vi "IonicsServiceTool.vi"() -> ()   [LabVIEW 2018]
uses:
  Type/_Source Type.ctl
  Type/_Syringe Pump Command.ctl
  Type/_Instrument Model.ctl
  Type/_RT Instrument State.ctl
  Type/_Run State.ctl
  Type/_Log Command.ctl
  Type/_RT Command.ctl
  Type/_RT Configuration 2.ctl
  Type/_PIC Channel.ctl
  Type/_RT Startup Options.ctl
  Type/_RT Instrument 2.ctl
  Type/_Data Operation.ctl
  Type/_Model Family.ctl
  Type/_SaveOption.ctl
  Type/_Board ID.ctl
  Type/_Run Module.ctl
  Type/_Voltage Type.ctl
  Print.ctl
  Type/_Pump Parameter.ctl
  Configuration/_Global Configuration.vi
  <vilib>/Utility/config.llb/Read Key (Path).vi
  <vilib>/Utility/config.llb/Write Key (Path).vi
  <vilib>/Utility/config.llb/Read Key (String).vi
  <vilib>/Utility/config.llb/Write Key (String).vi
  LCDriver/_Global LC Driver.vi
  <vilib>/Utility/config.llb/Read Key (I32).vi
  <vilib>/Utility/NIReport.llb/Append Image to Report (path wrap).vi
  <vilib>/Platform/browser.llb/Open URL in Default Browser (string).vi
  <vilib>/Utility/config.llb/Write Key (I32).vi
  <vilib>/Utility/NIReport.llb/NI_report.lvclass
  <vilib>/Utility/config.llb/NI_LVConfig.lvlib
panel:
  in  "Force Update Oscillators":bool
  out "Version":string
  out "Date/Time":string
  out "SN":string
  in  "Force Update Poles":bool
  out "MS State":T1
  in  "Print":bool
  in  "Options":bool
  in  "Unit":bool
  out "Firmware OK":bool
  out "Intlk/Per OK":bool
  out "Quad/Tune OK":bool=TRUE
  out "SVG OK":bool
  out "Voltage OK":bool
  out "Turbo OK":bool
  in  "Tab Control":T2(tab)
  out "*.ipf Path:":path=path "C:/GIT/EH-Simplicity/firmware-server/Sniffer.900/Ionica Server.ipf"
  in  "Header Info":bool
  out "IP Address":string="172.16.0.2"
  out "Corona":u16
  out "Source 2":u16
  out "Source 1":u16
  out "HSID":u16
  out "Model Name":T3=enum."Simulation (Single Source)"
  out "Serial Number":string="Ion Sniffer 03"
  in  "Refresh":bool
  out "Messages":string
  out "Description":string
  in  "Load Firmware":bool
  out "Current Information:":string[][](table)=[["FW Package Version", "0"], ["RT Firmware Version", "0"], ["FPGA Firmware Version", "0"], ["", ""], ["Instrument Serial #", "-1"], ["Instrument Model", "-1"]]
  out "Number of Power Failures:":u32
  out "Number of Pressure Overload Errors:":u32
  out "Total Number of Errors:":u32
  out "Errors:":string[][](table)=[["0", ""], ["", ""], ["", ""], ["", ""], ["", ""], ["", ""], ["", ""], ["", ""]]
  out "PumpStatus":u16(ring)
  out "Turning":bool
  out "Normal \nOperation":bool
  out "Accel":bool
  out "Decel":bool
  out "Frequency (Hz):":u16(slide) scale=0.0..1000.0
  out "Controller Temperature:":u16(slide) scale=0.0..90.0
  out "Moter Temperature:":u32(slide) scale=0.0..120.0
  out "Bearing Temperature:":u32(slide) scale=0.0..75.0
  out "Pressures:":string[][](table)=[["Foreline Pressure (torr)", "-0.11"], ["Analyzer Pressure (torr)", "1.00E+0"]]
  out "Run Time:":string[][](table)=[["Pump (hours)", ""], ["Days", ""], ["Number of Starts", ""], ["", ""], ["", ""], ["", ""], ["", ""], ["", ""]]
  out "Power:":string[][](table)=[["Voltage (V)", ""], ["Power (W)", ""], ["Current (A)", ""], ["Mean Current (A)", ""], ["Max Current (A)", ""], ["", ""], ["", ""], ["", ""]]
  out "Configuration:":string[][](table)=[["Pump Model", ""], ["Pump Serial Number", ""], ["Controller Model", ""], ["Controller Serial Number", ""], ["Electronics Model", ""], ["Electronic Serial Number", ""], ["Software Version", ""], ["Pump Parameter Set", ""]]
  in  "LBPower":bool
  in  "LBRunTime":bool
  in  "LBError":bool
  in  "LBConfiguration":bool
  in  "LBFreqTemp":bool
  in  "LBUpdateAll":bool
  in  "LBPump":bool
  in  "Update Power":bool
  in  "Update Temp":bool
  in  "Update Pumping":bool
  in  "Update Info":bool
  out "Error History":string[][](table)
  out "Temperatures:":string[][](table)=[["Electronic Drive Temperature", "Pass"], ["Pump Temperature", "Pass"], ["Power Stage Temperature (°C)", "0"], ["Electronics Temperature (°C)", "0"], ["Upper Pump Temperature (°C)", "0"], ["Bearing Temperature (°C)", "0"], ["Motor Temperature (°C)", "0"]]
  out "Power / Current:":string[][](table)=[["Drive Power (W)", "0"], ["Drive Current (A)", "0"]]
  out "Pumping:":string[][](table)=[["Rotational Frequency (Hz)", "0"], ["Rotational Speed (rpm)", "0"]]
  out "Pump Info:":string[][](table)=[["Hardware Version", "0"], ["Firmware Version", "0"], ["Operating Hours (Pump)", "0"], ["Operating Hours (Electronic Drive)", "0"]]
  in  "Turbo Update":bool
  out "Vacuum Readings by Region":string[][](table)=[["Foreline Pressure (torr)", "-0.11"], ["Analyzer Pressure (torr)", "1.00E+0"]]
  in  "Update Error":bool
  out "Main System Current (A)":dbl
  out "Lens Board 2 PS":i32(listbox)=-1
  in  "Set 0 Values":bool
  in  "Load Default Method":bool
  in  "Load Tune File":bool
  in  "Min Voltages":bool
  in  "Max Voltages":bool
  in  "Test Voltages":bool
  in  "Switch Polarity":bool
  out "Main System PS":i32(listbox)=-1
  out "Quad DC PS":i32(listbox)=-1
  out "Lens Board 1 PS":i32(listbox)=-1
  in  "Detector":string[][](table)=[["HED", "", "0.0", "3.014"], ["Horn", "", "0.0", "0.019"], ["DV", "", "0.0", "0.023"], ["Disc", "", "0.0", "2.014"], ["5", "L2 (11)", "0.0", "0.019"], ["6", "PF (12)", "-16.0", "0.019"], ["7", "CCL1 (13)", "0.0", "0.019"], ["8", "CCL2 (14)", "-100.0", "0.019"], ["9", "CC (23)", "-50.0", "0.014"], ["10", "CCAF (10)", "50.0", "0.019"], ["11", "CCL3 (15)", "-52.5", "0.014"], ["12", "CCL4 (16)", "-72.5", "0.014"], ["13", "ID (17)", "-100.0", "0.014"], ["14", "Horn (200)", "5500.0", "-82.090"], ["15", "DV (34)", "1000.0", "-82.773"], ["16", "M1RF (3)", "400.0", "2.161"], ["17", "Disc (32)", "10", "10"]]
  in  "Lens 1":string[][](table)=[["Element", "L1", "M1", "EV", "Spare", "M2", "CC", "Spare", "Spare"], ["Input", "0", "0", "0", "0", "0", "0", "0", "0"], ["Readback", "0", "0", "0", "0", "0", "0", "0", "0"]]
  in  "Lens 2":string[][](table)=[["Element", "CCAF", "L2", "PF", "CCL1", "CCL2", "CCL3", "CCL4", "ID"], ["Input", "", "", "", "", "", "", "", ""], ["Readback", "", "", "", "", "", "", "", ""]]
  out "Source Map":T4={"Ring 2"=0, "Ring 3"=0, "OK 2"=TRUE, "OK 3"=TRUE, "OK 4"=TRUE, "OK 5"=TRUE, "OK 6"=TRUE, "OK 7"=TRUE, "OK 8"=TRUE, "OK 9"=TRUE, "OK 10"=TRUE, "OK 11"=TRUE}
  out "Pressure Readings":string[][](table)=[["Foreline Pressure (torr)", "-0.11"], ["Analyzer Pressure (torr)", "1.00E+0"], ["Plenum Delta P (torr)", "-0.09"], ["Drying Gas Pressure (psi)", "-12.56"], ["Source Gas Pressure (psi)", "-12.56"]]
  in  "Corona/Curtain High Voltage":string[][](table)=[["Corona High Voltage", "0.0", "65535.000", "0"], ["Curtain Cap Voltage", "0.0", "910936.500", "0"]]
  in  "Source Probes":string[][](table)=[["Pillar 1", "None", "0.0", "2791790.869", "0"], ["Pillar 2", "None", "0.0", "2794412.334", "0"]]
  in  "Heaters":string[][](table)=[["1", "HSID", "200.0", "65535.000"], ["2", "P1T", "0.0", "93715.050"], ["3", "P2T", "0.0", "93715.050"]]
  in  "Typical Gas Settings":bool
  in  "Max Gas Settings":bool
  in  "Min Gas Settings":bool
  in  "Gas Flows":string[][](table)=[["1", "DG", "150.0", "316.460"], ["2", "NG1", "200.0", "312.782"], ["3", "HG1", "280.0", "354.817"], ["4", "NG2", "200.0", "0.000"], ["5", "HG2", "280.0", "0.000"], ["6", "CCP", "490", "-477.539"]]
  in  "GotoUPS":bool
  in  "IP Address":string
  in  "Input Value":sgl
  in  "Pump Command":T5=enum."status"
  out "Return Data":string
  in  "SendSyringeCommand":bool
  out "SourceOK":bool
  out "HG2OK":bool
  out "HG1OK":bool
  out "ExhaustOK":bool
  out "DryingGasOK":bool
  out "VacRdy":bool
  out "DoorOK":bool=TRUE
  out "Interlocks":string[][](table)=[["Card Cage Door", ""], ["Vacuum Ready", ""], ["Heating Gas 1", ""], ["Heating Gas 2", ""], ["Drying Gas", ""], ["Exhaust Gas", ""], ["Source Interlock", ""]]
  out "Source 2 Type:":T6=127 items=["None", "ESI", "APCI", "APPI", "MicroSpray"]
  out "Source 1 Type:":T6=127 items=["None", "ESI", "APCI", "APPI", "MicroSpray"]
  in  "FrequencyTuneSetup":bool
  out "Q2 RF Heat Sink Temperatures":string[][](table)=[["Q2 HS1", "-0.481"], ["Q2 HS2", "-0.481"], ["Q2 DC Pole A (18)", "-0.481"], ["Q2 DC Pole B (19)", "-0.481"]]
  out "Q1 RF Heat Sink Temperatures":string[][](table)=[["Q1 HS1", "-0.481"], ["Q1 HS2", "-0.481"], ["Q2 DC Pole A (18)", "-0.481"], ["Q2 DC Pole B (19)", "-0.481"]]
  out "M1 RF Heat Sink Temperatures":string[][](table)=[["M1 HS1", "-0.481"], ["M1 HS2", "-0.481"], ["Q2 DC Pole A (18)", "-0.481"], ["Q2 DC Pole B (19)", "-0.481"]]
  out "New Frequence":dbl=1.1064999969676137 format="%.4f"
  out "Old Frequency":dbl=1.1064999969676137 format="%.4f"
  in  "Adjust Cal Tables":bool
  out "M1RF Readback":dbl
  in  "M1RF":dbl=400.0 format="%#.3f"
  in  "Update PM":bool
  in  "Q2 Park Mass":dbl=400.0 format="%#.3f"
  in  "Q1 Park Mass":dbl=400.0 format="%#.3f"
  out "Q2 Total":dbl=157.94015025000002
  out "Q1 Total":dbl=157.94015025000002
  out "Q2 (VDC)":dbl=157.94015025000002
  out "Q1 (VDC)":dbl=157.94015025000002
  in  "Q2 DC Inputs":string[][](table)=[["600.00"], ["0.00"], ["0.00"]]
  in  "Q1 DC Inputs":string[][](table)=[["600.00"], ["0.00"], ["0.00"]]
  out "DC Pole Read Back":string[][](table)=[["Q1 DC Pole A", "-0.481"], ["Q1 DC Pole B", "-0.481"], ["Q2 DC Pole A", "-0.481"], ["Q2 DC Pole B", "-0.481"]]
  in  "Oscillator Settings":string[][](table)=[["M1RF", "66529043", "10", "10", "0.4", "1.5490", "2.256", "1.5490"], ["Q1RF", "47523813", "10", "10", "0.6", "1.1065", "-0.645", "1.1065"], ["Q2RF", "47523813", "10", "10", "0.6", "1.1065", "7.339", "1.1065"]]
  in  "Pos/Neg":enum32{"Positive", "Negative"}(radio)
  in  "Pole Swap Options Negative":T7
  in  "Pole Swap Options Positive":T7
  in  "Table Choice":T8(radio)
  out "Table 4":T9 caption="Q2 -ve Mass Calibration Table"
  out "Table 2":T9 caption="Q2 +ve Mass Calibration Table"
  out "Table 3":T9 caption="Q1 -ve Mass Calibration Table"
  out "Table 1":T9 caption="Q1 +ve Mass Calibration Table"
  in  "Edit Config":bool
  in  "Edit ADC":bool
  in  "View Config":bool
  in  "Export ADC":bool
  out "ADC List":i32(listbox)=130
  in  "Run":bool
  in  "Cancel":bool
  out "Progress Bar":u8(slide)=1 scale=0.0..100.0
  out "LoadedTable":bool
  in  "Tune File":path=path "C:/GIT/EH-Simplicity/firmware-server/Sniffer.900/InternalTools/DEFAULT_SETTINGS.d2m"
  in  "SG Input":dbl[](array[numeric])=[40.0, 0.0, 0.0, 0.0, 0.0, 0.0, 0.0, 200.0, 0.0, 0.0, 0.0, 0.0, 0.0, 0.0]
  in  "VoltageInput":dbl[](array[numeric])=[0.0, 0.0, 0.0, 0.0, 0.0, -16.0, 0.0, -100.0, -50.0, 50.0, -52.5, -72.5, -100.0, 5500.0, 1000.0, 400.0, 10.0, 0.0, 0.0]
  out "Quit":bool=TRUE
  out "Running":bool
  out "Ion Path":T10={"OK 1"=TRUE, "OK 2"=TRUE, "OK 3"=TRUE, "OK 4"=TRUE, "OK 5"=TRUE, "OK 6"=TRUE, "OK 7"=TRUE, "OK 8"=TRUE, "OK 9"=TRUE, "OK 10"=TRUE, "OK 15"=TRUE, "OK 20"=TRUE, "OK 16"=TRUE, "OK 11"=TRUE, "OK 17"=TRUE, "OK 18"=TRUE, "OK 19"=TRUE, "OK 12"=TRUE, "OK 13"=TRUE, "Selected 1"="Selected", "Selected 2"="Selected", "Selected 3"="Selected", "Selected 4"="Selected", "Selected 5"="Selected", "Selected 6"="Selected", "Selected 7"="Selected", "Selected 8"="Selected", "Selected 9"="Selected", "Selected 10"="Selected", "Selected 15"="Selected", "Selected 20"="Selected", "Selected 16"="Selected", "Selected 11"="Selected", "Selected 17"="Selected", "Selected 18"="Selected", "Selected 19"="Selected", "Selected 12"="Selected", "Selected 13"="Selected", "Ring 2"=0, "Ring 3"=0, "OK 14"=TRUE, "Selected 14"="Selected"}
  out "IonPathMap":enum32{"0", "200", "100"}(tab)
  # "PIC Firmware Version"
  # "It will take about 70s\nto complete Update All."
  # "Syringe Pump Control"
  # "UPS"
  # "V"
  # "Polarity"
  # "Pole Orientation"
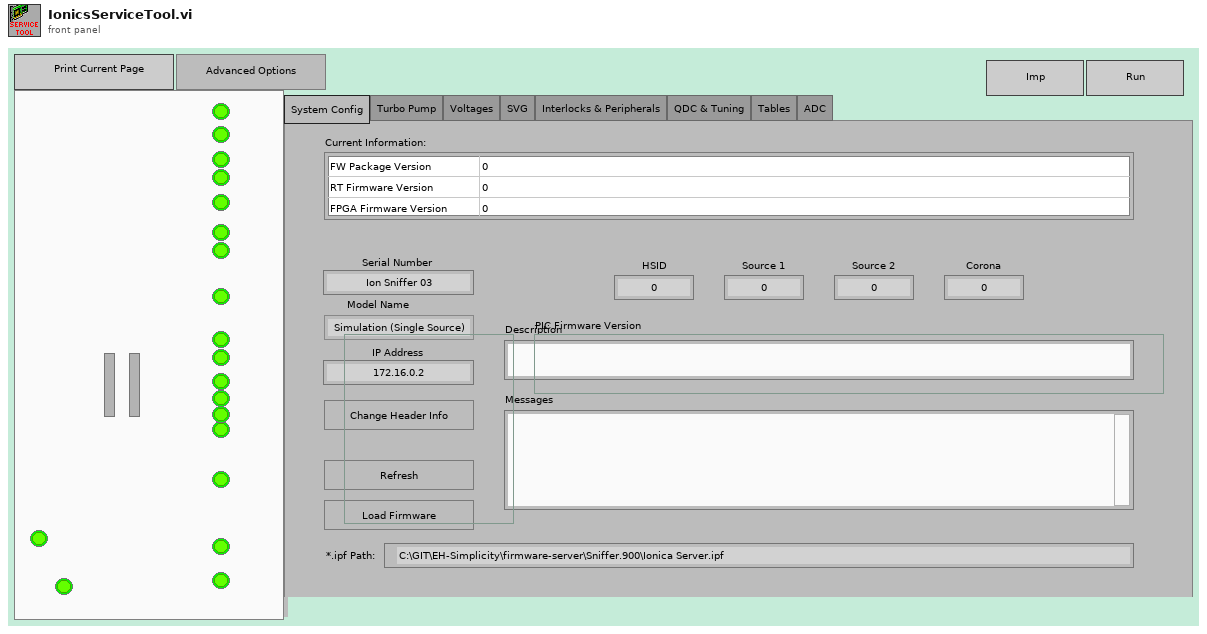
[diagram p1: front panel]
types:
  T1 = typedef "_RT Instrument State.ctl" = enum16{"Initializing", "Mass Spectrometer is Off", "Starting Up", "Turning Power Off", "Going to Standby", "Roughing Pump Ready", "Turning Turbo Off", "Turbo Startup", "Turbopump Ready", "Checking Vacuum", "Going to Ready", "Ready", "Running", "Source Standby", "Lost Communication", "Shutting Down", "Fault", "24V Standby", "Go to 24V Standby", "Turbopump Ready-Waiting"}
  T2 = enum32{"System Config", "Leybold 3QS", "Turbo Pump", "Voltages", "SVG", "Interlocks & Peripherals", "QDC & Tuning", "Tables", "ADC"}
  T3 = typedef "_Instrument Model.ctl" = enum16{"QSight 110", "QSight 120", "QSight 210", "QSight 220", "QSight 410", "QSight 420", "IONICS 3Q 110", "IONICS 3Q 120", "IONICS 3Q 210", "IONICS 3Q 220", "IONICS 3Q 310", "IONICS 3Q 320", "Simulation (Single Source)", "Simulation (Dual Source)"}
  T4 = cluster{"Ring 2":u16, "Ring 3":u16, "OK 2":bool, "OK 3":bool, "OK 4":bool, "OK 5":bool, "OK 6":bool, "OK 7":bool, "OK 8":bool, "OK 9":bool, "OK 10":bool, "OK 11":bool}
  T5 = typedef "_Syringe Pump Command.ctl" = enum16{"start", "stop", "pause", "restart", "help", "set units", "set diameter", "set rate", "set time", "set volume", "set delay", "save setting", "read limit parameter", "view parameter", "status"}
  T6 = typedef "_Source Type.ctl" = i8
  T7 = cluster{"Q1 A":bool, "Q1 B":bool, "Q2 A":bool, "Q2 B":bool}
  T8 = enum32{"Calibration", "Low Resolution", "Unit Resolution", "High Resolution"}
  T9 = cluster{"Graph":cluster{"all rows":dbl[], "all rows":dbl[]}, "Table":string[][]}
  T10 = cluster{"OK 1":bool, "OK 2":bool, "OK 3":bool, "OK 4":bool, "OK 5":bool, "OK 6":bool, "OK 7":bool, "OK 8":bool, "OK 9":bool, "OK 10":bool, "OK 15":bool, "OK 20":bool, "OK 16":bool, "OK 11":bool, "OK 17":bool, "OK 18":bool, "OK 19":bool, "OK 12":bool, "OK 13":bool, "Selected 1":string, "Selected 2":string, "Selected 3":string, "Selected 4":string, "Selected 5":string, "Selected 6":string, "Selected 7":string, "Selected 8":string, "Selected 9":string, "Selected 10":string, "Selected 15":string, "Selected 20":string, "Selected 16":string, "Selected 11":string, "Selected 17":string, "Selected 18":string, "Selected 19":string, "Selected 12":string, "Selected 13":string, "Ring 2":u16, "Ring 3":u16, "OK 14":bool, "Selected 14":string}
  T11 = enum32{"invalid app kind", "Development System", "Run Time System", "Student Edition", "Embedded LabVIEW", "Evaluation", "Custom"}
  T12 = enum8{"Enabled", "Disabled", "Disabled and Grayed Out"}
  T13 = typedef "_Run State.ctl" = enum16{"Init", "Update", "Start", "End", "Error"}
  T14 = typedef "_Log Command.ctl" = enum16{"No Command", "Open", "Read", "Write", "Close", "Check Size"}
  T15 = typedef "_RT Command.ctl" = enum16{"xml Start Run", "xml Start Actual Run", "xml Stop Run", "xml Runtime Update", "xml Get Status", "xml Get Table", "xml Set Table", "xml Get Configuration", "xml System Status", "xml Set LC Input Logic", "xml Get Data", "xml Get Info", "Start", "StartActualRun", "Stop", "Runtime Update", "Get Data", "Get Info", "Get Status", "Get Param", "Get Config", "Get Table", "Read ADC", "Set Oscillator", "Update Config", "Update Table", "Set All Pol", "Set Pol and DC", "Set Max Mass", "Toggle RP", "Toggle EL", "Set PIC", "Initialize Turbo", "Send Turbo Comm", "Close Turbo", "P1", "P2", "P3", "Send Serial", "Set LC Out", "Get LC In", "Read VAC", "Test Table", "Toggle Power", "Get Startup", "Set Startup", "Get ADC Table", "Set ADC Table", "Get Brief Status", "Get Detail Status", "Auxiliary Update", "Set CC Logics", "Test Channel", "Set CC Input Logics", "Ignore Error", "invalid"}
  T16 = enum16{"Use Dialog", "Temporary File", "My Tables"}
  T17 = typedef "_PIC Channel.ctl" = enum16{"Corona +HV", "Corona -HV", "HSID Temp", "Time Const 1", "Curtain Cap +HV", "Curtain Cap -HV", "Time Const 2", "Source 1 +HV", "Source 1 -HV", "Source 1 Temp", "Time Const 3", "Source 2 +HV", "Source 2 -HV", "Source 2 Temp", "Time Const 4"}
  T18 = typedef "_RT Instrument 2.ctl" = cluster{"Table":T19[], "Instrument":string[]}
  T19 = typedef "_RT Configuration 2.ctl" = cluster{"Name":string, "Ch#":u8, "Min":dbl, "Max":dbl, "Def+":dbl, "Def-":dbl, "Offset":dbl, "Slope":dbl, "Type":u8, "Description":string, "SettleT":dbl}
  T20 = cluster{"top":dbl, "left":dbl, "right":dbl, "bottom":dbl}
  T21 = typedef "Print.ctl" = cluster{"Picture Name":string, "VI Reference":refnum<vi>}
  T22 = enum16{"Standard Report", "HTML", "Word", "Excel"}
  T23 = typedef "_Data Operation.ctl" = enum8{"Initialize", "Get Data", "Set Data", "Close"}
  T24 = typedef "_SaveOption.ctl" = enum16{"Use Dialog", "Temporary File", "My Tables", "Full Path"}
  T25 = typedef "_Pump Parameter.ctl" = enum16{"Turn Pump Motor On", "Turn Pump Motor Off", "Read Pump Oil Deficiency", "Read Rotation Switch Point Attained", "Read Ele. Drive Over Temperature", "Read Pump Over Temperature", "Read Set Rotation Speed Attained", "Read Turbopump Accelerates", "Read Actual Rotation Speed in Hz", "Read Motor Current in A", "Read Operating Hours in h", "Read Motor Voltage in V", "Read Motor Power in W", "Set Rotation Speed Switchpoint in %", "Clear Error", "Read Error Code", "Read Bearing Temperature", "Read Hardware Version", "Read Firmware Version", "Read Operating Hours (Drive)", "Read Rotational Speed (rpm)", "Read Power Stage Temperature", "Read Electronics Temperature", "Read Upper Pump Temperature", "Read Motor Temperature", "Read Error Code History, 1", "Read Error Code History, 2", "Read Error Code History, 3", "Read Error Code History, 4", "Read Error Code History, 5", "Read Error Code History, 6", "Read Error Code History, 7", "Read Error Code History, 8", "Read Error Code History, 9", "Read Error Code History, 10"}
  T26 = enum32{"existing file", "new file", "new or existing file", "existing dir", "new dir", "new or existing dir", "existing file (use LLBs)", "new file (use LLBs)", "new or existing file (use LLBs)", "new or existing file or directory (use LLBs)"}
  T27 = enum32{"Leybold 3QS", "Pfeiffer Pump", "Voltages", "SVG", "Interlocks & Peripherals", "FW Manager", "QDC & Tuning", "Tables", "ADC"}
  T28 = cluster{"Source Map":refnum<vi>, "Ion Path":refnum<vi>, "Lens 1":refnum<vi>, "Lens 2":refnum<vi>, "Detector":refnum<vi>, "Main System PS":refnum<vi>, "Lens Board 1 PS":refnum<vi>, "Quad DC PS":refnum<vi>, "Gas Flows":refnum<vi>, "Heaters":refnum<vi>, "Source Probes":refnum<vi>, "Corona/Curtain High Voltage":refnum<vi>, "Pressure Readings":refnum<vi>, "DC Pole Read Back":refnum<vi>, "Lens Board 2 PS":refnum<vi>, "M1 RF Heat Sink Temperatures":refnum<vi>, "Q1 RF Heat Sink Temperatures":refnum<vi>, "Q2 RF Heat Sink Temperatures":refnum<vi>}
  T29 = typedef "NI_LVConfig.lvlib/Config Data RefNum.ctl" = refnum<k1>
  T30 = typedef "_LC Type.ctl" = enum16{"No LC", "Spark"}
  T31 = typedef "_RT Startup Options.ctl" = cluster{"Door":bool, "Curtain":bool, "Pressure":bool, "Turbo":bool, "SysPoll":bool, "GasFlag":bool, "SourceExhaust":bool}
  T32 = cluster{"Configuration 2":T18, "FrequencyTune":bool, "CalAjusted":bool, "Update":bool, "Running":bool, "ADC Table":T19[]}
  T33 = typedef "_Model Family.ctl" = u16
  T34 = typedef "_Board ID.ctl" = u16
  T35 = typedef "_Run Module.ctl" = u16
  T36 = cluster{"trimmed string":string, string, "selected path":path, "Source":enum32{"RT Target", "Folder"}}
  T37 = typedef "_Voltage Type.ctl" = u16
  T38 = cluster{"Frequency":u16, "Decel":bool, "Accel":bool, "Normal \nOperation":bool, "Turning":bool, "BearingTemp":u32, "MotorTemp":u32, "ControllerTemp":u16, "PumpStatus":u16, "NumErrors":u32, "NumOverload":u32, "NumFailure":u32}
  T39 = typedef "imagedata.ctl" = cluster{"image type":i32, "image depth":i32, "image":u8[], "mask":u8[], "colors":u32[], "Rectangle":cluster{"left":i16, "top":i16, "right":i16, "bottom":i16}}
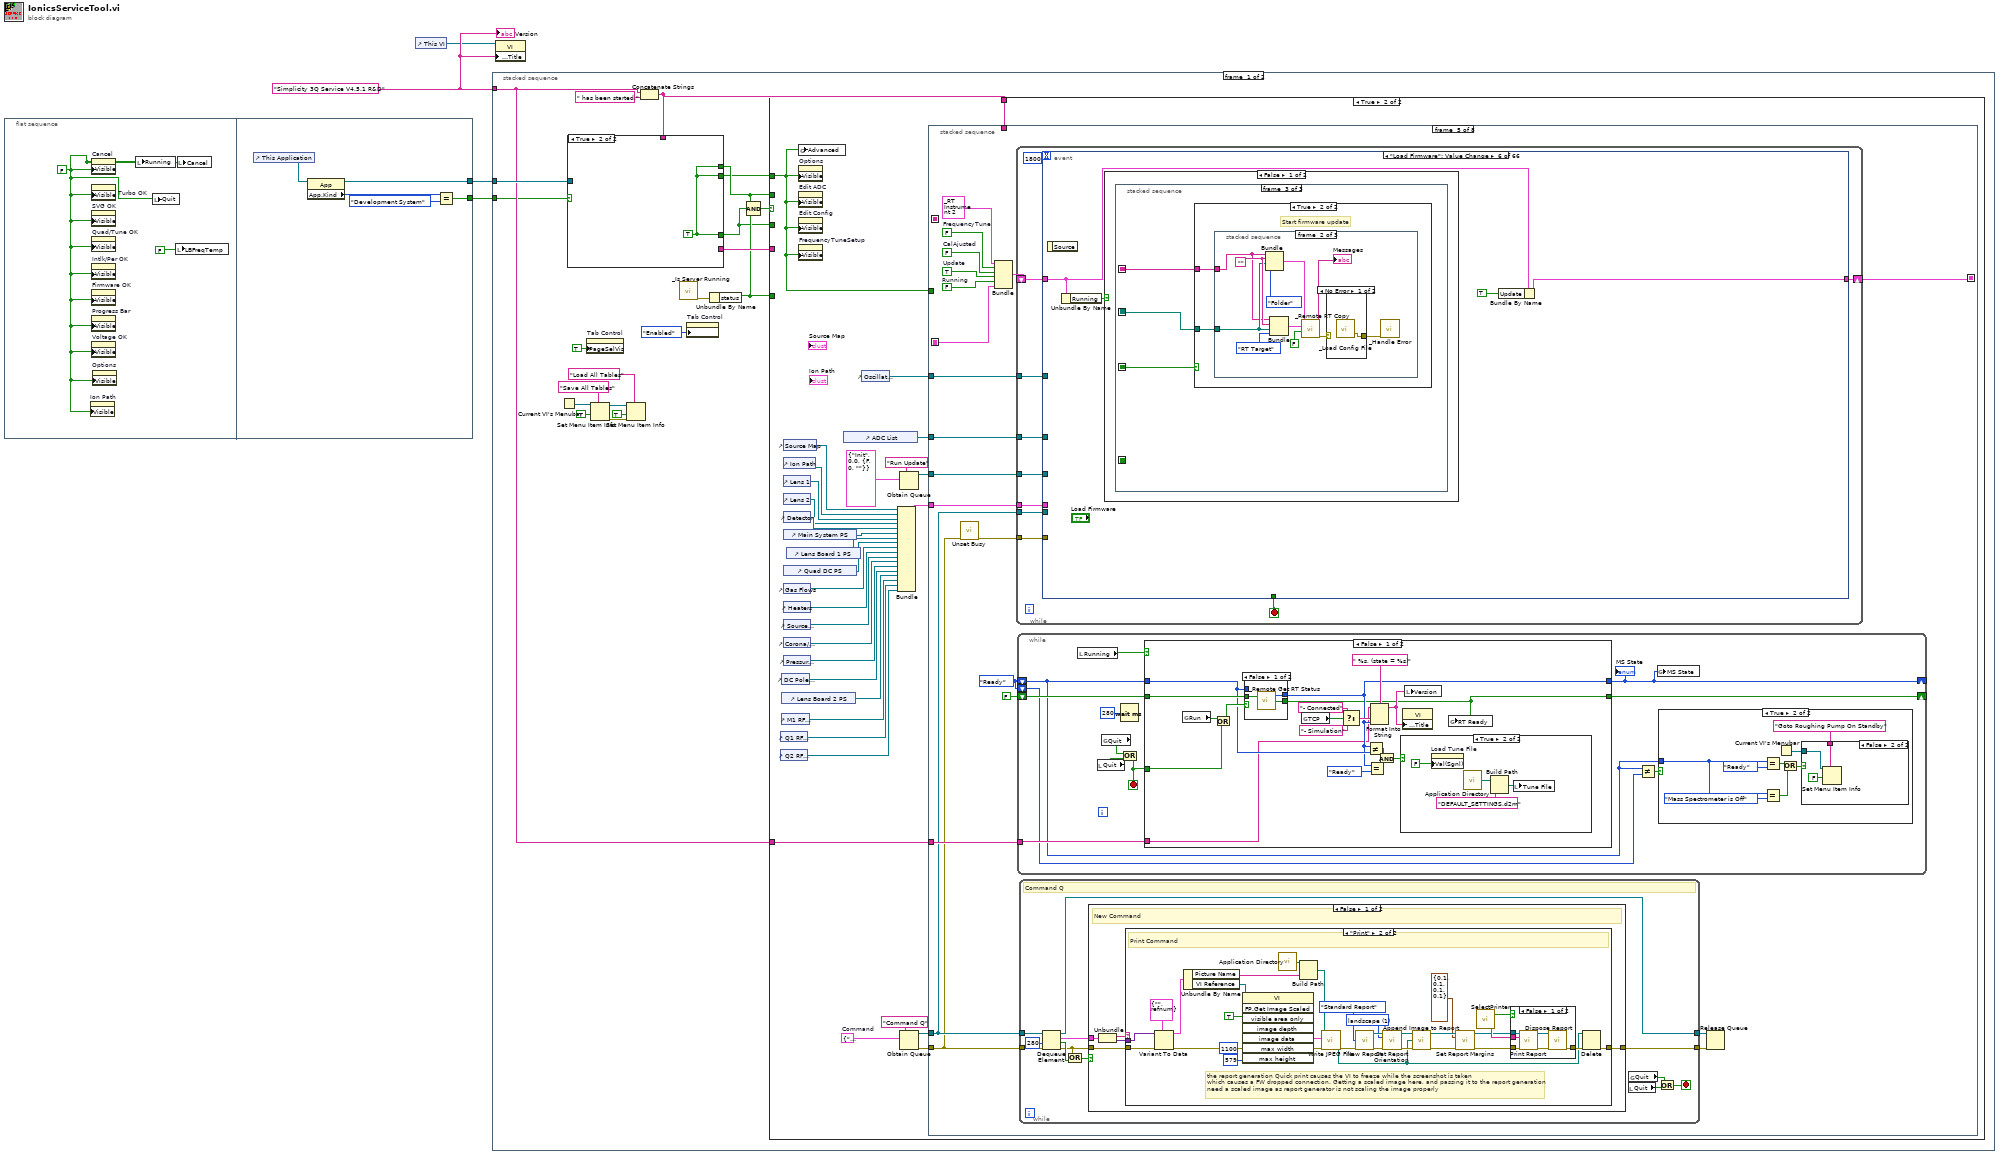
[diagram p0: block diagram]
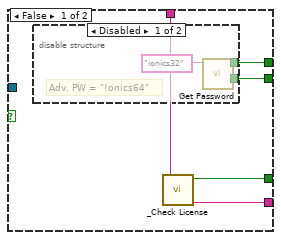
[diagram p2: hidden frame]
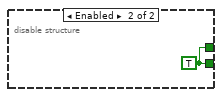
[diagram p3: hidden frame]
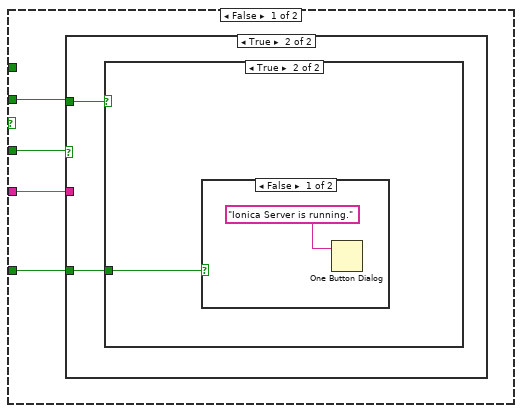
[diagram p4: hidden frame]
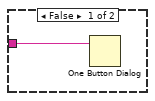
[diagram p5: hidden frame]
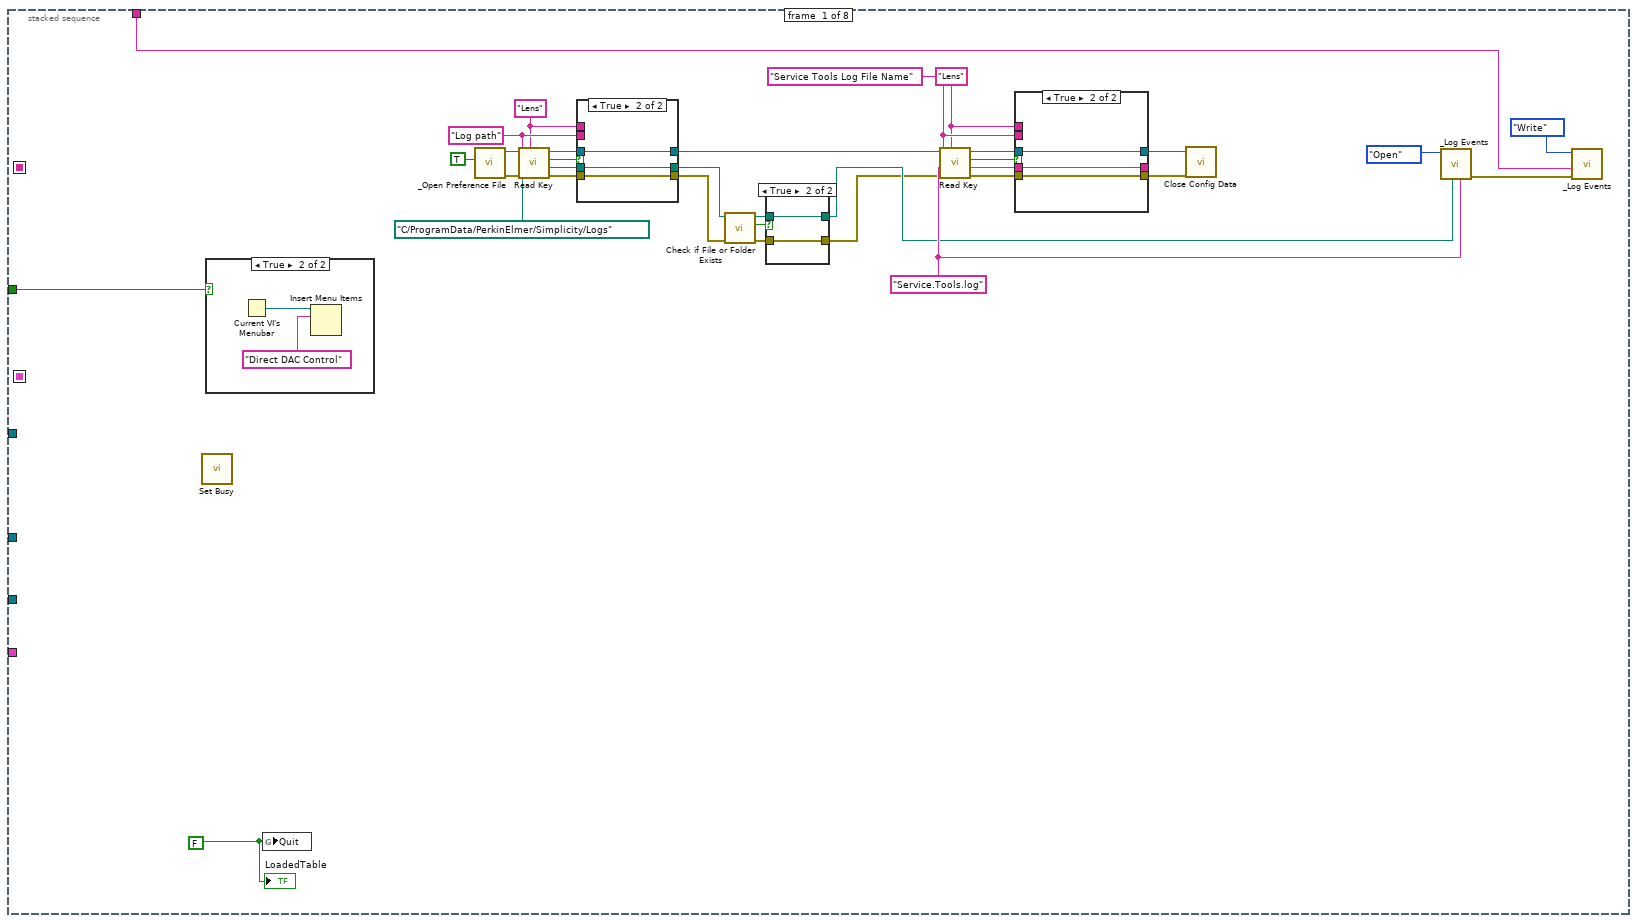
[diagram p8: hidden frame]
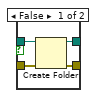
[diagram p9: hidden frame]
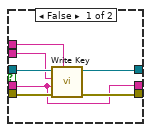
[diagram p10: hidden frame]
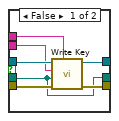
[diagram p11: hidden frame]
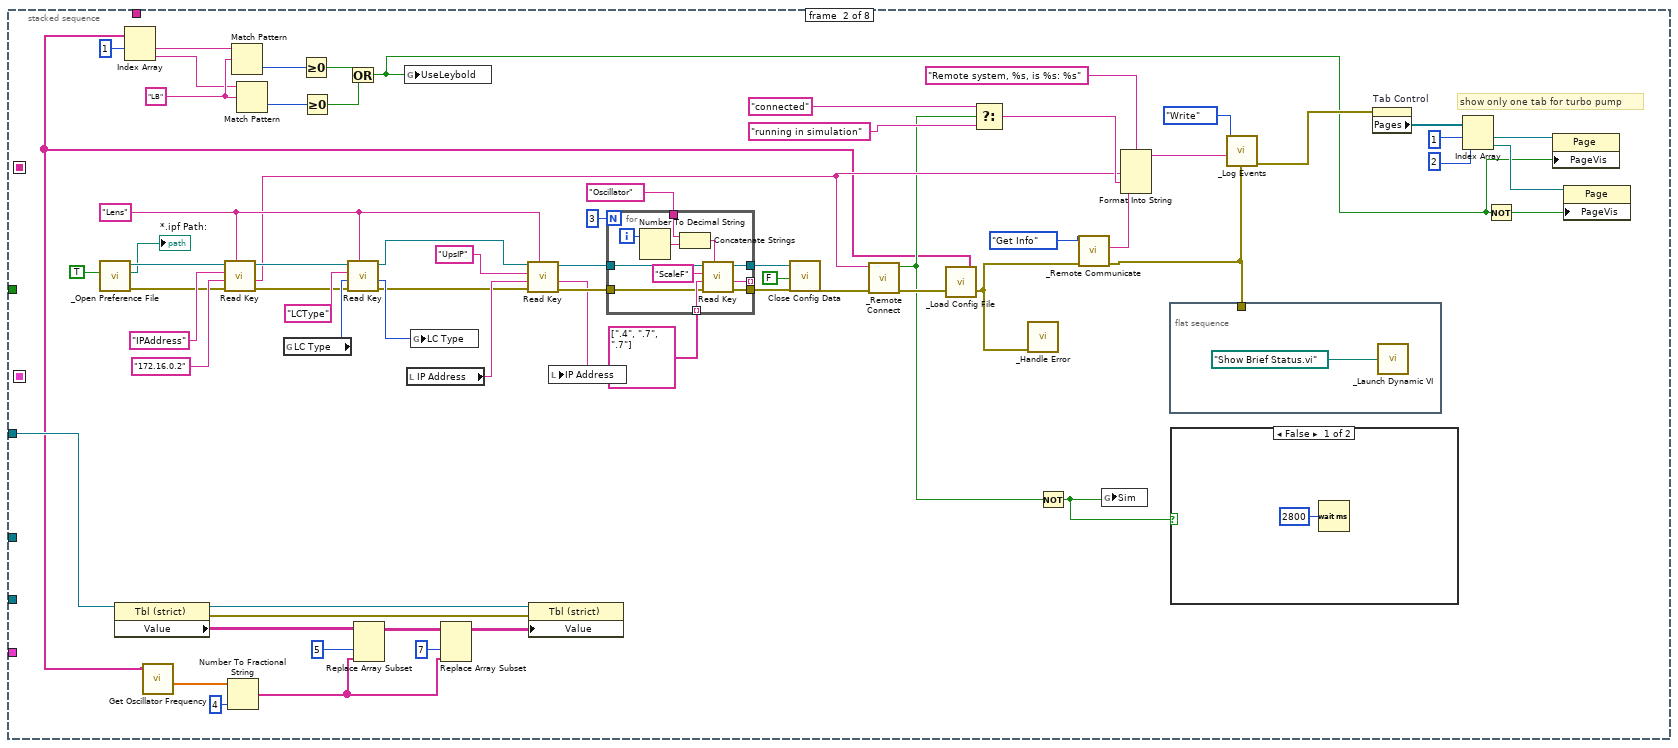
[diagram p13: hidden frame]
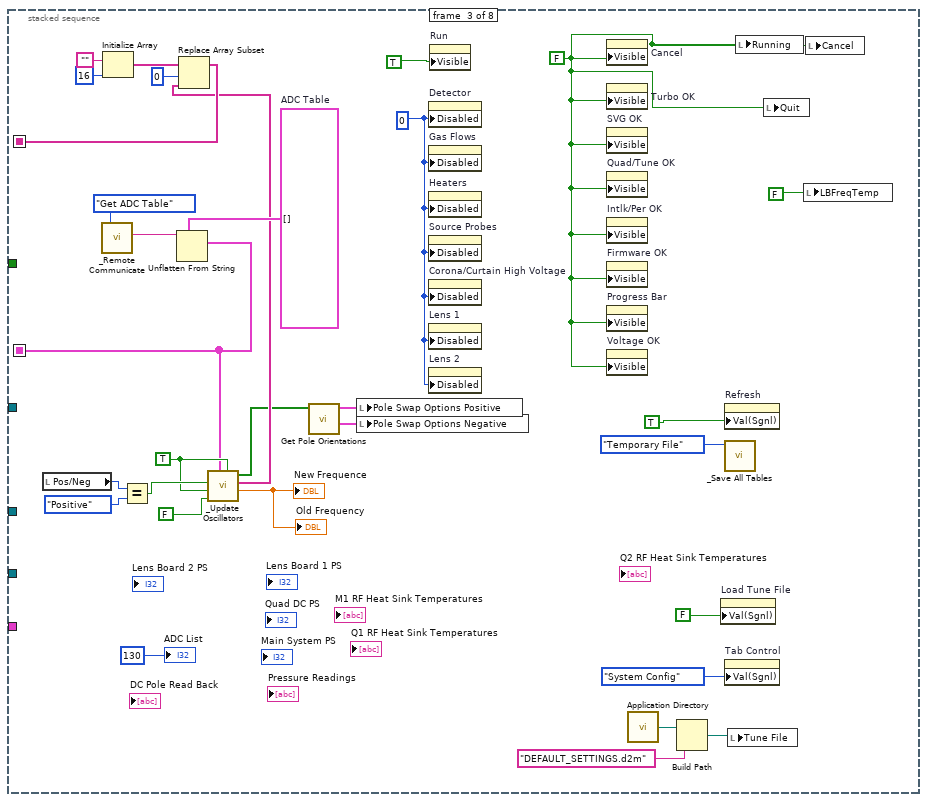
[diagram p15: hidden frame]
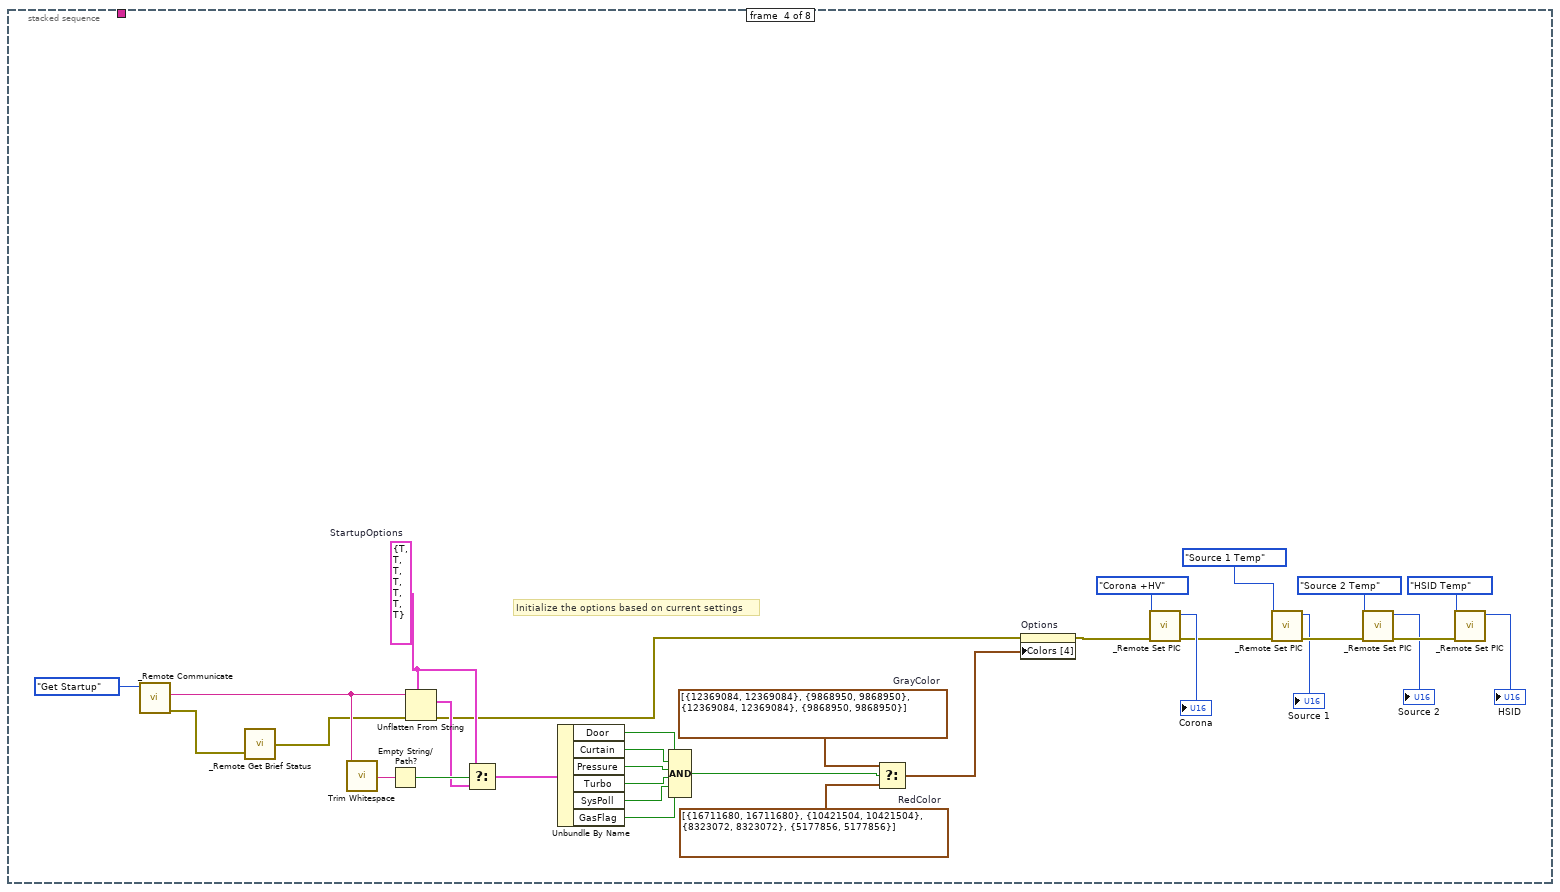
[diagram p16: hidden frame]
diagram:
  w2 = "Simplicity 3Q Service V4.5.1 R&D" ("string")
  n1 = flat-sequence {
    tunnel: [w9] -> w4
    tunnel: [w8] -> w3
    frame #0 {
      w5 = FALSE ("Unit")
      n2 = property on="Ion Path" class="Clust (strict)"("Visible"=w5) -> ()  [unwired: 2 in, 2 out]
      n3 = property on="Cancel" class="Bool (strict)"("Visible"=w5) -> ()  [unwired: 2 in, 2 out]
      n4 = property on="Turbo OK" class="Bool (strict)"("Visible"=w5) -> ()  [unwired: 2 in, 2 out]
      n5 = property on="SVG OK" class="Bool (strict)"("Visible"=w5) -> ()  [unwired: 2 in, 2 out]
      n6 = property on="Quad/Tune OK" class="Bool (strict)"("Visible"=w5) -> ()  [unwired: 2 in, 2 out]
      n7 = property on="Intlk/Per OK" class="Bool (strict)"("Visible"=w5) -> ()  [unwired: 2 in, 2 out]
      n8 = property on="Firmware OK" class="Bool (strict)"("Visible"=w5) -> ()  [unwired: 2 in, 2 out]
      n9 = property on="Progress Bar" class="Slide (strict)"("Visible"=w5) -> ()  [unwired: 2 in, 2 out]
      n10 = property on="Voltage OK" class="Bool (strict)"("Visible"=w5) -> ()  [unwired: 2 in, 2 out]
      n11 = property on="Options" class="Bool"("Visible"=w5) -> ()  [unwired: 2 in, 2 out]
      n12 = local write "Running"(w5) -> ()
      n13 = local write "Quit"(w5) -> ()
      n14 = local write "LBFreqTemp"(FALSE ("LBFreqTemp")) -> ()
      n15 = local write "Cancel"(w5) -> ()
    }
    frame #1 {
      n16 = control-ref of="This Application"() -> (w7:refnum<vi>)
      n17 = property class="App"(reference=w7) -> (reference out=w8:refnum<vi>, "App.Kind"=w10:T11)  [unwired: 1 in, 1 out]
      n18 = Equal?(x=w10, y=T11."Development System") -> (x = y?=w9:bool)
    }
  }
  n19 = control-ref of="This VI"() -> (w1:refnum<vi>)
  n20 = stacked-sequence {
    tunnel: w4 -> [w12 w1754]
    tunnel: w3 -> [w25 _]
    tunnel: w2 -> [w22 _]
    frame #0 {
      n21 = Current VI's Menubar() -> (w19:refnum<k9>)
      n22 = property on="Tab Control" class="TabCtl (strict)"("PageSelVis"=TRUE ("Page Selector Visible")) -> ()  [unwired: 2 in, 2 out]
      n23 = Set Menu Item Info(7:"Save All Tables" ("item tag"), 9:TRUE ("enabled"), 11:w19) -> (0:w15:errorcluster, 3:w16:refnum<k9>)  [unwired: 4 in]
      n24 = Set Menu Item Info(7:"Load All Tables" ("item tag"), 8:w15, 9:TRUE ("enabled"), 11:w16) -> ()  [unwired: 3 in, 2 out]
      n25 = Concatenate Strings(w22, " has been started." ("string")) -> (w24:string)
      n26 = case shown="True" w12 {
        tunnel: w24 -> [w37 _]
        tunnel: [w36 _] -> w31
        tunnel: [w35 w42] -> w30
        tunnel: [w34 w42] -> w29
        tunnel: [w33 w42] -> w26
        tunnel: w25 -> [_ _]
        frame False {
          n27 = disable-structure shown="Disabled" {
            disable-tunnel: [w39 w41] -> w35
            disable-tunnel: [w38 w41] -> w34
            frame Disabled {
              # "Adv. PW = \"!onics64\""
              n28 = call "Get Password.vi"("IonSniffer777"="ionics32") -> ("Advanced"=w38:bool, "Valid"=w39:bool)  [unwired: 5 out]
            }
            frame Enabled {
              w41 = TRUE ("Advanced")
            }
          }
          n29 = call "_Check License.vi"("ApplicationName"=w37) -> ("Reason"=w36:string, "Valid"=w33:bool)  [unwired: 5 out]
        }
        frame True {
          w42 = TRUE ("Valid")
        }
      }
      n30 = call "_Is Server Running.vi"() -> ("error out"=w28:errorcluster)  [unwired: 6 in, 1 out]
      n31 = property on="Tab Control" class="TabCtl (strict)"("DisabledEnum"=T12."Enabled" ("Disabled")) -> ()  [unwired: 2 in, 2 out]
      n32 = Unbundle By Name(w28) -> ("status"=w27:bool)
      n33 = Compound Arithmetic op=AND(w30, w26, w27) -> (w32:bool)
      n34 = case shown="True" w32 {
        tunnel: w24 -> [_ w66]
        tunnel: w26 -> [w46 _]
        tunnel: w31 -> [w45 _]
        tunnel: w30 -> [w44 _]
        tunnel: w29 -> [_ w57]
        tunnel: w27 -> [w43 _]
        tunnel: w22 -> [_ w56]
        frame False {
          n35 = case shown="True" w46 {
            tunnel: w45 -> [w47 _]
            tunnel: w44 -> [_ w49]
            tunnel: w43 -> [_ w48]
            frame False {
              n36 = One Button Dialog(message=w47) -> ()  [unwired: 2 out]
            }
            frame True {
              n37 = case shown="True" w49 {
                tunnel: w48 -> [_ w50]
                frame False {
                }
                frame True {
                  n38 = case shown="False" w50 {
                    frame False {
                      n39 = One Button Dialog(message="Ionica Server is running.") -> ()  [unwired: 2 out]
                    }
                    frame True {
                    }
                  }
                }
              }
            }
          }
        }
        frame True {
          w54 = cluster{"Command":string, "Data":variant} {"Command"="", "Data"=variant}  # Command
          n40 = control-ref of="Q1 RF Heat Sink Temperatures"() -> (w59:refnum<vi>)
          n41 = control-ref of="Q2 RF Heat Sink Temperatures"() -> (w58:refnum<vi>)
          n42 = control-ref of="Lens Board 2 PS"() -> (w61:refnum<vi>)
          n43 = control-ref of="DC Pole Read Back"() -> (w67:refnum<vi>)
          n44 = control-ref of="M1 RF Heat Sink Temperatures"() -> (w60:refnum<vi>)
          n45 = control-ref of="Ion Path"() -> (w63:refnum<vi>)
          n46 = control-ref of="Lens 1"() -> (w64:refnum<vi>)
          n47 = control-ref of="Lens 2"() -> (w65:refnum<vi>)
          n48 = control-ref of="Detector"() -> (w79:refnum<vi>)
          n49 = control-ref of="Main System PS"() -> (w78:refnum<vi>)
          n50 = control-ref of="Quad DC PS"() -> (w77:refnum<vi>)
          n51 = control-ref of="Gas Flows"() -> (w73:refnum<vi>)
          n52 = control-ref of="Heaters"() -> (w72:refnum<vi>)
          n53 = control-ref of="Source Probes"() -> (w71:refnum<vi>)
          n54 = control-ref of="Corona/Curtain High Voltage"() -> (w70:refnum<vi>)
          n55 = control-ref of="Pressure Readings"() -> (w69:refnum<vi>)
          n56 = control-ref of="Source Map"() -> (w62:refnum<vi>)
          n57 = control-ref of="Lens Board 1 PS"() -> (w76:refnum<vi>)
          n58 = global write "_Global Configuration.vi" "Advanced"(w57) -> ()
          n59 = property on="Options" class="Bool"("Visible"=w57) -> ()  [unwired: 2 in, 2 out]
          n60 = property on="Edit ADC" class="Bool"("Visible"=w57) -> ()  [unwired: 2 in, 2 out]
          n61 = property on="Edit Config" class="Bool"("Visible"=w57) -> ()  [unwired: 2 in, 2 out]
          n62 = property on="FrequencyTuneSetup" class="Bool (strict)"("Visible"=w57) -> ()  [unwired: 2 in, 2 out]
          n63 = control-ref of="ADC List"() -> (w74:refnum<vi>)
          n64 = control-ref of="Oscillator Settings"() -> (w68:refnum<vi>)
          n65 = Bundle("Source Map"=w62, "Ion Path"=w63, "Lens 1"=w64, "Lens 2"=w65, "Detector"=w79, "Main System PS"=w78, "Lens Board 1 PS"=w76, "Quad DC PS"=w77, "Gas Flows"=w73, "Heaters"=w72, "Source Probes"=w71, "Corona/Curtain High Voltage"=w70, "Pressure Readings"=w69, "DC Pole Read Back"=w67, "Lens Board 2 PS"=w61, "M1 RF Heat Sink Temperatures"=w60, "Q1 RF Heat Sink Temperatures"=w59, "Q2 RF Heat Sink Temperatures"=w58) -> (w75:T28)  [unwired: 1 out]
          n66 = Obtain Queue(name (unnamed)="Run Update", element data type=cluster{T13, dbl, "error out":errorcluster} {enum."Init", 0.0, "error out"={"status"=FALSE, "code"=0, "source"=""}}) -> (queue out=w80:refnum<queue>)  [unwired: 3 in, 2 out]
          n67 = Obtain Queue(name (unnamed)="Command Q", element data type=w54) -> (queue out=w53:refnum<queue>, error out=w52:errorcluster)  [unwired: 3 in, 1 out]
          n68 = stacked-sequence {
            seq-local: [_ _ w227 _ _ _ _ _] -> [_ _ _ _ w299 _ _ _]
            seq-local: [_ _ w232 _ _ _ _ _] -> [_ _ _ _ _ w1643 _ _]
            seq-local: [_ _ _ _ w297 _ _ _] -> [_ _ _ _ _ w1646 _ _]
            tunnel: w80 -> [_ _ _ _ w307 w1700 _ _]
            tunnel: w75 -> [_ _ _ _ w303 _ _ _]
            tunnel: w74 -> [_ _ _ _ w302 _ _ _]
            tunnel: w68 -> [_ w171 _ _ w301 _ _ _]
            tunnel: w66 -> [w83 _ _ _ _ _ _ _]
            tunnel: w57 -> [w114 _ _ _ _ _ _ _]
            tunnel: w56 -> [_ _ _ _ w294 _ _ _]
            tunnel: w53 -> [_ _ _ _ w293 _ _ _]
            tunnel: w52 -> [_ _ _ _ w290 _ _ _]
            frame #0 {
              w113 = "Service.Tools.log" ("default value")
              w103 = "Service Tools Log File Name" ("key")
              w102 = "Lens" ("section")
              w97 = "Log path" ("key")
              w96 = "Lens" ("section")
              w115 = FALSE ("Quit")
              n69 = call <vilib>:"Set Busy.vi"() -> ()  [unwired: 4 in, 8 out]
              n70 = case shown="True" w114 {
                frame False {
                }
                frame True {
                  n71 = Current VI's Menubar() -> (w143:refnum<k9>)
                  n72 = Insert Menu Items(8:"Direct DAC Control", 9:w143) -> ()  [unwired: 4 in, 3 out]
                }
              }
              n73 = global write "_Global Configuration.vi" "Quit"(w115) -> ()
              n74 = call "_Open Preference File.vi"("Initialize"=TRUE) -> ("error"=w89:errorcluster, "refnum"=w90:T29)  [unwired: 2 in, 3 out]
              n75 = call-poly <vilib>:"Read Key.vi"("section"=w96, "error in (no error)"=w89, "default value"=path "C:/ProgramData/PerkinElmer/Simplicity/Logs", "key"=w97, "refnum"=w90) -> ("error out"=w91:errorcluster, "value"=w93:path, "found?"=w92:bool, "refnum out"=w94:T29)  [unwired: 3 in]
              n76 = case shown="True" w92 {
                tunnel: w91 -> [w138 w141]
                tunnel: w93 -> [w132 w139]
                tunnel: w94 -> [w136 w140]
                tunnel: [w137 w141] -> w110
                tunnel: [w135 w140] -> w95
                tunnel: [w132 w139] -> w111
                tunnel: w96 -> [w134 _]
                tunnel: w97 -> [w133 _]
                frame False {
                  n77 = call-poly <vilib>:"Write Key.vi"("section"=w134, "error in (no error)"=w138, "value"=w132, "key"=w133, "refnum"=w136) -> ("error out"=w137:errorcluster, "refnum out"=w135:T29)  [unwired: 4 in, 1 out]
                }
                frame True {
                }
              }
              n78 = call <vilib>:"Check if File or Folder Exists.vi"("error in (no error)"=w110, "path"=w111) -> ("error out"=w106:errorcluster, "file or folder exists?"=w108:bool, "dup path"=w107:path)  [unwired: 7 in]
              n79 = case shown="True" w108 {
                tunnel: w106 -> [w119 w120]
                tunnel: w107 -> [w118 w121]
                tunnel: [w117 w121] -> w112
                tunnel: [w116 w120] -> w109
                frame False {
                  n80 = Create Folder(path (use dialog)=w118, error in=w119) -> (created path=w117:path, error out=w116:errorcluster)  [unwired: 1 in, 1 out]
                }
                frame True {
                }
              }
              n81 = call-poly <vilib>:"Read Key.vi"("section"=w102, "error in (no error)"=w109, "default value"=w113, "key"=w103, "refnum"=w95) -> ("error out"=w101:errorcluster, "value"=w100:string, "found?"=w99:bool, "refnum out"=w98:T29)  [unwired: 3 in]
              n82 = case shown="True" w99 {
                tunnel: w101 -> [w128 w131]
                tunnel: w100 -> [w122 w129]
                tunnel: w98 -> [w126 w130]
                tunnel: [w127 w131] -> w105
                tunnel: [w125 w130] -> w104
                tunnel: [w122 w129] -> _
                tunnel: w102 -> [w124 _]
                tunnel: w103 -> [w123 _]
                frame False {
                  n83 = call-poly <vilib>:"Write Key.vi"("section"=w124, "error in (no error)"=w128, "value"=w122, "key"=w123, "refnum"=w126) -> ("error out"=w127:errorcluster, "refnum out"=w125:T29)  [unwired: 4 in, 1 out]
                }
                frame True {
                }
              }
              n84 = call <vilib>:"Close Config Data.vi"("error in (no error)"=w105, "refnum"=w104) -> ()  [unwired: 1 in, 9 out]
              n85 = call "_Log Events.vi"("File Name"=w113, "Log Path"=w112, "Log Command"=_Log_Command."Open" ("File Command")) -> ("error out"=w86:errorcluster)  [unwired: 5 in, 1 out]
              n86 = call "_Log Events.vi"("error in (no error)"=w86, "Event"=w83, "Log Command"=_Log_Command."Write" ("File Command")) -> ()  [unwired: 5 in, 2 out]
              "LoadedTable" <- w115
            }
            frame #1 {
              w184 = "LB" ("regular expression")
              w189 = "Lens" ("section")
              # "show only one tab for turbo pump"
              n87 = call "_Open Preference File.vi"("Initialize"=TRUE) -> ("error"=w166:errorcluster, "ipf path"=→"*.ipf Path:":path, "refnum"=w198:T29)  [unwired: 2 in, 2 out]
              n88 = property class="Tbl (strict)"(reference=w171) -> (reference out=w172:refnum<vi>, error out=w144:errorcluster, "Value"=w173:string[][])  [unwired: 1 in]
              n89 = call-poly <vilib>:"Read Key.vi"("section"=w189, "error in (no error)"=w166, "default value"="172.16.0.2", "key"="IPAddress" ("section"), "refnum"=w198) -> ("error out"=w165:errorcluster, "value"=w154:string, "refnum out"=w195:T29)  [unwired: 1 in, 3 out]
              n90 = global read "_Global LC Driver.vi" "LC Type"() -> (w194:T30)
              n91 = call-poly <vilib>:"Read Key.vi"("section"=w189, "error in (no error)"=w165, "default value"=w194, "key"="LCType" ("section"), "refnum"=w195) -> ("error out"=w164:errorcluster, "value"=w192:i32, "refnum out"=w191:T29)  [unwired: 4 out]
              n92 = local read "IP Address"() -> (w188:string)
              n93 = global write "_Global LC Driver.vi" "LC Type"(w192) -> ()
              n94 = call-poly <vilib>:"Read Key.vi"("section"=w189, "error in (no error)"=w164, "default value"=w188, "key"="UpsIP" ("section"), "refnum"=w191) -> ("error out"=w158:errorcluster, "value"=w155:string, "refnum out"=w161:T29)  [unwired: 1 in, 3 out]
              n95 = local write "IP Address"(w155) -> ()
              n96 = for {
                N: 3 -> [_]
                tunnel: w161 -> [w223]
                tunnel: [w222] -> w157
                tunnel: "Oscillator" ("section") -> [w218]
                tunnel: string[] [".4", ".7", ".7"] ("key") -> [w216] mode=indexing
                tunnel: [w215] -> _ mode=indexing
                tunnel: w158 -> [w214]
                tunnel: [w213] -> w156
                i -> [w221]
                n97 = Number To Decimal String(number=w221) -> (decimal integer string=w220:string)  [unwired: 1 in]
                n98 = Concatenate Strings(w218, w220) -> (w219:string)
                n99 = call-poly <vilib>:"Read Key.vi"("section"=w219, "error in (no error)"=w214, "default value"=w216, "key"="ScaleF", "refnum"=w223) -> ("error out"=w213:errorcluster, "value"=w215:string, "refnum out"=w222:T29)  [unwired: 3 in, 1 out]
              }
              n100 = call <vilib>:"Close Config Data.vi"("error in (no error)"=w156, "write file if changed (T)"=FALSE ("write configuration file? (T)"), "refnum"=w157) -> ("error out"=w163:errorcluster)  [unwired: 8 out]
              n101 = call "_Remote Connect.vi"("error in (no error)"=w163, "IP Address"=w154) -> ("error out"=w210:errorcluster, "TCP"=w152:bool)  [unwired: 4 out]
              n102 = call "_Load Config File.vi"("error in (no error)"=w210) -> ("error out"=w211:errorcluster, "Instrument"=w148:string[])  [unwired: 1 in]
              n103 = Index Array(array=w148, index #1=1 ("index")) -> (element #1=w181:string, element #2=w180:string)  [unwired: 1 in]
              n104 = call "Get Oscillator Frequency.vi"("Array 3"=w148) -> ("Oscillator Freqs"=w147:dbl[])  [unwired: 9 in, 1 out]
              n105 = Number To Fractional String(number=w147, precision (6)=i16 4) -> (F-format string=w145:string[])  [unwired: 2 out]
              n106 = Match Pattern(string=w181, regular expression=w184) -> (offset past match=w186:i32)  [unwired: 4 out]
              n107 = Match Pattern(string=w180, regular expression=w184) -> (offset past match=w185:i32)  [unwired: 4 out]
              n108 = Greater Or Equal To 0?(x=w186) -> (x >= 0?=w183:bool)
              n109 = Greater Or Equal To 0?(x=w185) -> (x >= 0?=w182:bool)
              n110 = Or(x=w183, y=w182) -> (x .or. y?=w149:bool)
              n111 = Replace Array Subset(array=w173, new element=w145, index (col)=5 ("disabled index (col)")) -> (w168:string[][])  [unwired: 1 in]
              n112 = global write "_Global Configuration.vi" "UseLeybold"(w149) -> ()
              n113 = Replace Array Subset(array=w168, new element=w145, index (col)=7 ("disabled index (col)")) -> (w146:string[][])  [unwired: 1 in]
              n114 = property class="Tbl (strict)"(reference=w172, error in=w144, "Value"=w146) -> ()  [unwired: 2 out]
              n115 = Select(t="connected", s=w152, f="running in simulation") -> (s? t:f=w203:string)
              n116 = call "_Handle Error.vi"("error in (no error)"=w211) -> ()  [unwired: 2 in, 5 out]
              n117 = Not(x=w152) -> (.not. x?=w197:bool)
              n118 = call "_Remote Communicate.vi"("error in (no error)"=w211, "Command"=_RT_Command."Get Info") -> ("error out"=w153:errorcluster, "Info"=w209:string)  [unwired: 4 in, 2 out]
              n119 = global write "_Global Configuration.vi" "Sim"(w197) -> ()
              n120 = Format Into String(format string="Remote system, %s, is %s: %s", w154, w203, w209) -> (resulting string=w204:string)  [unwired: 2 in, 1 out]
              n121 = flat-sequence {
                tunnel: w153 -> [_]
                frame #0 {
                  n122 = call "_Launch Dynamic VI.vi"("VI Name"=path "Show Brief Status.vi" ("name or relative path")) -> ()  [unwired: 3 in, 1 out]
                }
              }
              n123 = case shown="False" w197 {
                frame False {
                  n124 = Wait (ms)(milliseconds to wait=u32 2800) -> ()  [unwired: 1 out]
                }
                frame True {
                }
              }
              n125 = call "_Log Events.vi"("error in (no error)"=w153, "Event"=w204, "Log Command"=_Log_Command."Write" ("File Command")) -> ("error out"=w151:errorcluster)  [unwired: 5 in, 1 out]
              n126 = property on="Tab Control" class="TabCtl (strict)"(error in=w151) -> ("Pages"=w178:refnum<vi>[])  [unwired: 1 in, 2 out]
              n127 = Index Array(array=w178, index #1=1 ("index"), index #2=2 ("index")) -> (element #1=w177:refnum<vi>, element #2=w176:refnum<vi>)
              n128 = Not(x=w149) -> (.not. x?=w150:bool)
              n129 = property class="Page"(reference=w177, "PageVis"=w149) -> ()  [unwired: 1 in, 2 out]
              n130 = property class="Page"(reference=w176, "PageVis"=w150) -> ()  [unwired: 1 in, 2 out]
            }
            frame #2 {
              w228 = TRUE ("UpdateInput (F)")
              w251 = T19[] []  # ADC Table
              w244 = u8 0 ("Disabled")
              w250 = FALSE ("Unit")
              n131 = local read "Pos/Neg"() -> (w238:enum32{"Positive", "Negative"})
              n132 = call "_Remote Communicate.vi"("Command"=_RT_Command."Get ADC Table") -> ("Info"=w252:string)  [unwired: 5 in, 3 out]
              n133 = Initialize Array("", 16 ("dimension size")) -> (w234:string[])
              n134 = Equal?(x=w238, y=enum32{"Positive", "Negative"}."Positive" ("Pos/Neg")) -> (x = y?=w230:bool)
              n135 = Unflatten From String(type=w251, binary string=w252) -> (value=w227:T19[])  [unwired: 1 in, 4 out]
              n136 = call "_Update Oscillators.vi"("UpdateInput (F)"=w228, "ADC Table"=w227, "Pole Swap (T)"=FALSE ("Update (T)"), "Update (T)"=w228, "Mode(pos)"=w230) -> ("Q1RF Frequency"=→"New Frequence" →"Old Frequency":dbl, "Instrument"=w231:string[], "Pole"=w225:bool[])  [unwired: 4 in]
              n137 = Replace Array Subset(array=w234, new element=w231, index=0) -> (w232:string[])
              n138 = call "Get Pole Orientations.vi"("Pole"=w225) -> ("Pole Swap Options Negative"=w239:T7, "Pole Swap Options Positive"=w240:T7)  [unwired: 9 in]
              n139 = local write "Pole Swap Options Positive"(w240) -> ()
              n140 = local write "Pole Swap Options Negative"(w239) -> ()
              n141 = property on="Detector" class="Tbl (strict)"("Disabled"=w244) -> ()  [unwired: 2 in, 2 out]
              n142 = property on="Gas Flows" class="Tbl (strict)"("Disabled"=w244) -> ()  [unwired: 2 in, 2 out]
              n143 = property on="Heaters" class="Tbl (strict)"("Disabled"=w244) -> ()  [unwired: 2 in, 2 out]
              n144 = property on="Source Probes" class="Tbl (strict)"("Disabled"=w244) -> ()  [unwired: 2 in, 2 out]
              n145 = property on="Corona/Curtain High Voltage" class="Tbl (strict)"("Disabled"=w244) -> ()  [unwired: 2 in, 2 out]
              n146 = property on="Lens 1" class="Tbl (strict)"("Disabled"=w244) -> ()  [unwired: 2 in, 2 out]
              n147 = property on="Lens 2" class="Tbl (strict)"("Disabled"=w244) -> ()  [unwired: 2 in, 2 out]
              n148 = property on="Run" class="Bool"("Visible"=TRUE) -> ()  [unwired: 2 in, 2 out]
              n149 = property on="Cancel" class="Bool (strict)"("Visible"=w250) -> ()  [unwired: 2 in, 2 out]
              n150 = property on="Turbo OK" class="Bool (strict)"("Visible"=w250) -> ()  [unwired: 2 in, 2 out]
              n151 = property on="SVG OK" class="Bool (strict)"("Visible"=w250) -> ()  [unwired: 2 in, 2 out]
              n152 = property on="Quad/Tune OK" class="Bool (strict)"("Visible"=w250) -> ()  [unwired: 2 in, 2 out]
              n153 = property on="Intlk/Per OK" class="Bool (strict)"("Visible"=w250) -> ()  [unwired: 2 in, 2 out]
              n154 = property on="Firmware OK" class="Bool (strict)"("Visible"=w250) -> ()  [unwired: 2 in, 2 out]
              n155 = property on="Progress Bar" class="Slide (strict)"("Visible"=w250) -> ()  [unwired: 2 in, 2 out]
              n156 = property on="Voltage OK" class="Bool (strict)"("Visible"=w250) -> ()  [unwired: 2 in, 2 out]
              n157 = call <vilib>:"Application Directory.vi"() -> ("Application Directory"=w241:path)
              n158 = Build Path(base path=w241, name or relative path="DEFAULT_SETTINGS.d2m") -> (appended path=w248:path)
              n159 = property on="Load Tune File" class="Bool (strict)"("Val(Sgnl)"=FALSE ("Value (Signaling)")) -> ()  [unwired: 2 in, 2 out]
              n160 = property on="Refresh" class="Bool (strict)"("Val(Sgnl)"=TRUE ("Use temporary file (F)")) -> ()  [unwired: 2 in, 2 out]
              n161 = call "_Save All Tables.vi"("SaveOption (Temporary File)"=T16."Temporary File" ("Use temporary file (F)")) -> ()  [unwired: 2 in, 5 out]
              n162 = property on="Tab Control" class="TabCtl (strict)"("Val(Sgnl)"=T2."System Config" ("Value (Signaling)")) -> ()  [unwired: 2 in, 2 out]
              n163 = local write "Tune File"(w248) -> ()
              n164 = local write "Running"(w250) -> ()
              n165 = local write "Quit"(w250) -> ()
              n166 = local write "LBFreqTemp"(FALSE ("LBFreqTemp")) -> ()
              n167 = local write "Cancel"(w250) -> ()
              "ADC List" <- 130 ("ADC List")
            }
            frame #3 {
              w262 = cluster{u32, u32}[] [{16711680, 16711680}, {10421504, 10421504}, {8323072, 8323072}, {5177856, 5177856}]  # RedColor
              w263 = cluster{u32, u32}[] [{12369084, 12369084}, {9868950, 9868950}, {12369084, 12369084}, {9868950, 9868950}]  # GrayColor
              w272 = T31 {"Door"=TRUE, "Curtain"=TRUE, "Pressure"=TRUE, "Turbo"=TRUE, "SysPoll"=TRUE, "GasFlag"=TRUE, "SourceExhaust"=TRUE}  # StartupOptions
              # "Initialize the options based on current settings"
              n168 = call "_Remote Communicate.vi"("Command"=_RT_Command."Get Startup") -> ("error out"=w259:errorcluster, "Info"=w275:string)  [unwired: 5 in, 2 out]
              n169 = call "_Remote Get Brief Status.vi"("error in (no error)"=w259) -> ("error out"=w258:errorcluster)  [unwired: 1 in, 2 out]
              n170 = call <vilib>:"Trim Whitespace.vi"("string"=w275) -> ("trimmed string"=w274:string)  [unwired: 1 in]
              n171 = Empty String/Path?(string/path=w274) -> (empty?=w273:bool)
              n172 = Unflatten From String(type=w272, binary string=w275, error in (no error)=w258) -> (value=w271:T31, error out=w257:errorcluster)  [unwired: 3 out]
              n173 = Select(t=w272, s=w273, f=w271) -> (s? t:f=w270:T31)
              n174 = Unbundle By Name(w270) -> ("Door"=w269:bool, "Curtain"=w268:bool, "Pressure"=w267:bool, "Turbo"=w266:bool, "SysPoll"=w265:bool, "GasFlag"=w264:bool)
              n175 = Compound Arithmetic op=AND(w269, w268, w267, w266, w265, w264) -> (w260:bool)
              n176 = Select(t=w263, s=w260, f=w262) -> (s? t:f=w261:cluster{u32, u32}[])
              n177 = property on="Options" class="Bool"(error in=w257, "Colors [4]"=w261) -> (error out=w256:errorcluster)  [unwired: 1 in, 1 out]
              n178 = call "_Remote Set PIC.vi"("error in (no error)"=w256, "PIC Channel"=_PIC_Channel."Corona +HV") -> ("error out"=w282:errorcluster, "Received Header"=→"Corona":u16)  [unwired: 1 in, 3 out]
              n179 = call "_Remote Set PIC.vi"("error in (no error)"=w282, "PIC Channel"=_PIC_Channel."Source 1 Temp") -> ("error out"=w281:errorcluster, "Received Header"=→"Source 1":u16)  [unwired: 1 in, 3 out]
              n180 = call "_Remote Set PIC.vi"("error in (no error)"=w281, "PIC Channel"=_PIC_Channel."Source 2 Temp") -> ("error out"=w280:errorcluster, "Received Header"=→"Source 2":u16)  [unwired: 1 in, 3 out]
              n181 = call "_Remote Set PIC.vi"("error in (no error)"=w280, "PIC Channel"=_PIC_Channel."HSID Temp") -> ("Received Header"=→"HSID":u16)  [unwired: 1 in, 4 out]
            }
            frame #4 {
              w296 = FALSE  # FrequencyTune
              w298 = FALSE  # CalAjusted
              w288 = _RT_Instrument_State."Ready" ("y")
              w305 = FALSE  # Running
              w306 = TRUE  # Update
              n182 = call <vilib>:"Unset Busy.vi"("error in (no error)"=w290) -> ("error out"=w289:errorcluster)  [unwired: 1 in, 9 out]
              n183 = Bundle("Configuration 2"=T18 {"Table"=[{"Name"="Q1 RF", "Ch#"=1, "Min"=0.0, "Max"=1500.0, "Def+"=400.0, "Def-"=400.0, "Offset"=0.0, "Slope"=218.45, "Type"=64, "Description"="Quadrupole 1 RF", "SettleT"=5.0}, {"Name"="Q1 DC", "Ch#"=4, "Min"=0.0, "Max"=1500.0, "Def+"=600.0, "Def-"=600.0, "Offset"=0.0, "Slope"=218.45, "Type"=64, "Description"="Quadrupole 1 DC", "SettleT"=5.0}, {"Name"="Q1 RR", "Ch#"=7, "Min"=0.0, "Max"=64000.0, "Def+"=32000.0, "Def-"=32000.0, "Offset"=32768.0, "Slope"=-1.0, "Type"=64, "Description"="Quadrupole 1 PW", "SettleT"=5.0}, {"Name"="Q2 RF", "Ch#"=2, "Min"=0.0, "Max"=1500.0, "Def+"=400.0, "Def-"=400.0, "Offset"=0.0, "Slope"=218.45, "Type"=64, "Description"="Quadrupole 2 RF", "SettleT"=5.0}, {"Name"="Q2 DC", "Ch#"=5, "Min"=0.0, "Max"=1500.0, "Def+"=600.0, "Def-"=600.0, "Offset"=0.0, "Slope"=218.45, "Type"=64, "Description"="Quadrupole 2 DC", "SettleT"=5.0}, {"Name"="Q2 RR", "Ch#"=9, "Min"=0.0, "Max"=64000.0, "Def+"=32000.0, "Def-"=32000.0, "Offset"=32768.0, "Slope"=-1.0, "Type"=64, "Description"="Quadrupole 2 PW", "SettleT"=5.0}, {"Name"="M1 RF", "Ch#"=3, "Min"=0.0, "Max"=500.0, "Def+"=400.0, "Def-"=400.0, "Offset"=0.0, "Slope"=14.7, "Type"=6, "Description"="Multipole 1 RF", "SettleT"=5.0}, {"Name"="EV", "Ch#"=20, "Min"=-400.0, "Max"=400.0, "Def+"=0.0, "Def-"=0.0, "Offset"=32768.0, "Slope"=-65.7, "Type"=7, "Description"="Entrance voltage", "SettleT"=5.0}, {"Name"="ED", "Ch#"=21, "Min"=-400.0, "Max"=400.0, "Def+"=0.0, "Def-"=0.0, "Offset"=32768.0, "Slope"=-131.0, "Type"=7, "Description"="Not Used 1", "SettleT"=5.0}, {"Name"="M1", "Ch#"=19, "Min"=-400.0, "Max"=400.0, "Def+"=0.0, "Def-"=0.0, "Offset"=32768.0, "Slope"=-65.6, "Type"=7, "Description"="Multipole 1", "SettleT"=5.0}, {"Name"="L1", "Ch#"=18, "Min"=-400.0, "Max"=400.0, "Def+"=0.0, "Def-"=0.0, "Offset"=32760.0, "Slope"=-65.9, "Type"=7, "Description"="Multipole Len 1", "SettleT"=5.0}, {"Name"="M2", "Ch#"=22, "Min"=-400.0, "Max"=400.0, "Def+"=0.0, "Def-"=0.0, "Offset"=32768.0, "Slope"=-66.0, "Type"=7, "Description"="Multipole 2", "SettleT"=5.0}, {"Name"="L2", "Ch#"=11, "Min"=-400.0, "Max"=400.0, "Def+"=0.0, "Def-"=0.0, "Offset"=32768.0, "Slope"=-65.9, "Type"=7, "Description"="Multipole Len 2", "SettleT"=5.0}, {"Name"="PF", "Ch#"=12, "Min"=-400.0, "Max"=400.0, "Def+"=-16.0, "Def-"=16.0, "Offset"=32768.0, "Slope"=-65.8, "Type"=7, "Description"="Prefilter 1", "SettleT"=5.0}, {"Name"="Q1", "Ch#"=6, "Min"=-150.0, "Max"=150.0, "Def+"=-1.0, "Def-"=1.0, "Offset"=32755.0, "Slope"=-131.3, "Type"=11, "Description"="Quadrupole 1", "SettleT"=5.0}, {"Name"="CC L1", "Ch#"=13, "Min"=-400.0, "Max"=400.0, "Def+"=0.0, "Def-"=0.0, "Offset"=32768.0, "Slope"=-65.8, "Type"=7, "Description"="Collision Cell Lens 1", "SettleT"=5.0}, {"Name"="CC L2", "Ch#"=14, "Min"=-400.0, "Max"=400.0, "Def+"=-100.0, "Def-"=100.0, "Offset"=32768.0, "Slope"=-65.8, "Type"=7, "Description"="Collision Cell Lens 2", "SettleT"=5.0}, {"Name"="CC", "Ch#"=23, "Min"=-400.0, "Max"=400.0, "Def+"=-50.0, "Def-"=50.0, "Offset"=32768.0, "Slope"=-65.8, "Type"=7, "Description"="Collision Energy", "SettleT"=5.0}, {"Name"="CC AF", "Ch#"=10, "Min"=-400.0, "Max"=400.0, "Def+"=50.0, "Def-"=-50.0, "Offset"=32768.0, "Slope"=-65.8, "Type"=7, "Description"="Axial Field", "SettleT"=5.0}, {"Name"="CC L3", "Ch#"=15, "Min"=-400.0, "Max"=400.0, "Def+"=-52.5, "Def-"=52.5, "Offset"=32768.0, "Slope"=-65.7, "Type"=7, "Description"="Collision Cell Lens 3", "SettleT"=5.0}, {"Name"="CC L4", "Ch#"=16, "Min"=-400.0, "Max"=400.0, "Def+"=-72.5, "Def-"=72.5, "Offset"=32768.0, "Slope"=-65.7, "Type"=7, "Description"="Collision Cell Lens 4", "SettleT"=5.0}, {"Name"="Q2", "Ch#"=8, "Min"=-150.0, "Max"=150.0, "Def+"=-54.0, "Def-"=54.0, "Offset"=32756.0, "Slope"=-131.3, "Type"=11, "Description"="Quadrupole 2", "SettleT"=5.0}, {"Name"="ID", "Ch#"=17, "Min"=-400.0, "Max"=400.0, "Def+"=-100.0, "Def-"=100.0, "Offset"=32768.0, "Slope"=-65.8, "Type"=18, "Description"="Detector Deflector", "SettleT"=5.0}, {"Name"="DISC", "Ch#"=32, "Min"=10.0, "Max"=2000.0, "Def+"=20.0, "Def-"=20.0, "Offset"=-10.0, "Slope"=1.23, "Type"=18, "Description"="Discriminator", "SettleT"=5.0}, {"Name"="DV", "Ch#"=34, "Min"=0.0, "Max"=3500.0, "Def+"=1000.0, "Def-"=1000.0, "Offset"=0.0, "Slope"=0.615, "Type"=18, "Description"="Detector Voltage", "SettleT"=5.0}, {"Name"="DET horn", "Ch#"=200, "Min"=0.0, "Max"=5500.0, "Def+"=5500.0, "Def-"=5500.0, "Offset"=0.0, "Slope"=0.615, "Type"=16, "Description"="Detector Horn", "SettleT"=200.0}, {"Name"="LS400A", "Ch#"=36, "Min"=0.0, "Max"=420.0, "Def+"=420.0, "Def-"=420.0, "Offset"=0.0, "Slope"=8.4, "Type"=64, "Description"="Len Power Supply A +400", "SettleT"=5.0}, {"Name"="LS-400A", "Ch#"=37, "Min"=-420.0, "Max"=-55.0, "Def+"=-420.0, "Def-"=-420.0, "Offset"=-433.0, "Slope"=-8.4, "Type"=64, "Description"="Len Power Supply A -400", "SettleT"=5.0}, {"Name"="LS400B", "Ch#"=38, "Min"=0.0, "Max"=420.0, "Def+"=420.0, "Def-"=420.0, "Offset"=0.0, "Slope"=8.4, "Type"=64, "Description"="Len Power Supply B +400", "SettleT"=5.0}, {"Name"="LS-400B", "Ch#"=39, "Min"=-420.0, "Max"=-55.0, "Def+"=-420.0, "Def-"=-420.0, "Offset"=-433.0, "Slope"=-8.4, "Type"=64, "Description"="Len Power Supply B  -400", "SettleT"=5.0}, {"Name"="QPS800", "Ch#"=40, "Min"=0.0, "Max"=600.0, "Def+"=600.0, "Def-"=600.0, "Offset"=0.0, "Slope"=4.25, "Type"=64, "Description"="Quad Power Supply +800", "SettleT"=5.0}, {"Name"="QPS-800", "Ch#"=41, "Min"=-600.0, "Max"=-110.0, "Def+"=-600.0, "Def-"=-600.0, "Offset"=-433.0, "Slope"=-4.2, "Type"=64, "Description"="Quad Power Supply -800", "SettleT"=5.0}, {"Name"="DG", "Ch#"=26, "Min"=30.0, "Max"=300.0, "Def+"=40.0, "Def-"=40.0, "Offset"=0.0, "Slope"=32.765, "Type"=32, "Description"="Drying Gas", "SettleT"=1000.0}, {"Name"="NG1", "Ch#"=27, "Min"=0.0, "Max"=500.0, "Def+"=0.0, "Def-"=0.0, "Offset"=0.0, "Slope"=32.765, "Type"=32, "Description"="Nebulizer Gas 1", "SettleT"=1000.0}, {"Name"="HG1", "Ch#"=29, "Min"=0.0, "Max"=350.0, "Def+"=0.0, "Def-"=0.0, "Offset"=0.0, "Slope"=32.765, "Type"=32, "Description"="Heating Gas 1", "SettleT"=1000.0}, {"Name"="NG2", "Ch#"=28, "Min"=0.0, "Max"=500.0, "Def+"=0.0, "Def-"=0.0, "Offset"=0.0, "Slope"=32.765, "Type"=32, "Description"="Nebulizer Gas 2", "SettleT"=1000.0}, {"Name"="HG2", "Ch#"=30, "Min"=0.0, "Max"=350.0, "Def+"=0.0, "Def-"=0.0, "Offset"=0.0, "Slope"=32.765, "Type"=32, "Description"="Heating Gas 2", "SettleT"=1000.0}, {"Name"="CC P", "Ch#"=43, "Min"=0.0, "Max"=500.0, "Def+"=0.0, "Def-"=0.0, "Offset"=0.0, "Slope"=32.765, "Type"=6, "Description"="Collision Pressure", "SettleT"=3000.0}, {"Name"="SX", "Ch#"=42, "Min"=0.0, "Max"=500.0, "Def+"=0.0, "Def-"=0.0, "Offset"=0.0, "Slope"=32.765, "Type"=32, "Description"="Source Exhaust", "SettleT"=1000.0}, {"Name"="ISV2", "Ch#"=204, "Min"=-6000.0, "Max"=6000.0, "Def+"=0.0, "Def-"=0.0, "Offset"=0.0, "Slope"=0.04, "Type"=34, "Description"="Ion Spray HV2", "SettleT"=200.0}, {"Name"="ISV1", "Ch#"=203, "Min"=-6000.0, "Max"=6000.0, "Def+"=0.0, "Def-"=0.0, "Offset"=0.0, "Slope"=0.04, "Type"=34, "Description"="Ion Spray HV1", "SettleT"=200.0}, {"Name"="CD", "Ch#"=202, "Min"=-255.0, "Max"=255.0, "Def+"=0.0, "Def-"=0.0, "Offset"=0.0, "Slope"=1.0, "Type"=34, "Description"="Corona Discharge", "SettleT"=2000.0}, {"Name"="CAP", "Ch#"=201, "Min"=-1100.0, "Max"=1100.0, "Def+"=0.0, "Def-"=0.0, "Offset"=0.0, "Slope"=0.22, "Type"=32, "Description"="Curtain Cap", "SettleT"=200.0}, {"Name"="HSID T", "Ch#"=81, "Min"=0.0, "Max"=300.0, "Def+"=200.0, "Def-"=200.0, "Offset"=0.0, "Slope"=1.0, "Type"=32, "Description"="HSID Temperature", "SettleT"=3000.0}, {"Name"="P1 T", "Ch#"=86, "Min"=0.0, "Max"=500.0, "Def+"=0.0, "Def-"=0.0, "Offset"=0.0, "Slope"=0.7, "Type"=32, "Description"="Probe 1 Temp", "SettleT"=3000.0}, {"Name"="P2 T", "Ch#"=84, "Min"=0.0, "Max"=500.0, "Def+"=0.0, "Def-"=0.0, "Offset"=0.0, "Slope"=0.7, "Type"=32, "Description"="Probe 2 Temp", "SettleT"=3000.0}], "Instrument"=["C:\\USERS\\PUBLIC\\Ion Sniffer\\GOLD\\Config\\Config-Default-Molana-110209.c3n", "Ion Sniffer 03", "Ionics 3Q Simulation", "0", "0", "0", "0", "172.16.0.2", "T", "0", "2864776525 47523813", "2864776525 47523813", "2864776499 66529043", "0", "0"]}, "FrequencyTune"=w296, "CalAjusted"=w298, "Update"=w306, "Running"=w305, "ADC Table"=w299) -> (w304:T32)  [unwired: 1 out]
              n184 = while {
                shift-right: [w499] -> w297
                shift-left: w304 -> [w501]
                tunnel: w307 -> [w498]
                tunnel: w303 -> [w497]
                tunnel: w302 -> [w496]
                tunnel: w301 -> [w495]
                tunnel: w293 -> [w494]
                tunnel: w289 -> [w493]
                stop <- w502 stop-if-true
                n185 = event shown="[5] \"Load Firmware\": Value Change" {
                  selector: _ -> [_ _ _ _ _ _ _ _ _ _ _ _ _ _ _ _ _ _ _ _ _ _ _ _ _ _ _ _ _ _ _ _ _ _ _ _ _ _ _ _ _ _ _ _ _ _ _ _ _ _ _ _ _ _ _ _ _ _ _ _ _ _ _ _ _ _]
                  dyn-events: _ -> [_ _ _ _ _ _ _ _ _ _ _ _ _ _ _ _ _ _ _ _ _ _ _ _ _ _ _ _ _ _ _ _ _ _ _ _ _ _ _ _ _ _ _ _ _ _ _ _ _ _ _ _ _ _ _ _ _ _ _ _ _ _ _ _ _ _]
                  timeout: 1800 -> [_ _ _ _ _ _ _ _ _ _ _ _ _ _ _ _ _ _ _ _ _ _ _ _ _ _ _ _ _ _ _ _ _ _ _ _ _ _ _ _ _ _ _ _ _ _ _ _ _ _ _ _ _ _ _ _ _ _ _ _ _ _ _ _ _ _]
                  tunnel: [w506 _ w599 _ _ _ _ _ _ _ _ _ _ _ _ _ _ _ _ _ _ _ _ _ _ _ _ _ _ _ _ _ _ _ _ _ _ _ _ _ _ _ _ _ _ _ _ _ _ _ _ _ _ _ _ _ _ _ _ _ _ _ _ _ _ _] -> w502
                  tunnel: w501 -> [w507 w524 w596 w747 w758 w768 w842 w896 w906 w909 w956 w984 w988 w1005 w1022 w1039 w1057 w1069 w1081 w1092 w1110 w1139 w1155 w1162 w1169 w1176 w1188 w1195 w1197 w1222 w1227 w1233 w1239 w1245 w1253 w1259 w1265 w1271 w1284 w1286 w1327 w1336 w1343 w1345 w1356 w1373 w1378 w1383 w1388 w1393 w1398 w1420 w1433 w1439 w1444 w1449 w1461 w1465 w1466 w1468 w1470 w1480 w1546 w1596 w1598 w1624]
                  tunnel: [w507 w526 w595 w751 w755 w767 w845 w895 w906 w909 w956 w984 w988 w1005 w1022 w1039 w1057 w1069 w1081 w1092 w1110 w1139 w1155 w1162 w1169 w1176 w1188 w1195 w1197 w1222 w1227 w1233 w1239 w1245 w1253 w1259 w1265 w1271 w1284 w1285 w1326 w1336 w1343 w1345 w1356 w1373 w1378 w1383 w1388 w1393 w1398 w1420 w1433 w1439 w1444 w1449 w1461 w1465 w1466 w1468 w1470 w1479 w1545 w1596 w1597 w1624] -> w499
                  tunnel: w498 -> [_ w525 _ w753 _ _ _ _ _ _ _ _ _ _ _ _ _ _ _ _ _ _ _ _ _ _ _ _ _ _ _ _ _ _ _ _ _ _ _ _ _ _ _ _ _ _ _ _ _ _ _ _ _ _ _ _ _ _ _ _ _ _ _ _ _ _]
                  tunnel: w497 -> [_ w521 _ _ _ _ _ _ _ _ _ _ _ _ _ _ _ _ _ _ _ _ _ _ _ _ _ _ _ _ _ _ _ _ _ _ _ _ _ _ _ _ _ _ _ _ _ _ _ _ _ _ _ _ _ _ _ _ _ _ _ _ _ _ _ _]
                  tunnel: w496 -> [_ w520 _ _ _ _ _ _ _ _ _ _ _ _ _ _ _ _ _ _ _ _ _ _ _ _ _ _ _ _ _ _ _ _ _ _ _ _ _ _ _ _ _ _ _ _ _ _ _ _ _ _ _ _ _ _ _ _ _ _ _ _ _ _ _ _]
                  tunnel: w495 -> [_ w519 w594 _ _ _ _ _ _ _ _ _ _ _ _ _ _ _ _ _ _ _ _ _ _ _ _ _ _ w1226 _ _ _ _ _ _ _ _ _ w1288 _ w1332 w1339 _ _ _ _ _ _ _ _ _ _ _ _ _ _ _ _ _ _ _ _ _ _ _]
                  tunnel: w494 -> [_ _ w593 _ _ _ _ _ _ _ _ _ _ _ _ _ _ _ _ _ _ _ _ _ _ _ _ _ _ _ _ _ _ _ _ _ _ _ w1282 _ _ _ _ _ _ _ _ _ _ _ _ _ _ _ _ _ _ _ _ _ _ _ _ _ _ _]
                  tunnel: w493 -> [_ _ _ _ _ _ _ _ _ _ _ _ _ _ _ _ _ _ _ _ _ _ _ _ _ _ _ _ _ _ _ _ _ _ _ _ _ _ w1283 _ _ _ _ _ _ _ _ _ _ _ _ _ _ _ _ _ _ _ _ _ _ _ _ _ _ _]
                  event Panel Close? {
                    w503 = FALSE ("Update")
                    w506 = TRUE ("Discard?")
                    n186 = event-data() -> ()  [unwired: 2 out]
                    n187 = call "_Remote Communicate.vi"("Command"=_RT_Command."Stop") -> ("error out"=w504:errorcluster)  [unwired: 5 in, 3 out]
                    n188 = call "_Remote Park Lens.vi"("error in"=w504, "All Ch (F)"=TRUE) -> ()  [unwired: 6 out]
                    n189 = global write "_Global Configuration.vi" "Quit"(w506) -> ()
                    n190 = global write "_Global Configuration.vi" "Run"(w503) -> ()
                    n191 = local write "Running"(w503) -> ()
                    n192 = event-data("Discard?"=w506) -> ()  [unwired: 1 in, 1 out]
                    "Quit" <- w506
                  }
                  event Timeout {
                    n193 = event-data() -> ()  [unwired: 2 out]
                    n194 = Unbundle By Name(w524) -> ("Update"=w523:bool, "Running"=w522:bool, "ADC Table"=w518:T19[])
                    n195 = case shown="False" w523 {
                      tunnel: w524 -> [w532 w590]
                      tunnel: [w531 w588] -> w526
                      tunnel: w522 -> [w534 _]
                      tunnel: w525 -> [w533 _]
                      tunnel: w518 -> [w530 _]
                      tunnel: w521 -> [w529 _]
                      tunnel: w520 -> [w528 _]
                      tunnel: w519 -> [w527 _]
                      frame False {
                        n196 = case shown="False" w534 {
                          tunnel: w533 -> [_ w576]
                          tunnel: w532 -> [w570 w571]
                          tunnel: [w570 w571] -> w531
                          tunnel: w530 -> [w537 _]
                          tunnel: w529 -> [w568 _]
                          tunnel: w528 -> [w565 _]
                          tunnel: w527 -> [w561 _]
                          frame False {
                            w543 = T6 4 items=["None", "ESI", "APCI", "APPI", "MicroSpray"] ("y")
                            w550 = FALSE ("Pole Swap (T)")
                            n197 = call "_Remote Communicate.vi"("Command"=_RT_Command."Read ADC") -> ("Data Array"=w538:i32[])  [unwired: 5 in, 3 out]
                            n198 = call "_Update Oscillators.vi"("UpdateInput (F)"=w550, "ADC Array"=w538, "ADC Table"=w537, "Pole Swap (T)"=w550, "Update (T)"=w550, "Oscillator Settings"=w561) -> ()  [unwired: 2 in, 4 out]
                            n199 = call "_Check ADCs.vi"("ADC Table"=w537, "ADC Values"=w538, "ADC List Ref"=w565) -> ("Interlocks"=w560:bool[])  [unwired: 4 out]
                            n200 = call "_Remote Calculate ADC.vi"("ADC Table"=w537, "ADC Channel (64)"=u8 56, "ADC Values"=w538) -> ("User Value"=→"M1RF Readback":dbl)  [unwired: 1 in, 3 out]
                            n201 = local read "VoltageInput"() -> (w566:dbl[])
                            n202 = call "_Remote Calculate ADC.vi"("ADC Table"=w537, "ADC Channel (64)"=u8 8, "ADC Values"=w538) -> ("User Value"=→"Main System Current (A)":dbl)  [unwired: 1 in, 3 out]
                            n203 = local read "SG Input"() -> (w559:dbl[])
                            n204 = call "_Check Voltages.vi"("Unit"="Unit", "SGInput"=w559, "ADC Table"=w537, "ADC Values"=w538, "VoltageInput"=w566, "Reference"=w568) -> ("Source 2 Type:"=w545:T6, "Source 1 Type:"=w544:T6, "SVG OK"=→"SVG OK":bool, "Voltage OK"=→"Voltage OK":bool, "Pressure"=→"Vacuum Readings by Region" →"Pressures:":string[][], "DC OK"=→"Quad/Tune OK":bool)
                            "Source 1 Type:" <- w544
                            "Source 2 Type:" <- w545
                            n205 = global read "_Global Configuration.vi" "Single Source"() -> (w558:bool)
                            n206 = Equal?(x=w545, y=w543) -> (x = y?=w546:bool)
                            n207 = Equal?(x=w544, y=w543) -> (x = y?=w542:bool)
                            n208 = Index Array(array=w560) -> (element #1=w552:bool, element #2=w553:bool, element #3=w541:bool, element #4=w547:bool, element #5=w555:bool, element #6=w556:bool, element #7=w557:bool)  [unwired: 7 in]
                            "DoorOK" <- w552
                            "VacRdy" <- w553
                            "DryingGasOK" <- w555
                            "ExhaustOK" <- w556
                            "SourceOK" <- w557
                            n209 = Compound Arithmetic op=OR(w547, w546, w558) -> (w554:bool)
                            "HG2OK" <- w554
                            n210 = Or(x=w542, y=w541) -> (x .or. y?=→"HG1OK":bool)
                            n211 = Compound Arithmetic op=AND(w552, w553, w541, w554, w555, w556, w557) -> (→"Intlk/Per OK":bool)
                          }
                          frame True {
                            n212 = Dequeue Element(queue=w576, timeout in ms (-1)=1) -> (element=w574:cluster{T13, dbl, "error out":errorcluster}, timed out?=w573:bool)  [unwired: 1 in, 2 out]
                            n213 = call "_Current Data Global.vi"("Operation"=_Data_Operation."Get Data") -> ()  [unwired: 3 in, 4 out]
                            n214 = case shown="False" w573 {
                              tunnel: w574 -> [w580 _]
                              frame False {
                                n215 = Unbundle(w580) -> (w579:T13, w577:dbl, "error out"=w578:errorcluster)
                                n216 = case shown="\"End\"" w579 {
                                tunnel: w578 -> [_ w581 w582]
                                tunnel: w577 -> [_ _ _]
                                frame "Init", Default {
                                }
                                frame "End" {
                                n217 = call "_Handle Error.vi"("error in (no error)"=w581) -> ()  [unwired: 2 in, 5 out]
                                }
                                frame "Error" {
                                n218 = call "_Handle Error.vi"("error in (no error)"=w582) -> ()  [unwired: 2 in, 5 out]
                                }
                                }
                              }
                              frame True {
                              }
                            }
                          }
                        }
                      }
                      frame True {
                        w587 = T33 1 items=["8080 Series", "100 Series", "200 Series", "300 Series", "Other Series"] ("Model Family (100)")
                        n219 = call "_Check Model Family.vi"("Model Family (100)"=w587) -> ("Yes"=w586:bool)
                        n220 = Select(t=enum32{"0", "200", "100"}."100" ("IonPathMap"), s=w586, f=enum32{"0", "200", "100"}."200" ("IonPathMap")) -> (s? t:f=w585:enum32{"0", "200", "100"})
                        n221 = stacked-sequence {
                          tunnel: w585 -> [w591 _]
                          frame #0 {
                            "IonPathMap" <- w591
                          }
                          frame #1 {
                            n222 = property on="Ion Path" class="Clust (strict)"("Visible"=TRUE) -> ()  [unwired: 2 in, 2 out]
                          }
                        }
                        n223 = Bundle By Name(cluster=w590, "Update"=FALSE) -> (w588:T32)
                      }
                    }
                    n224 = local read "Serial Number"() -> (w509:string)
                    n225 = Format Into String(format string="Serial Number: %s", w509) -> (resulting string=→"SN":string)  [unwired: 2 in, 1 out]
                    n226 = Get Date/Time In Seconds() -> (seconds since 1Jan1904=w517:timestamp)
                    n227 = Get Date/Time String(seconds (now)=w517, want seconds? (F)=TRUE) -> (date string=w514:string, time string=w513:string)  [unwired: 1 in]
                    n228 = Format Into String(format string="%s %s", w514, w513) -> (resulting string=→"Date/Time":string)  [unwired: 2 in, 1 out]
                  }
                  event Menu Selection (User) {
                    n229 = event-data() -> ("ItemTag"=w600:string)  [unwired: 1 out]
                    n230 = Unbundle By Name(w596) -> ("Running"=w601:bool, "ADC Table"=w598:T19[])
                    n231 = case shown="False" w601 {
                      tunnel: w600 -> [w607 _]
                      tunnel: [w606 _] -> w599
                      tunnel: w598 -> [w605 w741]
                      tunnel: [w604 w741] -> w597
                      tunnel: w594 -> [w603 _]
                      tunnel: w593 -> [w602 _]
                      frame False {
                        n232 = case shown="\"Load All Tables\"" w607 {
                          tunnel: [_ _ _ w631 _ _ _ _ _ _ _ _ _ _ _ _ _ _ _ _ w725 _] -> w606
                          tunnel: w605 -> [w609 w610 w623 w629 w633 w637 w642 w647 w652 w657 w662 w667 w671 w692 w694 w698 w702 w706 w707 w710 w727 w740]
                          tunnel: [w609 w610 w624 w629 w633 w636 w641 w646 w651 w656 w661 w666 w675 w692 w694 w698 w702 w706 w707 w710 w727 w740] -> w604
                          tunnel: w603 -> [_ _ w618 _ _ _ _ _ _ _ _ _ _ _ _ _ _ _ _ _ _ _]
                          tunnel: w602 -> [_ _ _ _ _ _ _ _ _ _ _ _ w670 _ _ _ _ _ _ _ _ _]
                          frame "Save All Tables" {
                            n233 = call "_Save All Tables.vi"("SaveOption (Temporary File)"=_SaveOption."Use Dialog") -> ()  [unwired: 2 in, 5 out]
                          }
                          frame Default {
                          }
                          frame "Load All Tables" {
                            w622 = FALSE ("Update (T)")
                            n234 = local read "Pos/Neg"() -> (w613:enum32{"Positive", "Negative"})
                            n235 = Equal?(x=w613, y=enum32{"Positive", "Negative"}."Positive" ("Pos/Neg")) -> (x = y?=w611:bool)
                            n236 = local write "LoadedTable"(TRUE ("LoadedTable")) -> ()
                            n237 = call "_Load All Tables.vi"() -> ("ADC Table"=w620:T19[], "Loaded ADC"=w625:bool)  [unwired: 1 in, 5 out]
                            n238 = call "_Update Oscillators.vi"("UpdateInput (F)"=TRUE, "ADC Table"=w620, "Pole Swap (T)"=w622, "Update (T)"=w622, "Mode(pos)"=w611, "Oscillator Settings"=w618) -> ("Q1RF Frequency"=w617:dbl, "Pole"=w614:bool[])  [unwired: 2 in, 2 out]
                            n239 = local write "New Frequence"(w617) -> ()
                            n240 = local write "Old Frequency"(w617) -> ()
                            n241 = call "Get Pole Orientations.vi"("Pole"=w614) -> ("Pole Swap Options Negative"=w615:T7, "Pole Swap Options Positive"=w616:T7)  [unwired: 9 in]
                            n242 = local write "Pole Swap Options Positive"(w616) -> ()
                            n243 = local write "Pole Swap Options Negative"(w615) -> ()
                            n244 = property on="Refresh" class="Bool (strict)"("Val(Sgnl)"=TRUE ("Use temporary file (F)")) -> ()  [unwired: 2 in, 2 out]
                            n245 = Select(t=w620, s=w625, f=w623) -> (s? t:f=w624:T19[])
                          }
                          frame "Quit" {
                            w631 = TRUE
                            n246 = call "_Remote Communicate.vi"("Command"=_RT_Command."Stop") -> ("error out"=w627:errorcluster)  [unwired: 5 in, 3 out]
                            n247 = call "_Remote Park Lens.vi"("error in"=w627, "All Ch (F)"=TRUE) -> ()  [unwired: 6 out]
                            n248 = global write "_Global Configuration.vi" "Run"(FALSE ("Run")) -> ()
                            n249 = global write "_Global Configuration.vi" "Quit"(w631) -> ()
                            n250 = local write "Quit"(w631) -> ()
                          }
                          frame "ADC Plot" {
                            n251 = call "_Launch Dynamic VI.vi"("VI Name"=path "ADC Plot.vi" ("name or relative path")) -> ()  [unwired: 3 in, 1 out]
                          }
                          frame "Quad DC without PS Test Points" {
                            w635 = T34 0 items=["Quad DC Board", "Lens 1 (Slot 8) Module", "Lens 2 (Slot 6) Module", "Detector Board", "Quad DC Board with Test Points", "Lens 1 Module with Test Points", "Len 2 Module with Test Points", "", "", "", "", ""] ("Board")
                            n252 = call "Board Calibrator.vi"("Board"=w635) -> ("ADC Table"=w638:T19[], "Suceeded"=w639:bool)  [unwired: 5 out]
                            n253 = Select(t=w638, s=w639, f=w637) -> (s? t:f=w636:T19[])
                          }
                          frame "Quad DC with PS Test Points" {
                            w640 = T34 4 items=["Quad DC Board", "Lens 1 (Slot 8) Module", "Lens 2 (Slot 6) Module", "Detector Board", "Quad DC Board with Test Points", "Lens 1 Module with Test Points", "Len 2 Module with Test Points", "", "", "", "", ""] ("Board")
                            n254 = call "Board Calibrator.vi"("Board"=w640) -> ("ADC Table"=w643:T19[], "Suceeded"=w644:bool)  [unwired: 5 out]
                            n255 = Select(t=w643, s=w644, f=w642) -> (s? t:f=w641:T19[])
                          }
                          frame "Lens 1 without PS Test Points" {
                            w645 = T34 1 items=["Quad DC Board", "Lens 1 (Slot 8) Module", "Lens 2 (Slot 6) Module", "Detector Board", "Quad DC Board with Test Points", "Lens 1 Module with Test Points", "Len 2 Module with Test Points", "", "", "", "", ""] ("Board")
                            n256 = call "Board Calibrator.vi"("Board"=w645) -> ("ADC Table"=w648:T19[], "Suceeded"=w649:bool)  [unwired: 5 out]
                            n257 = Select(t=w648, s=w649, f=w647) -> (s? t:f=w646:T19[])
                          }
                          frame "Lens 1 with PS Test Points" {
                            w650 = T34 5 items=["Quad DC Board", "Lens 1 (Slot 8) Module", "Lens 2 (Slot 6) Module", "Detector Board", "Quad DC Board with Test Points", "Lens 1 Module with Test Points", "Len 2 Module with Test Points", "", "", "", "", ""] ("Board")
                            n258 = call "Board Calibrator.vi"("Board"=w650) -> ("ADC Table"=w653:T19[], "Suceeded"=w654:bool)  [unwired: 5 out]
                            n259 = Select(t=w653, s=w654, f=w652) -> (s? t:f=w651:T19[])
                          }
                          frame "Lens 2 without PS Test Points" {
                            w655 = T34 2 items=["Quad DC Board", "Lens 1 (Slot 8) Module", "Lens 2 (Slot 6) Module", "Detector Board", "Quad DC Board with Test Points", "Lens 1 Module with Test Points", "Len 2 Module with Test Points", "", "", "", "", ""] ("Board")
                            n260 = call "Board Calibrator.vi"("Board"=w655) -> ("ADC Table"=w658:T19[], "Suceeded"=w659:bool)  [unwired: 5 out]
                            n261 = Select(t=w658, s=w659, f=w657) -> (s? t:f=w656:T19[])
                          }
                          frame "Lens 2 with PS Test Points" {
                            w660 = T34 6 items=["Quad DC Board", "Lens 1 (Slot 8) Module", "Lens 2 (Slot 6) Module", "Detector Board", "Quad DC Board with Test Points", "Lens 1 Module with Test Points", "Len 2 Module with Test Points", "", "", "", "", ""] ("Board")
                            n262 = call "Board Calibrator.vi"("Board"=w660) -> ("ADC Table"=w663:T19[], "Suceeded"=w664:bool)  [unwired: 5 out]
                            n263 = Select(t=w663, s=w664, f=w662) -> (s? t:f=w661:T19[])
                          }
                          frame "Detector Board" {
                            w665 = T34 3 items=["Quad DC Board", "Lens 1 (Slot 8) Module", "Lens 2 (Slot 6) Module", "Detector Board", "Quad DC Board with Test Points", "Lens 1 Module with Test Points", "Len 2 Module with Test Points", "", "", "", "", ""] ("Board")
                            n264 = call "Board Calibrator.vi"("Board"=w665) -> ("ADC Table"=w668:T19[], "Suceeded"=w669:bool)  [unwired: 5 out]
                            n265 = Select(t=w668, s=w669, f=w667) -> (s? t:f=w666:T19[])
                          }
                          frame "Ion Spray Voltages" {
                            n266 = call "ISV Calibration.vi"("queue out"=w670) -> ("Channel Values"=w673:dbl[], "Suceeded"=w672:bool, "ADC Table"=w674:T19[])  [unwired: 4 in]
                            n267 = case shown="True" w672 {
                              tunnel: w671 -> [w676 _]
                              tunnel: [w676 w691] -> w675
                              tunnel: w674 -> [_ w691]
                              tunnel: w673 -> [_ w687]
                              frame False {
                              }
                              frame True {
                                w690 = 1 ("index (row)")
                                n268 = Index Array(array=w687) -> (element #1=w686:dbl, element #2=w680:dbl)  [unwired: 2 in]
                                n269 = local read "Corona/Curtain High Voltage"() -> (w685:string[][])
                                n270 = Format Into String(format string="%0.1f", w686) -> (resulting string=w688:string)  [unwired: 2 in, 1 out]
                                n271 = Format Into String(format string="%0.1f", w680) -> (resulting string=w679:string)  [unwired: 2 in, 1 out]
                                n272 = local read "Source Probes"() -> (w682:string[][])
                                n273 = Replace Array Subset(array=w685, new element=w688, index (row)=w690, index (col)=w690) -> (w684:string[][])
                                n274 = Replace Array Subset(array=w682, new element=w679, index (row)=0, index (col)=2 ("disabled index (col)")) -> (w678:string[][])
                                n275 = property on="Corona/Curtain High Voltage" class="Tbl (strict)"("Val(Sgnl)"=w684) -> ()  [unwired: 2 in, 2 out]
                                n276 = property on="Source Probes" class="Tbl (strict)"("Val(Sgnl)"=w678) -> ()  [unwired: 2 in, 2 out]
                              }
                            }
                          }
                          frame "Show Brief Status" {
                            n277 = call "_Launch Dynamic VI.vi"("VI Name"=path "Show Brief Status.vi" ("name or relative path")) -> ()  [unwired: 3 in, 1 out]
                          }
                          frame "Start System" {
                            n278 = call "_Remote Communicate.vi"("DC Param"=u16 0, "Command"=_RT_Command."Toggle Power") -> ("error out"=w695:errorcluster)  [unwired: 4 in, 3 out]
                            n279 = call <vilib>:"Simple Error Handler.vi"("error in (no error)"=w695) -> ()  [unwired: 1 in, 8 out]
                          }
                          frame "Goto Roughing Pump On Standby" {
                            n280 = call "_Remote Communicate.vi"("DC Param"=u16 1, "Command"=_RT_Command."Toggle Power") -> ("error out"=w699:errorcluster)  [unwired: 4 in, 3 out]
                            n281 = call <vilib>:"Simple Error Handler.vi"("error in (no error)"=w699) -> ()  [unwired: 1 in, 8 out]
                          }
                          frame "Shut Down System" {
                            n282 = call "_Remote Communicate.vi"("DC Param"=u16 2, "Command"=_RT_Command."Toggle Power") -> ("error out"=w703:errorcluster)  [unwired: 4 in, 3 out]
                            n283 = call <vilib>:"Simple Error Handler.vi"("error in (no error)"=w703) -> ()  [unwired: 1 in, 8 out]
                          }
                          frame "Update Methods" {
                            n284 = call "Update Methods.vi"() -> ()  [unwired: 12 in]
                          }
                          frame "Diagnostics Run" {
                            n285 = call "Auto Diagnotics Run.vi"() -> ()  [unwired: 8 in]
                          }
                          frame "Firmware Reboot" {
                            n286 = local read "MS State"() -> (w709:T1)
                            n287 = case shown="Default" w709 {
                              tunnel: [w720 TRUE ("T button?")] -> w708
                              frame Default {
                                n288 = Two Button Dialog(message="MS will have to be shutdown before performing a firmware reboot.", 2:"Continue" ("T button name (\"OK\")")) -> (T button?=w720:bool)  [unwired: 1 out]
                              }
                              frame "Mass Spectrometer is Off" {
                              }
                            }
                            n289 = case shown="True" w708 {
                              frame False {
                              }
                              frame True {
                                n290 = call "_Open Preference File.vi"() -> ("error"=w712:errorcluster, "refnum"=w713:T29)  [unwired: 3 in, 3 out]
                                n291 = call-poly <vilib>:"Read Key.vi"("section"="Lens", "error in (no error)"=w712, "default value"="172.16.0.2", "key"="IPAddress", "refnum"=w713) -> ("error out"=w714:errorcluster, "value"=w711:string, "refnum out"=w715:T29)  [unwired: 1 in, 3 out]
                                n292 = call "_Remote Reboot.vi"("IP Address"=w711) -> ()  [unwired: 1 in, 1 out]
                                n293 = call <vilib>:"Close Config Data.vi"("error in (no error)"=w714, "write file if changed (T)"=FALSE ("write configuration file? (F)"), "refnum"=w715) -> ()  [unwired: 9 out]
                              }
                            }
                          }
                          frame "Switch User" {
                            n294 = disable-structure shown="Disabled" {
                              disable-tunnel: [w729 w731] -> w726
                              disable-tunnel: [w728 w731] -> w724
                              frame Disabled {
                                n295 = call "Get Password.vi"("IonSniffer777"="ionics32") -> ("Advanced"=w728:bool, "Valid"=w729:bool)  [unwired: 5 out]
                              }
                              frame Enabled {
                                w731 = TRUE ("Advanced")
                              }
                            }
                            n296 = global write "_Global Configuration.vi" "Advanced"(w724) -> ()
                            n297 = property on="Options" class="Bool"("Visible"=w724) -> ()  [unwired: 2 in, 2 out]
                            n298 = property on="Edit ADC" class="Bool"("Visible"=w724) -> ()  [unwired: 2 in, 2 out]
                            n299 = property on="Edit Config" class="Bool"("Visible"=w724) -> ()  [unwired: 2 in, 2 out]
                            n300 = property on="FrequencyTuneSetup" class="Bool (strict)"("Visible"=w724) -> ()  [unwired: 2 in, 2 out]
                            n301 = case shown="True" w724 {
                              frame False {
                                n302 = Current VI's Menubar() -> (w733:refnum<k9>)
                                n303 = Delete Menu Items(7:"Direct DAC Control", 9:w733) -> ()  [unwired: 2 in, 2 out]
                              }
                              frame True {
                                w737 = "Direct DAC Control"
                                n304 = Current VI's Menubar() -> (w736:refnum<k9>)
                                n305 = Get Menu Item Info(7:w737, 11:w736) -> (1:w734:bool, 3:w735:refnum<k9>)  [unwired: 1 in, 5 out]
                                n306 = case shown="False" w734 {
                                tunnel: w737 -> [w739 _]
                                tunnel: w735 -> [w738 _]
                                frame False {
                                n307 = Insert Menu Items(8:w739, 9:w738) -> ()  [unwired: 4 in, 3 out]
                                }
                                frame True {
                                }
                                }
                              }
                            }
                            n308 = Not(x=w726) -> (.not. x?=w725:bool)
                            n309 = global write "_Global Configuration.vi" "Quit"(w725) -> ()
                          }
                          frame "Direct DAC Control" {
                            n310 = call "Direct DAC Control.vi"() -> ()  [unwired: 8 in]
                          }
                        }
                      }
                      frame True {
                      }
                    }
                    n311 = Bundle By Name(cluster=w596, "ADC Table"=w597) -> (w595:T32)
                  }
                  event "Run": Value Change {
                    w742 = u8 1 ("Disabled")
                    w748 = T35 2 items=["Diagnostics", "Tune", "Acquisition"] ("RunModule")
                    w743 = FALSE
                    n312 = event-data() -> ()  [unwired: 2 out]
                    n313 = Flush Queue(queue=w753) -> ()  [unwired: 1 in, 3 out]
                    n314 = local write "Running"("Run") -> ()
                    n315 = global write "_Global Configuration.vi" "RunModule"(w748) -> ()
                    n316 = property on="Run" class="Bool"("Visible"=FALSE) -> ()  [unwired: 2 in, 2 out]
                    n317 = property on="Cancel" class="Bool (strict)"("Visible"=TRUE) -> ()  [unwired: 2 in, 2 out]
                    n318 = property on="Detector" class="Tbl (strict)"("Disabled"=w742) -> ()  [unwired: 2 in, 2 out]
                    n319 = property on="Gas Flows" class="Tbl (strict)"("Disabled"=w742) -> ()  [unwired: 2 in, 2 out]
                    n320 = property on="Heaters" class="Tbl (strict)"("Disabled"=w742) -> ()  [unwired: 2 in, 2 out]
                    n321 = property on="Source Probes" class="Tbl (strict)"("Disabled"=w742) -> ()  [unwired: 2 in, 2 out]
                    n322 = property on="Corona/Curtain High Voltage" class="Tbl (strict)"("Disabled"=w742) -> ()  [unwired: 2 in, 2 out]
                    n323 = property on="Lens 1" class="Tbl (strict)"("Disabled"=w742) -> ()  [unwired: 2 in, 2 out]
                    n324 = property on="Lens 2" class="Tbl (strict)"("Disabled"=w742) -> ()  [unwired: 2 in, 2 out]
                    n325 = property on="Turbo OK" class="Bool (strict)"("Visible"=w743) -> ()  [unwired: 2 in, 2 out]
                    n326 = property on="SVG OK" class="Bool (strict)"("Visible"=w743) -> ()  [unwired: 2 in, 2 out]
                    n327 = property on="Intlk/Per OK" class="Bool (strict)"("Visible"=w743) -> ()  [unwired: 2 in, 2 out]
                    n328 = property on="Firmware OK" class="Bool (strict)"("Visible"=w743) -> ()  [unwired: 2 in, 2 out]
                    n329 = property on="Quad/Tune OK" class="Bool (strict)"("Visible"=w743) -> ()  [unwired: 2 in, 2 out]
                    n330 = property on="Voltage OK" class="Bool (strict)"("Visible"=w743) -> ()  [unwired: 2 in, 2 out]
                    n331 = property on="Progress Bar" class="Slide (strict)"("Visible"=TRUE) -> ()  [unwired: 2 in, 2 out]
                    n332 = Bundle By Name(cluster=w747, "Running"=TRUE) -> (w751:T32)
                    "Progress Bar" <- u8 0 ("ProgressBar")
                  }
                  event "Cancel": Value Change {
                    n333 = event-data() -> ()  [unwired: 7 out]
                    n334 = local write "Cancel"(FALSE ("Cancel")) -> ()
                    n335 = stacked-sequence {
                      tunnel: w758 -> [_ w763 _]
                      tunnel: [_ w763 _] -> w756
                      frame #0 {
                        w759 = u8 0 ("Disabled")
                        w760 = TRUE
                        w761 = FALSE ("Update")
                        n336 = property on="Detector" class="Tbl (strict)"("Disabled"=w759) -> ()  [unwired: 2 in, 2 out]
                        n337 = property on="Gas Flows" class="Tbl (strict)"("Disabled"=w759) -> ()  [unwired: 2 in, 2 out]
                        n338 = property on="Heaters" class="Tbl (strict)"("Disabled"=w759) -> ()  [unwired: 2 in, 2 out]
                        n339 = property on="Source Probes" class="Tbl (strict)"("Disabled"=w759) -> ()  [unwired: 2 in, 2 out]
                        n340 = property on="Corona/Curtain High Voltage" class="Tbl (strict)"("Disabled"=w759) -> ()  [unwired: 2 in, 2 out]
                        n341 = property on="Lens 1" class="Tbl (strict)"("Disabled"=w759) -> ()  [unwired: 2 in, 2 out]
                        n342 = property on="Lens 2" class="Tbl (strict)"("Disabled"=w759) -> ()  [unwired: 2 in, 2 out]
                        n343 = call <vilib>:"Set Busy.vi"() -> ()  [unwired: 4 in, 8 out]
                        n344 = global write "_Global Configuration.vi" "Run"(w761) -> ()
                        n345 = property on="Turbo OK" class="Bool (strict)"("Visible"=w760) -> ()  [unwired: 2 in, 2 out]
                        n346 = property on="SVG OK" class="Bool (strict)"("Visible"=w760) -> ()  [unwired: 2 in, 2 out]
                        n347 = property on="Intlk/Per OK" class="Bool (strict)"("Visible"=w760) -> ()  [unwired: 2 in, 2 out]
                        n348 = property on="Firmware OK" class="Bool (strict)"("Visible"=w760) -> ()  [unwired: 2 in, 2 out]
                        n349 = property on="Quad/Tune OK" class="Bool (strict)"("Visible"=w760) -> ()  [unwired: 2 in, 2 out]
                        n350 = property on="Voltage OK" class="Bool (strict)"("Visible"=w760) -> ()  [unwired: 2 in, 2 out]
                        n351 = property on="Progress Bar" class="Slide (strict)"("Visible"=FALSE) -> ()  [unwired: 2 in, 2 out]
                        "Running" <- w761
                      }
                      frame #1 {
                      }
                      frame #2 {
                        n352 = call "_Remote Park Lens.vi"() -> ()  [unwired: 2 in, 6 out]
                        n353 = call <vilib>:"Unset Busy.vi"() -> ()  [unwired: 2 in, 10 out]
                        n354 = property on="Run" class="Bool"("Visible"=TRUE) -> ()  [unwired: 2 in, 2 out]
                        n355 = property on="Cancel" class="Bool (strict)"("Visible"=FALSE) -> ()  [unwired: 2 in, 2 out]
                      }
                    }
                    n356 = Bundle By Name(cluster=w756, "Running"=FALSE) -> (w755:T32)
                  }
                  event "Load Firmware": Value Change {
                    n357 = event-data() -> ()  [unwired: 2 out]
                    n358 = Unbundle By Name(w768) -> ("Running"=w769:bool)
                    n359 = case shown="False" w769 {
                      frame False {
                        n360 = stacked-sequence {
                          seq-local: [_ w816 _] -> [_ _ w825]
                          seq-local: [_ w813 _] -> [_ _ w826]
                          seq-local: [w771 _ _] -> [_ w814 _]
                          seq-local: [w770 _ _] -> [_ _ w824]
                          frame #0 {
                            w784 = ""
                            w774 = "RT Controller Image Info" ("section")
                            # "Update Firmware from Files"
                            n361 = Current VI's Path() -> (path=w812:path)
                            n362 = Strip Path(path=w812) -> (stripped path=w811:path)  [unwired: 1 out]
                            n363 = Strip Path(path=w811) -> (stripped path=w810:path)  [unwired: 1 out]
                            n364 = call "File Dialog"("start path"=w810, "prompt"="Please choose a firmware image folder") -> ("selected path"=w770:path)  [unwired: 5 in, 8 out]
                            n365 = Build Path(base path=w770, name or relative path="RTCtrlr.ini") -> (appended path=w775:path)
                            n366 = call <vilib>:"Open Config Data.vi"("create file if necessary (T)"=FALSE ("create file if necessary? (T)"), "configuration file path"=w775) -> ("error out"=w807:errorcluster, "refnum"=w808:T29)  [unwired: 7 in, 1 out]
                            n367 = call-poly <vilib>:"Read Key.vi"("section"=w774, "error in (no error)"=w807, "default value"=w784, "key"="Model", "refnum"=w808) -> ("error out"=w804:errorcluster, "value"=w782:string, "refnum out"=w805:T29)  [unwired: 1 in, 3 out]
                            n368 = call-poly <vilib>:"Read Key.vi"("section"=w774, "error in (no error)"=w804, "default value"=w784, "key"="Image_Type", "refnum"=w805) -> ("error out"=w801:errorcluster, "value"=w781:string, "refnum out"=w802:T29)  [unwired: 1 in, 3 out]
                            n369 = call-poly <vilib>:"Read Key.vi"("section"=w774, "error in (no error)"=w801, "default value"=w784, "key"="MAC_Address", "refnum"=w802) -> ("error out"=w796:errorcluster, "value"=w778:string, "refnum out"=w797:T29)  [unwired: 1 in, 3 out]
                            n370 = call-poly <vilib>:"Read Key.vi"("section"=w774, "error in (no error)"=w796, "default value"=w784, "key"="Time", "refnum"=w797) -> ("error out"=w787:errorcluster, "value"=w780:string, "refnum out"=w788:T29)  [unwired: 1 in, 3 out]
                            n371 = call-poly <vilib>:"Read Key.vi"("section"=w774, "error in (no error)"=w787, "default value"=w784, "key"="IP_Address", "refnum"=w788) -> ("error out"=w785:errorcluster, "value"=w779:string, "refnum out"=w786:T29)  [unwired: 1 in, 3 out]
                            n372 = call-poly <vilib>:"Read Key.vi"("section"=w774, "error in (no error)"=w785, "default value"=w784, "key"="Host_Name", "refnum"=w786) -> ("error out"=w794:errorcluster, "value"=w777:string, "refnum out"=w795:T29)  [unwired: 1 in, 3 out]
                            n373 = call <vilib>:"Close Config Data.vi"("error in (no error)"=w794, "refnum"=w795) -> ("error out"=w798:errorcluster)  [unwired: 1 in, 8 out]
                            n374 = Format Into String(format string="Model: %s    Image: %s    Created: %s\nIP: %s     MAC: %s     Name: %s", error in=w798, w782, w781, w780, w779, w778, w777) -> (resulting string=w790:string, error out=w791:errorcluster)  [unwired: 1 in]
                            n375 = Unbundle By Name(w791) -> ("status"=w771:bool)
                            n376 = Select(t="Failed to load the backup files.\nPlease find a folder containing the firmware back-up files.", s=w771, f=w790) -> (s? t:f=→"Description":string)
                          }
                          frame #1 {
                            n377 = case shown="False" w814 {
                              selector: w814 -> [_ w823]
                              tunnel: [w820 w822] -> w813
                              frame False {
                                n378 = Two Button Dialog(message="The vacuum pumps will be shut off during firmware update.  Please press OK to continue.") -> (T button?=w820:bool)  [unwired: 2 out]
                              }
                              frame True {
                                n379 = Not(x=w823) -> (.not. x?=w822:bool)
                              }
                            }
                            n380 = global read "_Global Configuration.vi" "Configuration 2"() -> (w819:T18)
                            n381 = Unbundle By Name(w819) -> ("Instrument"=w818:string[])
                            n382 = Index Array(array=w818, index=7) -> (element=w817:string)
                            n383 = call <vilib>:"Trim Whitespace.vi"("string"=w817) -> ("trimmed string"=w816:string)  [unwired: 1 in]
                          }
                          frame #2 {
                            n384 = case shown="True" w826 {
                              tunnel: w825 -> [_ w828]
                              tunnel: w824 -> [_ w827]
                              frame False {
                              }
                              frame True {
                                # "Start firmware update"
                                n385 = stacked-sequence {
                                tunnel: w828 -> [_ w830 _]
                                tunnel: w827 -> [_ w832 _]
                                frame #0 {
                                n386 = call <vilib>:"Set Busy.vi"() -> ()  [unwired: 4 in, 8 out]
                                }
                                frame #1 {
                                w839 = ""
                                n387 = Bundle("trimmed string"=w830, w839, "selected path"=w832, "Source"=enum32{"RT Target", "Folder"}."Folder") -> (w835:T36)  [unwired: 1 out]
                                n388 = Bundle("trimmed string"=w830, w839, "selected path"=w832, "Source"=enum32{"RT Target", "Folder"}."RT Target") -> (w834:T36)  [unwired: 1 out]
                                n389 = call "_Remote RT Copy.vi"("Copy software only"=FALSE, "Image Destination"=w834, "Image Source"=w835) -> ("Error Out"=w831:errorcluster, "Messages"=→"Messages":string)  [unwired: 1 in, 4 out]
                                n390 = case shown="No Error" w831 {
                                selector: w831 -> [_ w841]
                                tunnel: [w840 w841] -> w829
                                frame No Error {
                                n391 = call "_Load Config File.vi"() -> ("error out"=w840:errorcluster)  [unwired: 2 in, 1 out]
                                }
                                frame Error {
                                }
                                }
                                n392 = call "_Handle Error.vi"("error in (no error)"=w829) -> ()  [unwired: 2 in, 5 out]
                                }
                                frame #2 {
                                n393 = call <vilib>:"Unset Busy.vi"() -> ()  [unwired: 2 in, 10 out]
                                }
                                }
                              }
                            }
                          }
                        }
                      }
                      frame True {
                      }
                    }
                    n394 = Bundle By Name(cluster=w768, "Update"=TRUE) -> (w767:T32)
                  }
                  event "Refresh": Value Change {
                    n395 = event-data() -> ()  [unwired: 2 out]
                    n396 = flat-sequence {
                      tunnel: [w847] -> w843
                      tunnel: w842 -> [w847]
                      tunnel: [w854] -> w844
                      tunnel: w843 -> [w854]
                      tunnel: [w894] -> w845
                      tunnel: w844 -> [w894]
                      frame #0 {
                        n397 = call <vilib>:"Set Busy.vi"() -> ()  [unwired: 4 in, 8 out]
                      }
                      frame #1 {
                        w891 = u32 200000000 ("y")
                        # "Firmware Check"
                        n398 = global read "_Global Configuration.vi" "Configuration 2"() -> (w890:T18)
                        n399 = Unbundle By Name(w890) -> ("Instrument"=w889:string[])
                        n400 = Wait (ms)(milliseconds to wait=u32 200) -> ()  [unwired: 1 out]
                        n401 = call "_Remote Communicate.vi"("Command"=_RT_Command."Get Info") -> ("Info"=w892:string)  [unwired: 5 in, 3 out]
                        n402 = Index Array(array=w889, index #1=0 ("index"), index #2=1 ("index"), index #3=2 ("index"), index #4=7 ("index")) -> (element #1=w878:string, element #2=w868:string, element #3=w864:string, element #4=w867:string)
                        n403 = Scan From String(format string="%s %s FPGA: %d; RT: %d; MEM: 2\n%[^,;]; FW:\\s%s ", input string=w892) -> (output 3=w850:i32, output 4=w849:i32, output 6=w848:string)  [unwired: 2 in, 12 out]
                        n404 = Greater?(x=w850, y=w891) -> (0:w874:bool)
                        n405 = Greater?(x=w849, y=w891) -> (0:w882:bool)
                        n406 = local write "Serial Number"(w868) -> ()
                        n407 = Number To Decimal String(number=w849) -> (decimal integer string=w852:string)  [unwired: 1 out]
                        n408 = Number To Decimal String(number=w850) -> (decimal integer string=w853:string)  [unwired: 1 out]
                        n409 = Empty String/Path?(string/path=w878) -> (empty?=w884:bool)
                        n410 = Empty String/Path?(string/path=w868) -> (empty?=w885:bool)
                        n411 = Empty String/Path?(string/path=w864) -> (empty?=w883:bool)
                        n412 = Empty String/Path?(string/path=w867) -> (empty?=w873:bool)
                        n413 = call "_Convert Model Name.vi"("Model"=w864) -> ("Model Name"=w865:T3)  [unwired: 1 in, 1 out]
                        n414 = local read "Current Information:"() -> (w877:string[][])
                        n415 = local write "Model Name"(w865) -> ()
                        n416 = Not(x=w884) -> (.not. x?=w881:bool)
                        n417 = Not(x=w885) -> (.not. x?=w880:bool)
                        n418 = Not(x=w883) -> (.not. x?=w879:bool)
                        n419 = Not(x=w873) -> (.not. x?=w872:bool)
                        n420 = Build Array(w848, w852, w853) -> (w875:string[])
                        n421 = Compound Arithmetic op=AND(w874, w882, w881, w880, w879, w872) -> (→"Firmware OK":bool)
                        n422 = call "_Open Preference File.vi"() -> ("error"=w857:errorcluster, "refnum"=w861:T29)  [unwired: 3 in, 3 out]
                        n423 = Replace Array Subset(array=w877, new element=w875, index (col)=1 ("disabled index (col)")) -> (→"Current Information:":string[][])  [unwired: 1 in]
                        n424 = call-poly <vilib>:"Read Key.vi"("section"="Lens", "error in (no error)"=w857, "default value"="172.16.0.2", "key"="IPAddress" ("section"), "refnum"=w861) -> ("error out"=w856:errorcluster, "value"=w855:string, "refnum out"=w858:T29)  [unwired: 1 in, 3 out]
                        n425 = local write "IP Address"(w855) -> ()
                        n426 = call <vilib>:"Close Config Data.vi"("error in (no error)"=w856, "write file if changed (T)"=FALSE ("write configuration file? (T)"), "refnum"=w858) -> ()  [unwired: 9 out]
                      }
                      frame #2 {
                        n427 = call <vilib>:"Unset Busy.vi"() -> ()  [unwired: 2 in, 10 out]
                      }
                    }
                    n428 = local write "Refresh"(FALSE ("Refresh")) -> ()
                  }
                  event "Header Info": Value Change {
                    n429 = event-data() -> ()  [unwired: 7 out]
                    n430 = local read "Serial Number"() -> (w898:string)
                    n431 = local read "Model Name"() -> (w899:T3)
                    n432 = call "Get Header Info.vi"("Model Name"=w899, "Serial Number"=w898) -> ("Model Name out"=→"Model Name":T3, "IP Address"=→"IP Address":string, "Serial Number out"=→"Serial Number":string)  [unwired: 3 out]
                    n433 = Bundle By Name(cluster=w896, "Update"=TRUE) -> (w895:T32)
                  }
                  event "GotoUPS": Value Change {
                    n434 = event-data() -> ()  [unwired: 2 out]
                    n435 = call-poly <vilib>:"Open URL in Default Browser.vi"("URL"="IP Address") -> ("error out"=w903:errorcluster, "URL out"=w904:string)  [unwired: 5 in]
                    n436 = local write "IP Address"(w904) -> ()
                    n437 = case shown="Error" w903 {
                      frame No Error {
                      }
                      frame Error {
                        n438 = One Button Dialog(message="Invalid address format.  \nTo fully ensure accuracy, please take the following steps:\n1. Open the web page in your default browser.\n2. Copy the command line from the address bar.\n3. Paste the path in Ionica Service Tool, and press \"Go to UPS\".") -> ()  [unwired: 1 in, 1 out]
                      }
                    }
                  }
                  event "SendSyringeCommand": Value Change {
                    n439 = event-data() -> ()  [unwired: 2 out]
                    n440 = Unbundle By Name(w909) -> ("Running"=w908:bool)
                    n441 = case shown="False" w908 {
                      frame False {
                        n442 = case shown="\"status\", Default" "Pump Command" {
                          tunnel: [u8 2 u8 3 u8 12 u8 13 u8 14 u8 17 u8 4 u8 5 u8 18 u8 6 u8 19 u8 11 u8 16 u8 15 u8 7] -> w913
                          frame "start" {
                          }
                          frame "stop" {
                          }
                          frame "pause" {
                          }
                          frame "restart" {
                          }
                          frame "help" {
                          }
                          frame "set units" {
                          }
                          frame "set diameter" {
                          }
                          frame "set rate" {
                          }
                          frame "set time" {
                          }
                          frame "set volume" {
                          }
                          frame "set delay" {
                          }
                          frame "save setting" {
                          }
                          frame "read limit parameter" {
                          }
                          frame "view parameter" {
                          }
                          frame "status", Default {
                          }
                        }
                        n443 = Format Into String(format string="%d,%f", w913, "Input Value") -> (resulting string=w910:string)  [unwired: 2 in, 1 out]
                        n444 = call "_Remote Communicate.vi"("String"=w910, "Command"=_RT_Command."Auxiliary Update") -> ("Info"=→"Return Data":string)  [unwired: 4 in, 3 out]
                      }
                      frame True {
                      }
                    }
                  }
                  event "VoltageInput": Value Change {
                    w942 = "Input"
                    w946 = 8 ("length")
                    n445 = event-data() -> ("NewVal"=w955:dbl[])  [unwired: 1 out]
                    n446 = Number To Fractional String(number=w955, precision (6)=i16 1) -> (F-format string=w947:string[])  [unwired: 2 out]
                    n447 = Array Subset(array=w947, index=0, length=w946) -> (w945:string[])
                    n448 = Array Subset(array=w947, index=w946, length=w946) -> (w944:string[])
                    n449 = Array Subset(array=w947, index=16, length=3) -> (w943:string[])
                    n450 = Build Array (concatenate)(w942, w945) -> (w933:string[])
                    n451 = Build Array (concatenate)(w942, w944) -> (w939:string[])
                    n452 = Build Array (concatenate)("", w943) -> (w941:string[])
                    n453 = Replace Array Subset(array="Lens 1", new element=w933, index (row)=1 ("disabled index (col)")) -> (w935:string[][])  [unwired: 1 in]
                    n454 = Replace Array Subset(array="Lens 2", new element=w939, index (row)=1 ("disabled index (col)")) -> (w940:string[][])  [unwired: 1 in]
                    n455 = Replace Array Subset(array="Detector", new element=w941, index (col)=1 ("disabled index (col)")) -> (w951:string[][])  [unwired: 1 in]
                    n456 = local write "Lens 1"(w935) -> ()
                    n457 = local write "Lens 2"(w940) -> ()
                    n458 = local write "Detector"(w951) -> ()
                  }
                  event "SG Input": Value Change {
                    # "EHSM-1864 - SX row should be removed"
                    # "EHSM-351 - Set SX to 0 - delete the SX entry"
                    n459 = event-data() -> ("NewVal"=w982:dbl[])  [unwired: 1 out]
                    n460 = Number To Fractional String(number=w982, precision (6)=i16 1) -> (F-format string=w971:string[])  [unwired: 2 out]
                    n461 = Split 1D Array(array=w971, index=7) -> (first subarray=w960:string[], second subarray=w969:string[])
                    n462 = Delete From Array(array=w960, length=1, index=5) -> (array with subset deleted=w959:string[])  [unwired: 1 out]
                    n463 = Replace Array Subset(array="Gas Flows", new element=w959, index (col)=2 ("disabled index (col)")) -> (w961:string[][])  [unwired: 1 in]
                    n464 = local write "Gas Flows"(w961) -> ()
                    n465 = Split 1D Array(array=w969, index=3) -> (first subarray=w963:string[], second subarray=w967:string[])
                    n466 = Replace Array Subset(array="Heaters", new element=w963, index (col)=2 ("disabled index (col)")) -> (w977:string[][])  [unwired: 1 in]
                    n467 = local write "Heaters"(w977) -> ()
                    n468 = Split 1D Array(array=w967, index=2) -> (first subarray=w964:string[], second subarray=w965:string[])
                    n469 = Replace Array Subset(array="Source Probes", new element=w964, index (col)=2 ("disabled index (col)")) -> (w962:string[][])  [unwired: 1 in]
                    n470 = local write "Source Probes"(w962) -> ()
                    n471 = Replace Array Subset(array="Corona/Curtain High Voltage", new element=w965, index (col)=1 ("disabled index (col)")) -> (w974:string[][])  [unwired: 1 in]
                    n472 = local write "Corona/Curtain High Voltage"(w974) -> ()
                  }
                  event "Detector": Value Change {
                    n473 = event-data() -> ("OldVal"=w985:string[][], "NewVal"=w986:string[][])  [unwired: 1 out]
                    n474 = Unbundle By Name(w988) -> ("Running"=w987:bool)
                    n475 = case shown="False" w987 {
                      tunnel: w986 -> [w999 _]
                      tunnel: w985 -> [_ w1001]
                      frame False {
                        w993 = 1 ("disabled index (col)")
                        n476 = Index Array(array=w999, index (col)=w993) -> (element=w996:string[])  [unwired: 1 in]
                        n477 = Array Subset(array=w996, index=w993, length=3) -> (w995:string[])
                        n478 = local read "VoltageInput"() -> (w992:dbl[])
                        n479 = Fract/Exp String To Number(string=w995) -> (number=w990:dbl[])  [unwired: 4 out]
                        n480 = Replace Array Subset(array=w992, new element=w990, index=16) -> (w989:dbl[])
                        n481 = local read "SG Input"() -> (w997:dbl[])
                        n482 = call "_Remote Set Voltages.vi"("Source/Gas"=w997, "UserValues"=w989) -> ("error out"=w998:errorcluster, "Voltages"=w1000:dbl[])  [unwired: 2 in, 2 out]
                        n483 = property on="VoltageInput" class="Arr (strict)"("Val(Sgnl)"=w1000) -> ()  [unwired: 2 in, 2 out]
                        n484 = call "_Handle Error.vi"("error in (no error)"=w998) -> ()  [unwired: 2 in, 5 out]
                      }
                      frame True {
                        n485 = local write "Detector"(w1001) -> ()
                      }
                    }
                  }
                  event "Lens 1": Value Change {
                    n486 = event-data() -> ("OldVal"=w1002:string[][], "NewVal"=w1003:string[][])  [unwired: 1 out]
                    n487 = Unbundle By Name(w1005) -> ("Running"=w1004:bool)
                    n488 = case shown="False" w1004 {
                      tunnel: w1003 -> [w1016 _]
                      tunnel: w1002 -> [_ w1018]
                      frame False {
                        w1006 = 1 ("disabled index (col)")
                        n489 = Index Array(array=w1016, index (row)=w1006) -> (element=w1013:string[])  [unwired: 1 in]
                        n490 = Array Subset(array=w1013, index=w1006, length=8) -> (w1012:string[])
                        n491 = local read "VoltageInput"() -> (w1010:dbl[])
                        n492 = Fract/Exp String To Number(string=w1012) -> (number=w1008:dbl[])  [unwired: 4 out]
                        n493 = Replace Array Subset(array=w1010, new element=w1008, index=0) -> (w1007:dbl[])
                        n494 = local read "SG Input"() -> (w1014:dbl[])
                        n495 = call "_Remote Set Voltages.vi"("Source/Gas"=w1014, "UserValues"=w1007) -> ("error out"=w1015:errorcluster, "Voltages"=w1017:dbl[])  [unwired: 2 in, 2 out]
                        n496 = property on="VoltageInput" class="Arr (strict)"("Val(Sgnl)"=w1017) -> ()  [unwired: 2 in, 2 out]
                        n497 = call "_Handle Error.vi"("error in (no error)"=w1015) -> ()  [unwired: 2 in, 5 out]
                      }
                      frame True {
                        n498 = local write "Lens 1"(w1018) -> ()
                      }
                    }
                  }
                  event "Lens 2": Value Change {
                    n499 = event-data() -> ("OldVal"=w1019:string[][], "NewVal"=w1020:string[][])  [unwired: 1 out]
                    n500 = Unbundle By Name(w1022) -> ("Running"=w1021:bool)
                    n501 = case shown="False" w1021 {
                      tunnel: w1020 -> [w1033 _]
                      tunnel: w1019 -> [_ w1035]
                      frame False {
                        w1023 = 1 ("disabled index (col)")
                        n502 = Index Array(array=w1033, index (row)=w1023) -> (element=w1030:string[])  [unwired: 1 in]
                        n503 = Array Subset(array=w1030, index=w1023, length=8) -> (w1029:string[])
                        n504 = local read "VoltageInput"() -> (w1027:dbl[])
                        n505 = Fract/Exp String To Number(string=w1029) -> (number=w1025:dbl[])  [unwired: 4 out]
                        n506 = Replace Array Subset(array=w1027, new element=w1025, index=8) -> (w1024:dbl[])
                        n507 = local read "SG Input"() -> (w1031:dbl[])
                        n508 = call "_Remote Set Voltages.vi"("Source/Gas"=w1031, "UserValues"=w1024) -> ("error out"=w1032:errorcluster, "Voltages"=w1034:dbl[])  [unwired: 2 in, 2 out]
                        n509 = property on="VoltageInput" class="Arr (strict)"("Val(Sgnl)"=w1034) -> ()  [unwired: 2 in, 2 out]
                        n510 = call "_Handle Error.vi"("error in (no error)"=w1032) -> ()  [unwired: 2 in, 5 out]
                      }
                      frame True {
                        n511 = local write "Lens 2"(w1035) -> ()
                      }
                    }
                  }
                  event "Gas Flows": Value Change {
                    n512 = event-data() -> ("OldVal"=w1036:string[][], "NewVal"=w1037:string[][])  [unwired: 1 out]
                    n513 = Unbundle By Name(w1039) -> ("Running"=w1038:bool)
                    n514 = case shown="False" w1038 {
                      tunnel: w1037 -> [w1054 _]
                      tunnel: w1036 -> [_ w1055]
                      frame False {
                        # "EHSM-351 - Set SX to 0 - add an entry for SX as 0"
                        n515 = Index Array(array=w1054, index (col)=2 ("disabled index (col)")) -> (element=w1052:string[])  [unwired: 1 in]
                        n516 = Fract/Exp String To Number(string=w1052) -> (number=w1041:dbl[])  [unwired: 4 out]
                        n517 = Insert Into Array(array=w1041, index=5, new element=0.0 ("new element/subarray")) -> (w1040:dbl[])
                        n518 = Reshape Array(w1040, 7 ("dimension size")) -> (w1043:dbl[])
                        n519 = local read "SG Input"() -> (w1048:dbl[])
                        n520 = local read "VoltageInput"() -> (w1049:dbl[])
                        n521 = Replace Array Subset(array=w1048, new element=w1043, index=0) -> (w1042:dbl[])
                        n522 = call "_Remote Set Voltages.vi"("Source/Gas"=w1042, "UserValues"=w1049) -> ("error out"=w1051:errorcluster, "Source/Gas Out"=w1050:dbl[])  [unwired: 2 in, 2 out]
                        n523 = property on="SG Input" class="Arr (strict)"("Val(Sgnl)"=w1050) -> ()  [unwired: 2 in, 2 out]
                        n524 = call "_Handle Error.vi"("error in (no error)"=w1051) -> ()  [unwired: 2 in, 5 out]
                      }
                      frame True {
                        n525 = local write "Gas Flows"(w1055) -> ()
                      }
                    }
                  }
                  event "Typical Gas Settings": Value Change {
                    n526 = event-data() -> ()  [unwired: 2 out]
                    n527 = Unbundle By Name(w1057) -> ("Running"=w1056:bool)
                    n528 = case shown="False" w1056 {
                      frame False {
                        n529 = global read "_Global Configuration.vi" "Single Source"() -> (w1061:bool)
                        n530 = local read "VoltageInput"() -> (w1065:dbl[])
                        n531 = local read "SG Input"() -> (w1064:dbl[])
                        n532 = Select(t=dbl[] [150.0, 200.0, 350.0, 0.0, 0.0, 0.0, 450.0] ("output array"), s=w1061, f=dbl[] [150.0, 200.0, 350.0, 200.0, 350.0, 0.0, 450.0] ("output array")) -> (s? t:f=w1059:dbl[])
                        n533 = Replace Array Subset(array=w1064, new element=w1059, index=0) -> (w1062:dbl[])
                        n534 = call "_Remote Set Voltages.vi"("Source/Gas"=w1062, "UserValues"=w1065) -> ("error out"=w1067:errorcluster, "Source/Gas Out"=w1066:dbl[])  [unwired: 2 in, 2 out]
                        n535 = property on="SG Input" class="Arr (strict)"("Val(Sgnl)"=w1066) -> ()  [unwired: 2 in, 2 out]
                        n536 = call "_Handle Error.vi"("error in (no error)"=w1067) -> ()  [unwired: 2 in, 5 out]
                      }
                      frame True {
                      }
                    }
                  }
                  event "Max Gas Settings": Value Change {
                    n537 = event-data() -> ()  [unwired: 2 out]
                    n538 = Unbundle By Name(w1069) -> ("Running"=w1068:bool)
                    n539 = case shown="False" w1068 {
                      frame False {
                        n540 = global read "_Global Configuration.vi" "Single Source"() -> (w1073:bool)
                        n541 = Select(t=dbl[] [300.0, 450.0, 350.0, 0.0, 0.0, 0.0, 500.0] ("output array"), s=w1073, f=dbl[] [300.0, 450.0, 350.0, 450.0, 350.0, 0.0, 500.0] ("output array")) -> (s? t:f=w1070:dbl[])
                        n542 = local read "VoltageInput"() -> (w1077:dbl[])
                        n543 = local read "SG Input"() -> (w1076:dbl[])
                        n544 = Replace Array Subset(array=w1076, new element=w1070, index=0) -> (w1074:dbl[])
                        n545 = call "_Remote Set Voltages.vi"("Source/Gas"=w1074, "UserValues"=w1077) -> ("error out"=w1079:errorcluster, "Source/Gas Out"=w1078:dbl[])  [unwired: 2 in, 2 out]
                        n546 = property on="SG Input" class="Arr (strict)"("Val(Sgnl)"=w1078) -> ()  [unwired: 2 in, 2 out]
                        n547 = call "_Handle Error.vi"("error in (no error)"=w1079) -> ()  [unwired: 2 in, 5 out]
                      }
                      frame True {
                      }
                    }
                  }
                  event "Min Gas Settings": Value Change {
                    n548 = event-data() -> ()  [unwired: 2 out]
                    n549 = Unbundle By Name(w1081) -> ("Running"=w1080:bool)
                    n550 = case shown="False" w1080 {
                      frame False {
                        n551 = local read "VoltageInput"() -> (w1086:dbl[])
                        n552 = local read "SG Input"() -> (w1085:dbl[])
                        n553 = Replace Array Subset(array=w1085, new element=dbl[] [30.0, 0.0, 0.0, 0.0, 0.0, 0.0, 0.0] ("output array"), index=0) -> (w1083:dbl[])
                        n554 = call "_Remote Set Voltages.vi"("Source/Gas"=w1083, "UserValues"=w1086) -> ("error out"=w1088:errorcluster, "Source/Gas Out"=w1087:dbl[])  [unwired: 2 in, 2 out]
                        n555 = property on="SG Input" class="Arr (strict)"("Val(Sgnl)"=w1087) -> ()  [unwired: 2 in, 2 out]
                        n556 = call "_Handle Error.vi"("error in (no error)"=w1088) -> ()  [unwired: 2 in, 5 out]
                      }
                      frame True {
                      }
                    }
                  }
                  event "Heaters": Value Change {
                    n557 = event-data() -> ("OldVal"=w1089:string[][], "NewVal"=w1090:string[][])  [unwired: 1 out]
                    n558 = Unbundle By Name(w1092) -> ("Running"=w1091:bool)
                    n559 = case shown="False" w1091 {
                      tunnel: w1090 -> [w1104 _]
                      tunnel: w1089 -> [_ w1106]
                      frame False {
                        n560 = Index Array(array=w1104, index (col)=2 ("disabled index (col)")) -> (element=w1102:string[])  [unwired: 1 in]
                        n561 = Fract/Exp String To Number(string=w1102) -> (number=w1097:dbl[])  [unwired: 4 out]
                        n562 = local read "VoltageInput"() -> (w1099:dbl[])
                        n563 = local read "SG Input"() -> (w1098:dbl[])
                        n564 = Reshape Array(w1097, 3 ("dimension size")) -> (w1095:dbl[])
                        n565 = Replace Array Subset(array=w1098, new element=w1095, index=7) -> (w1093:dbl[])
                        n566 = call "_Remote Set Voltages.vi"("Source/Gas"=w1093, "UserValues"=w1099) -> ("error out"=w1101:errorcluster, "Source/Gas Out"=w1100:dbl[], "Voltages"=w1105:dbl[])  [unwired: 2 in, 1 out]
                        n567 = property on="VoltageInput" class="Arr (strict)"("Val(Sgnl)"=w1105) -> ()  [unwired: 2 in, 2 out]
                        n568 = call "_Handle Error.vi"("error in (no error)"=w1101) -> ()  [unwired: 2 in, 5 out]
                        n569 = property on="SG Input" class="Arr (strict)"("Val(Sgnl)"=w1100) -> ()  [unwired: 2 in, 2 out]
                      }
                      frame True {
                        n570 = local write "Heaters"(w1106) -> ()
                      }
                    }
                  }
                  event "Source Probes": Value Change {
                    n571 = event-data() -> ("OldVal"=w1107:string[][], "NewVal"=w1108:string[][])  [unwired: 1 out]
                    n572 = Unbundle By Name(w1110) -> ("Running"=w1109:bool)
                    n573 = case shown="False" w1109 {
                      tunnel: w1108 -> [w1133 _]
                      tunnel: w1107 -> [_ w1135]
                      frame False {
                        w1115 = 0.0 ("t")
                        w1120 = T6 2 items=["None", "ESI", "APCI"] ("Source 1 Type:")
                        n574 = local read "Source 1 Type:"() -> (w1122:T6)
                        n575 = local read "Source 2 Type:"() -> (w1121:T6)
                        n576 = Index Array(array=w1133, index (col)=2 ("disabled index (col)")) -> (element=w1131:string[])  [unwired: 1 in]
                        n577 = Fract/Exp String To Number(string=w1131) -> (number=w1126:dbl[])  [unwired: 4 out]
                        n578 = Equal?(x=w1122, y=w1120) -> (x = y?=w1119:bool)
                        n579 = Equal?(x=w1120, y=w1121) -> (x = y?=w1117:bool)
                        n580 = local read "VoltageInput"() -> (w1128:dbl[])
                        n581 = local read "SG Input"() -> (w1127:dbl[])
                        n582 = Reshape Array(w1126, 2 ("dimension size")) -> (w1112:dbl[])
                        n583 = Index Array(array=w1112) -> (element #1=w1118:dbl, element #2=w1116:dbl)  [unwired: 2 in]
                        n584 = Select(t=w1115, s=w1117, f=w1116) -> (s? t:f=w1113:dbl)
                        n585 = Select(t=w1115, s=w1119, f=w1118) -> (s? t:f=w1114:dbl)
                        n586 = Build Array(w1114, w1113) -> (w1111:dbl[])
                        n587 = Replace Array Subset(array=w1127, new element=w1111, index=10) -> (w1123:dbl[])
                        n588 = call "_Remote Set Voltages.vi"("Source/Gas"=w1123, "UserValues"=w1128) -> ("error out"=w1130:errorcluster, "Source/Gas Out"=w1129:dbl[], "Voltages"=w1134:dbl[])  [unwired: 2 in, 1 out]
                        n589 = property on="VoltageInput" class="Arr (strict)"("Val(Sgnl)"=w1134) -> ()  [unwired: 2 in, 2 out]
                        n590 = call "_Handle Error.vi"("error in (no error)"=w1130) -> ()  [unwired: 2 in, 5 out]
                        n591 = property on="SG Input" class="Arr (strict)"("Val(Sgnl)"=w1129) -> ()  [unwired: 2 in, 2 out]
                      }
                      frame True {
                        n592 = local write "Source Probes"(w1135) -> ()
                      }
                    }
                  }
                  event "Corona/Curtain High Voltage": Value Change {
                    n593 = event-data() -> ("OldVal"=w1136:string[][], "NewVal"=w1137:string[][])  [unwired: 1 out]
                    n594 = Unbundle By Name(w1139) -> ("Running"=w1138:bool)
                    n595 = case shown="False" w1138 {
                      tunnel: w1137 -> [w1151 _]
                      tunnel: w1136 -> [_ w1153]
                      frame False {
                        n596 = Index Array(array=w1151, index (col)=1 ("disabled index (col)")) -> (element=w1149:string[])  [unwired: 1 in]
                        n597 = Fract/Exp String To Number(string=w1149) -> (number=w1144:dbl[])  [unwired: 4 out]
                        n598 = local read "VoltageInput"() -> (w1146:dbl[])
                        n599 = local read "SG Input"() -> (w1145:dbl[])
                        n600 = Reshape Array(w1144, 2 ("dimension size")) -> (w1142:dbl[])
                        n601 = Replace Array Subset(array=w1145, new element=w1142, index=12) -> (w1140:dbl[])
                        n602 = call "_Remote Set Voltages.vi"("Source/Gas"=w1140, "UserValues"=w1146) -> ("error out"=w1148:errorcluster, "Source/Gas Out"=w1147:dbl[], "Voltages"=w1152:dbl[])  [unwired: 2 in, 1 out]
                        n603 = property on="VoltageInput" class="Arr (strict)"("Val(Sgnl)"=w1152) -> ()  [unwired: 2 in, 2 out]
                        n604 = call "_Handle Error.vi"("error in (no error)"=w1148) -> ()  [unwired: 2 in, 5 out]
                        n605 = property on="SG Input" class="Arr (strict)"("Val(Sgnl)"=w1147) -> ()  [unwired: 2 in, 2 out]
                      }
                      frame True {
                        n606 = local write "Source Probes"(w1153) -> ()
                      }
                    }
                  }
                  event "Test Voltages": Value Change {
                    n607 = event-data() -> ()  [unwired: 2 out]
                    n608 = Unbundle By Name(w1155) -> ("Running"=w1154:bool)
                    n609 = case shown="False" w1154 {
                      frame False {
                        w1160 = T37 0 items=["Default", "Minimum", "Maximum", "Zero", "User"] ("VoltageType")
                        n610 = local read "SG Input"() -> (w1157:dbl[])
                        n611 = call "_Remote Set Voltages.vi"("Source/Gas"=w1157, "VoltageType"=w1160) -> ("error out"=w1159:errorcluster, "Source/Gas Out"=w1156:dbl[], "Voltages"=w1158:dbl[])  [unwired: 2 in, 1 out]
                        n612 = property on="VoltageInput" class="Arr (strict)"("Val(Sgnl)"=w1158) -> ()  [unwired: 2 in, 2 out]
                        n613 = property on="SG Input" class="Arr (strict)"("Val(Sgnl)"=w1156) -> ()  [unwired: 2 in, 2 out]
                        n614 = call "_Handle Error.vi"("error in (no error)"=w1159) -> ()  [unwired: 2 in, 5 out]
                      }
                      frame True {
                      }
                    }
                  }
                  event "Max Voltages": Value Change {
                    n615 = event-data() -> ()  [unwired: 2 out]
                    n616 = Unbundle By Name(w1162) -> ("Running"=w1161:bool)
                    n617 = case shown="False" w1161 {
                      frame False {
                        w1167 = T37 2 items=["Default", "Minimum", "Maximum", "Zero", "User"] ("VoltageType")
                        n618 = local read "SG Input"() -> (w1164:dbl[])
                        n619 = call "_Remote Set Voltages.vi"("Source/Gas"=w1164, "VoltageType"=w1167) -> ("error out"=w1166:errorcluster, "Source/Gas Out"=w1163:dbl[], "Voltages"=w1165:dbl[])  [unwired: 2 in, 1 out]
                        n620 = call "_Handle Error.vi"("error in (no error)"=w1166) -> ()  [unwired: 2 in, 5 out]
                        n621 = property on="SG Input" class="Arr (strict)"("Val(Sgnl)"=w1163) -> ()  [unwired: 2 in, 2 out]
                        n622 = property on="VoltageInput" class="Arr (strict)"("Val(Sgnl)"=w1165) -> ()  [unwired: 2 in, 2 out]
                      }
                      frame True {
                      }
                    }
                  }
                  event "Min Voltages": Value Change {
                    n623 = event-data() -> ()  [unwired: 2 out]
                    n624 = Unbundle By Name(w1169) -> ("Running"=w1168:bool)
                    n625 = case shown="False" w1168 {
                      frame False {
                        w1174 = T37 1 items=["Default", "Minimum", "Maximum", "Zero", "User"] ("VoltageType")
                        n626 = local read "SG Input"() -> (w1171:dbl[])
                        n627 = call "_Remote Set Voltages.vi"("Source/Gas"=w1171, "VoltageType"=w1174) -> ("error out"=w1173:errorcluster, "Source/Gas Out"=w1170:dbl[], "Voltages"=w1172:dbl[])  [unwired: 2 in, 1 out]
                        n628 = call "_Handle Error.vi"("error in (no error)"=w1173) -> ()  [unwired: 2 in, 5 out]
                        n629 = property on="SG Input" class="Arr (strict)"("Val(Sgnl)"=w1170) -> ()  [unwired: 2 in, 2 out]
                        n630 = property on="VoltageInput" class="Arr (strict)"("Val(Sgnl)"=w1172) -> ()  [unwired: 2 in, 2 out]
                      }
                      frame True {
                      }
                    }
                  }
                  event "Set 0 Values": Value Change {
                    n631 = event-data() -> ()  [unwired: 2 out]
                    n632 = Unbundle By Name(w1176) -> ("Running"=w1175:bool)
                    n633 = case shown="False" w1175 {
                      frame False {
                        w1181 = T37 3 items=["Default", "Minimum", "Maximum", "Zero", "User"] ("VoltageType")
                        n634 = local read "SG Input"() -> (w1178:dbl[])
                        n635 = call "_Remote Set Voltages.vi"("Source/Gas"=w1178, "VoltageType"=w1181) -> ("error out"=w1180:errorcluster, "Source/Gas Out"=w1177:dbl[], "Voltages"=w1179:dbl[])  [unwired: 2 in, 1 out]
                        n636 = call "_Handle Error.vi"("error in (no error)"=w1180) -> ()  [unwired: 2 in, 5 out]
                        n637 = property on="SG Input" class="Arr (strict)"("Val(Sgnl)"=w1177) -> ()  [unwired: 2 in, 2 out]
                        n638 = property on="VoltageInput" class="Arr (strict)"("Val(Sgnl)"=w1179) -> ()  [unwired: 2 in, 2 out]
                      }
                      frame True {
                      }
                    }
                  }
                  event "Load Tune File": Value Change {
                    n639 = event-data() -> ("NewVal"=w1186:bool)  [unwired: 1 out]
                    n640 = local write "Load Tune File"(FALSE ("Load Tune File")) -> ()
                    n641 = call "_Remote Set Method Voltages.vi"("use dialog? (F)"=w1186, "start path"="Tune File") -> ("error out"=w1185:errorcluster, "Source/Gas Out"=w1183:dbl[], "Voltages"=w1184:dbl[])  [unwired: 3 out]
                    n642 = case shown="No Error" w1185 {
                      tunnel: w1184 -> [w1190 _]
                      tunnel: w1183 -> [w1189 _]
                      frame No Error {
                        n643 = property on="VoltageInput" class="Arr (strict)"("Val(Sgnl)"=w1190) -> ()  [unwired: 2 in, 2 out]
                        n644 = property on="SG Input" class="Arr (strict)"("Val(Sgnl)"=w1189) -> ()  [unwired: 2 in, 2 out]
                      }
                      frame Error {
                      }
                    }
                  }
                  event "Load Default Method": Value Change {
                    n645 = event-data() -> ()  [unwired: 2 out]
                    n646 = property on="Load Tune File" class="Bool (strict)"("Val(Sgnl)"=FALSE ("Value (Signaling)")) -> ()  [unwired: 2 in, 2 out]
                    n647 = call <vilib>:"Application Directory.vi"() -> ("Application Directory"=w1191:path)
                    n648 = Build Path(base path=w1191, name or relative path="DEFAULT_SETTINGS.d2m") -> (appended path=w1194:path)
                    n649 = local write "Tune File"(w1194) -> ()
                  }
                  event "Switch Polarity": Value Change {
                    n650 = event-data() -> ()  [unwired: 2 out]
                    n651 = Unbundle By Name(w1197) -> ("Running"=w1196:bool)
                    n652 = case shown="False" w1196 {
                      frame False {
                        n653 = Split 1D Array(array="VoltageInput", index=16) -> (first subarray=w1201:dbl[], second subarray=w1200:dbl[])
                        n654 = Negate(x=w1201) -> (-x=w1199:dbl[])
                        n655 = Build Array (concatenate)(w1199, w1200) -> (w1198:dbl[])
                        n656 = call "_Remote Set Voltages.vi"("Source/Gas"="SG Input", "UserValues"=w1198) -> ("error out"=w1207:errorcluster, "Source/Gas Out"=w1204:dbl[], "Voltages"=w1206:dbl[])  [unwired: 2 in, 1 out]
                        n657 = property on="SG Input" class="Arr (strict)"("Val(Sgnl)"=w1204) -> ()  [unwired: 2 in, 2 out]
                        n658 = call "_Handle Error.vi"("error in (no error)"=w1207) -> ()  [unwired: 2 in, 5 out]
                        n659 = property on="VoltageInput" class="Arr (strict)"("Val(Sgnl)"=w1206) -> ()  [unwired: 2 in, 2 out]
                      }
                      frame True {
                      }
                    }
                  }
                  event "Pos/Neg", "Force Update Poles": Value Change {
                    n660 = event-data() -> ()  [unwired: 2 out]
                    n661 = Unbundle By Name(w1222) -> ("ADC Table"=w1221:T19[])
                    n662 = Unbundle By Name("Pole Swap Options Positive") -> ("Q1 B"=w1211:bool, "Q2 B"=w1210:bool)
                    n663 = Unbundle By Name("Pole Swap Options Negative") -> ("Q1 A"=w1209:bool, "Q2 A"=w1208:bool)
                    n664 = local write "Force Update Poles"(FALSE ("Force Update Poles")) -> ()
                    n665 = Equal?(x="Pos/Neg", y=enum32{"Positive", "Negative"}."Positive" ("Pos/Neg")) -> (x = y?=w1214:bool)
                    n666 = Build Array(w1211, w1210, w1209, w1208) -> (w1223:bool[])
                    n667 = call "_Update Oscillators.vi"("Pole In"=w1223, "ADC Table"=w1221, "Pole Swap (T)"=TRUE, "Update (T)"=FALSE, "Mode(pos)"=w1214, "Oscillator Settings"=w1226) -> ("Pole"=w1219:bool[])  [unwired: 2 in, 3 out]
                    n668 = call "Get Pole Orientations.vi"("Pole"=w1219) -> ("Pole Swap Options Negative"=w1217:T7, "Pole Swap Options Positive"=w1218:T7)  [unwired: 9 in]
                    n669 = local write "Pole Swap Options Positive"(w1218) -> ()
                    n670 = local write "Pole Swap Options Negative"(w1217) -> ()
                  }
                  event "Pole Swap Options Positive.Q1 A": Value Change {
                    n671 = event-data() -> ("NewVal"=w1231:bool)  [unwired: 1 out]
                    n672 = local read "Pole Swap Options Positive"() -> (w1228:T7)
                    n673 = Not(x=w1231) -> (.not. x?=w1230:bool)
                    n674 = Bundle By Name(cluster=w1228, "Q1 A"=w1231, "Q1 B"=w1230) -> (w1229:T7)
                    n675 = local write "Pole Swap Options Positive"(w1229) -> ()
                    n676 = property on="Force Update Poles" class="Bool (strict)"("Val(Sgnl)"=TRUE ("Value (Signaling)")) -> ()  [unwired: 2 in, 2 out]
                  }
                  event "Pole Swap Options Positive.Q1 B": Value Change {
                    n677 = event-data() -> ("NewVal"=w1237:bool)  [unwired: 1 out]
                    n678 = local read "Pole Swap Options Positive"() -> (w1234:T7)
                    n679 = Not(x=w1237) -> (.not. x?=w1236:bool)
                    n680 = Bundle By Name(cluster=w1234, "Q1 B"=w1237, "Q1 A"=w1236) -> (w1235:T7)
                    n681 = local write "Pole Swap Options Positive"(w1235) -> ()
                    n682 = property on="Force Update Poles" class="Bool (strict)"("Val(Sgnl)"=TRUE ("Value (Signaling)")) -> ()  [unwired: 2 in, 2 out]
                  }
                  event "Pole Swap Options Positive.Q2 A": Value Change {
                    n683 = event-data() -> ("NewVal"=w1243:bool)  [unwired: 1 out]
                    n684 = local read "Pole Swap Options Positive"() -> (w1240:T7)
                    n685 = Not(x=w1243) -> (.not. x?=w1242:bool)
                    n686 = Bundle By Name(cluster=w1240, "Q2 A"=w1243, "Q2 B"=w1242) -> (w1241:T7)
                    n687 = local write "Pole Swap Options Positive"(w1241) -> ()
                    n688 = property on="Force Update Poles" class="Bool (strict)"("Val(Sgnl)"=TRUE ("Value (Signaling)")) -> ()  [unwired: 2 in, 2 out]
                  }
                  event "Pole Swap Options Positive.Q2 B": Value Change {
                    n689 = event-data() -> ("NewVal"=w1249:bool)  [unwired: 1 out]
                    n690 = local read "Pole Swap Options Positive"() -> (w1246:T7)
                    n691 = Not(x=w1249) -> (.not. x?=w1248:bool)
                    n692 = Bundle By Name(cluster=w1246, "Q2 B"=w1249, "Q2 A"=w1248) -> (w1247:T7)
                    n693 = local write "Pole Swap Options Positive"(w1247) -> ()
                    n694 = property on="Force Update Poles" class="Bool (strict)"("Val(Sgnl)"=TRUE ("Value (Signaling)")) -> ()  [unwired: 2 in, 2 out]
                  }
                  event "Pole Swap Options Negative.Q1 A": Value Change {
                    n695 = event-data() -> ("NewVal"=w1255:bool)  [unwired: 1 out]
                    n696 = local read "Pole Swap Options Negative"() -> (w1251:T7)
                    n697 = Not(x=w1255) -> (.not. x?=w1254:bool)
                    n698 = Bundle By Name(cluster=w1251, "Q1 A"=w1255, "Q1 B"=w1254) -> (w1252:T7)
                    n699 = local write "Pole Swap Options Negative"(w1252) -> ()
                    n700 = property on="Force Update Poles" class="Bool (strict)"("Val(Sgnl)"=TRUE ("Value (Signaling)")) -> ()  [unwired: 2 in, 2 out]
                  }
                  event "Pole Swap Options Negative.Q1 B": Value Change {
                    n701 = event-data() -> ("NewVal"=w1261:bool)  [unwired: 1 out]
                    n702 = local read "Pole Swap Options Negative"() -> (w1257:T7)
                    n703 = Not(x=w1261) -> (.not. x?=w1260:bool)
                    n704 = Bundle By Name(cluster=w1257, "Q1 B"=w1261, "Q1 A"=w1260) -> (w1258:T7)
                    n705 = local write "Pole Swap Options Negative"(w1258) -> ()
                    n706 = property on="Force Update Poles" class="Bool (strict)"("Val(Sgnl)"=TRUE ("Value (Signaling)")) -> ()  [unwired: 2 in, 2 out]
                  }
                  event "Pole Swap Options Negative.Q2 A": Value Change {
                    n707 = event-data() -> ("NewVal"=w1267:bool)  [unwired: 1 out]
                    n708 = local read "Pole Swap Options Negative"() -> (w1263:T7)
                    n709 = Not(x=w1267) -> (.not. x?=w1266:bool)
                    n710 = Bundle By Name(cluster=w1263, "Q2 A"=w1267, "Q2 B"=w1266) -> (w1264:T7)
                    n711 = local write "Pole Swap Options Negative"(w1264) -> ()
                    n712 = property on="Force Update Poles" class="Bool (strict)"("Val(Sgnl)"=TRUE ("Value (Signaling)")) -> ()  [unwired: 2 in, 2 out]
                  }
                  event "Pole Swap Options Negative.Q2 B": Value Change {
                    n713 = event-data() -> ("NewVal"=w1273:bool)  [unwired: 1 out]
                    n714 = local read "Pole Swap Options Negative"() -> (w1269:T7)
                    n715 = Not(x=w1273) -> (.not. x?=w1272:bool)
                    n716 = Bundle By Name(cluster=w1269, "Q2 B"=w1273, "Q2 A"=w1272) -> (w1270:T7)
                    n717 = local write "Pole Swap Options Negative"(w1270) -> ()
                    n718 = property on="Force Update Poles" class="Bool (strict)"("Val(Sgnl)"=TRUE ("Value (Signaling)")) -> ()  [unwired: 2 in, 2 out]
                  }
                  event "Print": Value Change {
                    n719 = event-data() -> ()  [unwired: 2 out]
                    n720 = control-ref of="This VI"() -> (w1276:refnum<vi>)
                    n721 = Bundle By Name(cluster=T21 {"Picture Name"="", "VI Reference"=refnum} ("Cluster"), "Picture Name"="ServiceTool.jpg" ("name or relative path"), "VI Reference"=w1276) -> (w1275:T21)
                    n722 = Bundle By Name(cluster=cluster{"Command":string, "Data":variant} {"Command"="", "Data"=variant} ("element"), "Command"="Print", "Data"=w1275) -> (w1279:cluster{"Command":string, "Data":variant})
                    n723 = Enqueue Element(queue=w1282, element=w1279, error in (no error)=w1283) -> ()  [unwired: 1 in, 3 out]
                  }
                  event "Oscillator Settings": Value Change {
                    n724 = event-data() -> ()  [unwired: 7 out]
                    n725 = Unbundle By Name(w1286) -> ("ADC Table"=w1287:T19[])
                    n726 = stacked-sequence {
                      tunnel: w1288 -> [_ w1305 _]
                      tunnel: w1287 -> [_ w1302 _]
                      tunnel: w1286 -> [_ _ w1306]
                      tunnel: [_ _ w1307] -> w1285
                      frame #0 {
                        w1294 = 7 ("disabled index (col)")
                        # "copy the Q1RF input to Q2RF"
                        n727 = Index Array(array="Oscillator Settings", index (row)=1, index (col)=w1294) -> (element=w1292:string)
                        n728 = Replace Array Subset(array="Oscillator Settings", new element=w1292, index (row)=2, index (col)=w1294) -> (w1289:string[][])
                        n729 = local write "Oscillator Settings"(w1289) -> ()
                      }
                      frame #1 {
                        w1303 = TRUE ("Update (T)")
                        n730 = local read "Pos/Neg"() -> (w1297:enum32{"Positive", "Negative"})
                        n731 = Equal?(x=w1297, y=enum32{"Positive", "Negative"}."Positive" ("Pos/Neg")) -> (x = y?=w1295:bool)
                        n732 = call "_Update Oscillators.vi"("UpdateInput (F)"=w1303, "ADC Table"=w1302, "Pole Swap (T)"=FALSE, "Update (T)"=w1303, "Mode(pos)"=w1295, "Oscillator Settings"=w1305) -> ("Q1RF Frequency"=w1301:dbl, "Pole"=w1298:bool[])  [unwired: 2 in, 2 out]
                        n733 = local write "New Frequence"(w1301) -> ()
                        n734 = call "Get Pole Orientations.vi"("Pole"=w1298) -> ("Pole Swap Options Negative"=w1299:T7, "Pole Swap Options Positive"=w1300:T7)  [unwired: 9 in]
                        n735 = local write "Pole Swap Options Positive"(w1300) -> ()
                        n736 = local write "Pole Swap Options Negative"(w1299) -> ()
                      }
                      frame #2 {
                        n737 = Unbundle By Name(w1306) -> ("FrequencyTune"=w1308:bool)
                        n738 = case shown="True" w1308 {
                          tunnel: [w1309 w1312] -> w1307
                          tunnel: w1306 -> [w1309 w1313]
                          frame False {
                          }
                          frame True {
                            n739 = global read "_Global Configuration.vi" "Configuration 2"() -> (w1311:T18)
                            n740 = Unbundle By Name(w1311) -> ("Instrument"=w1310:string[])
                            n741 = Bundle By Name(cluster=w1313, "Configuration 2.Instrument"=w1310) -> (w1312:T32)
                          }
                        }
                      }
                    }
                  }
                  event "Force Update Oscillators": Value Change {
                    w1325 = FALSE ("Update (T)")
                    n742 = event-data() -> ()  [unwired: 2 out]
                    n743 = local write "Force Update Oscillators"(FALSE ("Force Update Poles")) -> ()
                    n744 = local read "Pos/Neg"() -> (w1317:enum32{"Positive", "Negative"})
                    n745 = call "_Remote Communicate.vi"("Command"=_RT_Command."Get ADC Table") -> ("error out"=w1324:errorcluster, "Info"=w1323:string)  [unwired: 5 in, 2 out]
                    n746 = Equal?(x=w1317, y=enum32{"Positive", "Negative"}."Positive" ("Pos/Neg")) -> (x = y?=w1315:bool)
                    n747 = Unflatten From String(type=T19[] [], binary string=w1323, error in (no error)=w1324) -> (value=w1321:T19[])  [unwired: 2 in, 2 out]
                    n748 = call "_Update Oscillators.vi"("UpdateInput (F)"=TRUE ("Pole Swap (T)"), "ADC Table"=w1321, "Pole Swap (T)"=w1325, "Update (T)"=w1325, "Mode(pos)"=w1315) -> ("Pole"=w1318:bool[])  [unwired: 4 in, 2 out]
                    n749 = Bundle By Name(cluster=w1327, "ADC Table"=w1321) -> (w1326:T32)
                    n750 = call "Get Pole Orientations.vi"("Pole"=w1318) -> ("Pole Swap Options Negative"=w1319:T7, "Pole Swap Options Positive"=w1320:T7)  [unwired: 9 in]
                    n751 = local write "Pole Swap Options Positive"(w1320) -> ()
                    n752 = local write "Pole Swap Options Negative"(w1319) -> ()
                  }
                  event "Q1 DC Inputs": Value Change {
                    n753 = event-data() -> ()  [unwired: 2 out]
                    n754 = call "_Remote Update DC.vi"("DC Inputs"="Q1 DC Inputs", "Table Reference"=w1332, "Ch#"=u8[] [4, 7, 6]) -> ("DC Outputs"=w1334:string[][], "Total"=→"Q1 Total":dbl, "VDC"=→"Q1 (VDC)":dbl)  [unwired: 2 out]
                    n755 = local write "Q1 DC Inputs"(w1334) -> ()
                  }
                  event "Q2 DC Inputs": Value Change {
                    n756 = event-data() -> ()  [unwired: 2 out]
                    n757 = call "_Remote Update DC.vi"("DC Inputs"="Q2 DC Inputs", "Table Reference"=w1339, "Ch#"=u8[] [5, 9, 8]) -> ("DC Outputs"=w1342:string[][], "Total"=→"Q2 Total":dbl, "VDC"=→"Q2 (VDC)":dbl)  [unwired: 2 out]
                    n758 = local write "Q2 DC Inputs"(w1342) -> ()
                  }
                  event "Turbo Update": Value Change {
                    n759 = event-data() -> ()  [unwired: 2 out]
                    n760 = Unbundle By Name(w1345) -> ("Running"=w1344:bool)
                    n761 = case shown="False" w1344 {
                      frame False {
                        n762 = stacked-sequence {
                          frame #0 {
                            n763 = call <vilib>:"Set Busy.vi"() -> ()  [unwired: 4 in, 8 out]
                          }
                          frame #1 {
                            w1346 = string[][] [] ("Error History")
                            n764 = local write "Pump Info:"(w1346) -> ()
                            n765 = local write "Error History"(w1346) -> ()
                            n766 = local write "Pumping:"(w1346) -> ()
                            n767 = local write "Power / Current:"(w1346) -> ()
                            n768 = local write "Temperatures:"(w1346) -> ()
                          }
                          frame #2 {
                            w1348 = TRUE
                            n769 = call "_Remote Get Turbo Status.vi"("Update Info"=w1348, "Update Temp"=w1348, "Update Error"=w1348, "Update Pumping"=w1348, "Update Power"=w1348) -> ("Power / Current:"=→"Power / Current:":string[][], "Turbo OK"=→"Turbo OK":bool, "Pump Info:"=→"Pump Info:":string[][], "Temperatures:"=→"Temperatures:":string[][], "Error History"=→"Error History":string[][], "Pumping:"=→"Pumping:":string[][])
                          }
                          frame #3 {
                            n770 = call <vilib>:"Unset Busy.vi"() -> ()  [unwired: 2 in, 10 out]
                          }
                        }
                      }
                      frame True {
                      }
                    }
                  }
                  event "LBFreqTemp": Value Change {
                    n771 = event-data() -> ()  [unwired: 2 out]
                    n772 = Unbundle By Name(w1356) -> ("Running"=w1355:bool)
                    n773 = case shown="False" w1355 {
                      frame False {
                        n774 = stacked-sequence {
                          frame #0 {
                            n775 = call <vilib>:"Set Busy.vi"() -> ()  [unwired: 4 in, 8 out]
                          }
                          frame #1 {
                            n776 = call "_Remote Get Leybold Status.vi"("UpdateOthers"=TRUE) -> ("OtherInfo"=w1370:T38, "Turbo OK"=w1357:bool)  [unwired: 5 in, 4 out]
                            n777 = local write "Turbo OK"(w1357) -> ()
                            n778 = Unbundle By Name(w1370) -> ("Frequency"=→"Frequency (Hz):":u16, "Decel"=→"Decel":bool, "Accel"=→"Accel":bool, "Normal \nOperation"=→"Normal \nOperation":bool, "Turning"=→"Turning":bool, "BearingTemp"=→"Bearing Temperature:":u32, "MotorTemp"=→"Moter Temperature:":u32, "ControllerTemp"=→"Controller Temperature:":u16, "PumpStatus"=→"PumpStatus":u16, "NumErrors"=→"Total Number of Errors:":u32, "NumOverload"=→"Number of Pressure Overload Errors:":u32, "NumFailure"=→"Number of Power Failures:":u32)
                          }
                          frame #2 {
                            n779 = call <vilib>:"Unset Busy.vi"() -> ()  [unwired: 2 in, 10 out]
                          }
                        }
                      }
                      frame True {
                      }
                    }
                    n780 = local write "LBFreqTemp"(FALSE ("LBFreqTemp")) -> ()
                  }
                  event "Update Info": Value Change {
                    n781 = event-data() -> ()  [unwired: 2 out]
                    n782 = Unbundle By Name(w1373) -> ("Running"=w1372:bool)
                    n783 = case shown="False" w1372 {
                      frame False {
                        n784 = stacked-sequence {
                          frame #0 {
                            n785 = call <vilib>:"Set Busy.vi"() -> ()  [unwired: 4 in, 8 out]
                          }
                          frame #1 {
                            n786 = local write "Pump Info:"(string[][] [] ("Error History")) -> ()
                          }
                          frame #2 {
                            n787 = call "_Remote Get Turbo Status.vi"("Update Info"=TRUE) -> ("Pump Info:"=w1375:string[][])  [unwired: 4 in, 5 out]
                            n788 = local write "Pump Info:"(w1375) -> ()
                          }
                          frame #3 {
                            n789 = call <vilib>:"Unset Busy.vi"() -> ()  [unwired: 2 in, 10 out]
                          }
                        }
                      }
                      frame True {
                      }
                    }
                  }
                  event "LBConfiguration": Value Change {
                    n790 = event-data() -> ()  [unwired: 2 out]
                    n791 = Unbundle By Name(w1378) -> ("Running"=w1377:bool)
                    n792 = case shown="False" w1377 {
                      frame False {
                        n793 = stacked-sequence {
                          frame #0 {
                            n794 = call <vilib>:"Set Busy.vi"() -> ()  [unwired: 4 in, 8 out]
                          }
                          frame #1 {
                            n795 = local write "Configuration:"(string[][] [] ("Error History")) -> ()
                          }
                          frame #2 {
                            n796 = call "_Remote Get Leybold Status.vi"("UpdateConfig"=TRUE) -> ("Configuration:"=→"Configuration:":string[][])  [unwired: 5 in, 5 out]
                          }
                          frame #3 {
                            n797 = call <vilib>:"Unset Busy.vi"() -> ()  [unwired: 2 in, 10 out]
                          }
                        }
                      }
                      frame True {
                      }
                    }
                  }
                  event "LBPower": Value Change {
                    n798 = event-data() -> ()  [unwired: 2 out]
                    n799 = Unbundle By Name(w1383) -> ("Running"=w1382:bool)
                    n800 = case shown="False" w1382 {
                      frame False {
                        n801 = stacked-sequence {
                          frame #0 {
                            n802 = call <vilib>:"Set Busy.vi"() -> ()  [unwired: 4 in, 8 out]
                          }
                          frame #1 {
                            n803 = local write "Power:"(string[][] [] ("Error History")) -> ()
                          }
                          frame #2 {
                            n804 = call "_Remote Get Leybold Status.vi"("UpdatePower"=TRUE) -> ("Power:"=→"Power:":string[][])  [unwired: 5 in, 5 out]
                          }
                          frame #3 {
                            n805 = call <vilib>:"Unset Busy.vi"() -> ()  [unwired: 2 in, 10 out]
                          }
                        }
                      }
                      frame True {
                      }
                    }
                  }
                  event "LBRunTime": Value Change {
                    n806 = event-data() -> ()  [unwired: 2 out]
                    n807 = Unbundle By Name(w1388) -> ("Running"=w1387:bool)
                    n808 = case shown="False" w1387 {
                      frame False {
                        n809 = stacked-sequence {
                          frame #0 {
                            n810 = call <vilib>:"Set Busy.vi"() -> ()  [unwired: 4 in, 8 out]
                          }
                          frame #1 {
                            n811 = local write "Run Time:"(string[][] [] ("Error History")) -> ()
                          }
                          frame #2 {
                            n812 = call "_Remote Get Leybold Status.vi"("UpdateRunTime"=TRUE) -> ("Run Time:"=→"Run Time:":string[][])  [unwired: 5 in, 5 out]
                          }
                          frame #3 {
                            n813 = call <vilib>:"Unset Busy.vi"() -> ()  [unwired: 2 in, 10 out]
                          }
                        }
                      }
                      frame True {
                      }
                    }
                  }
                  event "LBError": Value Change {
                    n814 = event-data() -> ()  [unwired: 2 out]
                    n815 = Unbundle By Name(w1393) -> ("Running"=w1392:bool)
                    n816 = case shown="False" w1392 {
                      frame False {
                        n817 = stacked-sequence {
                          frame #0 {
                            n818 = call <vilib>:"Set Busy.vi"() -> ()  [unwired: 4 in, 8 out]
                          }
                          frame #1 {
                            n819 = local write "Errors:"(string[][] [] ("Error History")) -> ()
                          }
                          frame #2 {
                            n820 = call "_Remote Get Leybold Status.vi"("UpdateError"=TRUE) -> ("Errors:"=→"Errors:":string[][])  [unwired: 5 in, 5 out]
                          }
                          frame #3 {
                            n821 = call <vilib>:"Unset Busy.vi"() -> ()  [unwired: 2 in, 10 out]
                          }
                        }
                      }
                      frame True {
                      }
                    }
                  }
                  event "LBUpdateAll": Value Change {
                    n822 = event-data() -> ()  [unwired: 2 out]
                    n823 = Unbundle By Name(w1398) -> ("Running"=w1397:bool)
                    n824 = case shown="False" w1397 {
                      frame False {
                        n825 = stacked-sequence {
                          frame #0 {
                            n826 = call <vilib>:"Set Busy.vi"() -> ()  [unwired: 4 in, 8 out]
                          }
                          frame #1 {
                            w1399 = string[][] [] ("Error History")
                            n827 = local write "Configuration:"(w1399) -> ()
                            n828 = local write "Power:"(w1399) -> ()
                            n829 = local write "Run Time:"(w1399) -> ()
                            n830 = local write "Errors:"(w1399) -> ()
                          }
                          frame #2 {
                            w1418 = TRUE
                            n831 = call "_Remote Get Leybold Status.vi"("UpdateError"=w1418, "UpdateRunTime"=w1418, "UpdatePower"=w1418, "UpdateOthers"=w1418, "UpdateConfig"=w1418) -> ("Run Time:"=w1414:string[][], "Power:"=w1415:string[][], "OtherInfo"=w1412:T38, "Configuration:"=w1416:string[][], "Turbo OK"=w1413:bool, "Errors:"=w1417:string[][])  [unwired: 1 in]
                            n832 = local write "Errors:"(w1417) -> ()
                            n833 = local write "Power:"(w1415) -> ()
                            n834 = local write "Turbo OK"(w1413) -> ()
                            n835 = local write "Run Time:"(w1414) -> ()
                            n836 = local write "Configuration:"(w1416) -> ()
                            n837 = Unbundle By Name(w1412) -> ("Frequency"=w1411:u16, "Decel"=w1410:bool, "Accel"=w1409:bool, "Normal \nOperation"=w1408:bool, "Turning"=w1407:bool, "BearingTemp"=w1406:u32, "MotorTemp"=w1405:u32, "ControllerTemp"=w1404:u16, "PumpStatus"=w1403:u16, "NumErrors"=w1402:u32, "NumOverload"=w1401:u32, "NumFailure"=w1400:u32)
                            n838 = local write "Frequency (Hz):"(w1411) -> ()
                            n839 = local write "Decel"(w1410) -> ()
                            n840 = local write "Accel"(w1409) -> ()
                            n841 = local write "Normal \nOperation"(w1408) -> ()
                            n842 = local write "Controller Temperature:"(w1404) -> ()
                            n843 = local write "PumpStatus"(w1403) -> ()
                            n844 = local write "Number of Pressure Overload Errors:"(w1401) -> ()
                            n845 = local write "Number of Power Failures:"(w1400) -> ()
                            n846 = local write "Turning"(w1407) -> ()
                            n847 = local write "Bearing Temperature:"(w1406) -> ()
                            n848 = local write "Moter Temperature:"(w1405) -> ()
                            n849 = local write "Total Number of Errors:"(w1402) -> ()
                          }
                          frame #3 {
                            n850 = call <vilib>:"Unset Busy.vi"() -> ()  [unwired: 2 in, 10 out]
                          }
                        }
                      }
                      frame True {
                      }
                    }
                  }
                  event "LBPump": Value Change {
                    n851 = event-data() -> ()  [unwired: 2 out]
                    n852 = Unbundle By Name(w1420) -> ("Running"=w1419:bool)
                    n853 = case shown="False" w1419 {
                      frame False {
                        n854 = stacked-sequence {
                          frame #0 {
                            n855 = call <vilib>:"Set Busy.vi"() -> ()  [unwired: 4 in, 8 out]
                          }
                          frame #1 {
                            w1424 = 1 ("disabled index (col)")
                            n856 = local read "Configuration:"() -> (w1427:string[][])
                            n857 = call "_Remote Get Leybold Status.vi"("UpdatePump"=TRUE) -> ("Configuration:"=w1430:string[][])  [unwired: 5 in, 5 out]
                            n858 = Index Array(array=w1430, index (col)=1 ("disabled index (col)")) -> (element=w1428:string[])  [unwired: 1 in]
                            n859 = Index Array(array=w1428) -> (element #1=w1423:string, element #2=w1422:string)  [unwired: 2 in]
                            n860 = Replace Array Subset(array=w1427, new element=w1423, index (row)=0, index (col)=w1424) -> (w1425:string[][])
                            n861 = Replace Array Subset(array=w1425, new element=w1422, index (row)=w1424, index (col)=w1424) -> (w1421:string[][])
                            n862 = local write "Configuration:"(w1421) -> ()
                          }
                          frame #2 {
                            n863 = call <vilib>:"Unset Busy.vi"() -> ()  [unwired: 2 in, 10 out]
                          }
                        }
                      }
                      frame True {
                      }
                    }
                  }
                  event "Update Pumping": Value Change {
                    n864 = event-data() -> ()  [unwired: 2 out]
                    n865 = Unbundle By Name(w1433) -> ("Running"=w1432:bool)
                    n866 = case shown="False" w1432 {
                      frame False {
                        n867 = stacked-sequence {
                          frame #0 {
                            n868 = call <vilib>:"Set Busy.vi"() -> ()  [unwired: 4 in, 8 out]
                          }
                          frame #1 {
                            n869 = local write "Pumping:"(string[][] [] ("Error History")) -> ()
                          }
                          frame #2 {
                            n870 = call "_Remote Get Turbo Status.vi"("Update Pumping"=TRUE) -> ("Turbo OK"=w1435:bool, "Pumping:"=w1436:string[][])  [unwired: 4 in, 4 out]
                            n871 = local write "Turbo OK"(w1435) -> ()
                            n872 = local write "Pumping:"(w1436) -> ()
                          }
                          frame #3 {
                            n873 = call <vilib>:"Unset Busy.vi"() -> ()  [unwired: 2 in, 10 out]
                          }
                        }
                      }
                      frame True {
                      }
                    }
                  }
                  event "Update Temp": Value Change {
                    n874 = event-data() -> ()  [unwired: 2 out]
                    n875 = Unbundle By Name(w1439) -> ("Running"=w1438:bool)
                    n876 = case shown="False" w1438 {
                      frame False {
                        n877 = stacked-sequence {
                          frame #0 {
                            n878 = call <vilib>:"Set Busy.vi"() -> ()  [unwired: 4 in, 8 out]
                          }
                          frame #1 {
                            n879 = local write "Temperatures:"(string[][] [] ("Error History")) -> ()
                          }
                          frame #2 {
                            n880 = call "_Remote Get Turbo Status.vi"("Update Temp"=TRUE) -> ("Temperatures:"=w1441:string[][])  [unwired: 4 in, 5 out]
                            n881 = local write "Temperatures:"(w1441) -> ()
                          }
                          frame #3 {
                            n882 = call <vilib>:"Unset Busy.vi"() -> ()  [unwired: 2 in, 10 out]
                          }
                        }
                      }
                      frame True {
                      }
                    }
                  }
                  event "Update Power": Value Change {
                    n883 = event-data() -> ()  [unwired: 2 out]
                    n884 = Unbundle By Name(w1444) -> ("Running"=w1443:bool)
                    n885 = case shown="False" w1443 {
                      frame False {
                        n886 = stacked-sequence {
                          frame #0 {
                            n887 = call <vilib>:"Set Busy.vi"() -> ()  [unwired: 4 in, 8 out]
                          }
                          frame #1 {
                            n888 = local write "Power / Current:"(string[][] [] ("Error History")) -> ()
                          }
                          frame #2 {
                            n889 = call "_Remote Get Turbo Status.vi"("Update Power"=TRUE) -> ("Power / Current:"=w1446:string[][])  [unwired: 4 in, 5 out]
                            n890 = local write "Power / Current:"(w1446) -> ()
                          }
                          frame #3 {
                            n891 = call <vilib>:"Unset Busy.vi"() -> ()  [unwired: 2 in, 10 out]
                          }
                        }
                      }
                      frame True {
                      }
                    }
                  }
                  event "Update Error": Value Change {
                    n892 = event-data() -> ()  [unwired: 2 out]
                    n893 = Unbundle By Name(w1449) -> ("Running"=w1448:bool)
                    n894 = case shown="False" w1448 {
                      frame False {
                        n895 = stacked-sequence {
                          frame #0 {
                            n896 = call <vilib>:"Set Busy.vi"() -> ()  [unwired: 4 in, 8 out]
                          }
                          frame #1 {
                            n897 = call "_Remote Send Turbo Command.vi"("Pump Command"=_Pump_Parameter."Clear Error") -> ()  [unwired: 2 in, 5 out]
                            n898 = local write "Error History"(string[][] [] ("Error History")) -> ()
                          }
                          frame #2 {
                            n899 = call "_Remote Get Turbo Status.vi"("Update Error"=TRUE) -> ("Error History"=w1452:string[][])  [unwired: 4 in, 5 out]
                            n900 = local write "Error History"(w1452) -> ()
                          }
                          frame #3 {
                            n901 = call <vilib>:"Unset Busy.vi"() -> ()  [unwired: 2 in, 10 out]
                          }
                        }
                      }
                      frame True {
                      }
                    }
                  }
                  event "Export ADC": Value Change {
                    n902 = event-data() -> ()  [unwired: 2 out]
                    n903 = call "_Get File.vi"("For Write (T)"=TRUE, "select mode (new or existing)"=T26."new or existing file", "default name"="My ADC Table", "extension (isd)"="*.txt" ("pattern (all files)"), "prompt"="Please enter an export file name.") -> ("Seleted File"=w1454:path, "Succeeded"=w1455:bool)  [unwired: 1 in, 2 out]
                    n904 = case shown="True" w1455 {
                      tunnel: w1454 -> [_ w1462]
                      frame False {
                      }
                      frame True {
                        n905 = property on="ADC List" class="MCListbox (strict)"() -> ("ItemNames"=w1463:string[][])  [unwired: 2 in, 2 out]
                        n906 = call "_Export Table To Text File.vi"("2D data"=w1463, "file path (dialog if empty)"=w1462) -> ()  [unwired: 4 in, 3 out]
                      }
                    }
                  }
                  event "Edit ADC": Value Change {
                    n907 = event-data() -> ()  [unwired: 2 out]
                    n908 = call "_Launch Dynamic VI.vi"("VI Name"=path "Show ADC Readings.vi" ("name or relative path")) -> ()  [unwired: 3 in, 1 out]
                  }
                  event "Edit Config": Value Change {
                    n909 = event-data() -> ()  [unwired: 7 out]
                    n910 = flat-sequence {
                      frame #0 {
                        n911 = call "Edit Configuration.vi"() -> ()  [unwired: 8 out]
                      }
                      frame #1 {
                        n912 = property on="Force Update Oscillators" class="Bool (strict)"("Val(Sgnl)"=TRUE ("Value (Signaling)")) -> ()  [unwired: 2 in, 2 out]
                      }
                    }
                  }
                  event "View Config": Value Change {
                    n913 = event-data() -> ()  [unwired: 2 out]
                    n914 = call "Configuration Viewer.vi"() -> ()  [unwired: 8 out]
                  }
                  event "Update PM", "M1RF": Value Change {
                    n915 = event-data() -> ()  [unwired: 2 out]
                    n916 = Unbundle By Name(w1470) -> ("Running"=w1469:bool)
                    n917 = case shown="False" w1469 {
                      frame False {
                        n918 = call "_Remote Park Mass.vi"("Q2 Park Mass"="Q2 Park Mass", "Q1 Park Mass"="Q1 Park Mass", "M1RF"="M1RF") -> ("error out"=w1473:errorcluster, "Q2 Park Mass Out"=w1474:dbl, "Q1 Park Mass Out"=w1475:dbl, "M1RF Out"=w1471:dbl)  [unwired: 1 in]
                        n919 = local write "Q2 Park Mass"(w1474) -> ()
                        n920 = local write "Q1 Park Mass"(w1475) -> ()
                        n921 = local write "M1RF"(w1471) -> ()
                        n922 = call "_Handle Error.vi"("error in (no error)"=w1473) -> ()  [unwired: 2 in, 5 out]
                      }
                      frame True {
                      }
                    }
                  }
                  event "FrequencyTuneSetup": Value Change {
                    n923 = event-data() -> ("NewVal"=w1478:bool)  [unwired: 1 out]
                    n924 = case shown="False" w1478 {
                      tunnel: w1480 -> [w1482 w1503]
                      tunnel: [w1483 w1502] -> w1479
                      frame False {
                        # "End Frequency Tuning"
                        n925 = flat-sequence {
                          tunnel: w1482 -> [w1484]
                          tunnel: [w1484] -> w1481
                          tunnel: [w1498] -> w1483
                          tunnel: w1481 -> [w1499]
                          frame #0 {
                            n926 = Current VI's Menubar() -> (w1485:refnum<k9>)
                            n927 = property on="Tab Control" class="TabCtl (strict)"("PageSelVis"=TRUE ("Page Selector Visible")) -> ()  [unwired: 2 in, 2 out]
                            n928 = Set Menu Item Info(7:"Save All Tables" ("item tag"), 9:TRUE ("enabled"), 11:w1485) -> (0:w1489:errorcluster, 3:w1488:refnum<k9>)  [unwired: 4 in]
                            n929 = Set Menu Item Info(7:"Load All Tables" ("item tag"), 8:w1489, 9:TRUE ("enabled"), 11:w1488) -> ()  [unwired: 3 in, 2 out]
                          }
                          frame #1 {
                            n930 = local read "M1RF"() -> (w1497:dbl)
                            n931 = Unbundle By Name(w1499) -> ("Configuration 2"=w1501:T18)
                            n932 = call "_Remote Park Mass.vi"("UseDefault (F)"=TRUE, "M1RF"=w1497) -> ("Q2 Park Mass Out"=w1494:dbl, "Q1 Park Mass Out"=w1493:dbl, "M1RF Out"=w1495:dbl)  [unwired: 2 in, 1 out]
                            n933 = Bundle By Name(cluster=w1499, "FrequencyTune"=FALSE) -> (w1498:T32)
                            n934 = global write "_Global Configuration.vi" "Configuration 2"(w1501) -> ()
                            n935 = local write "Q2 Park Mass"(w1494) -> ()
                            n936 = local write "Q1 Park Mass"(w1493) -> ()
                            n937 = local write "M1RF"(w1495) -> ()
                          }
                        }
                      }
                      frame True {
                        # "Start Frequency Tuning"
                        n938 = flat-sequence {
                          tunnel: w1503 -> [w1517]
                          tunnel: [w1516] -> w1506
                          tunnel: [w1515] -> w1505
                          tunnel: w1506 -> [w1518]
                          tunnel: w1505 -> [w1521]
                          tunnel: [w1518] -> w1504
                          tunnel: [w1534] -> w1502
                          tunnel: w1504 -> [w1544]
                          frame #0 {
                            n939 = global read "_Global Configuration.vi" "Configuration 2"() -> (w1515:T18)
                            n940 = Current VI's Menubar() -> (w1514:refnum<k9>)
                            n941 = Set Menu Item Info(7:"Save All Tables" ("item tag"), 9:FALSE ("enabled"), 11:w1514) -> (0:w1510:errorcluster, 3:w1511:refnum<k9>)  [unwired: 4 in]
                            n942 = Set Menu Item Info(7:"Load All Tables" ("item tag"), 8:w1510, 9:FALSE ("enabled"), 11:w1511) -> ()  [unwired: 3 in, 2 out]
                            n943 = Bundle By Name(cluster=w1517, "Configuration 2"=w1515) -> (w1516:T32)
                            n944 = property on="Tab Control" class="TabCtl (strict)"("PageSelVis"=FALSE ("Page Selector Visible")) -> ()  [unwired: 2 in, 2 out]
                          }
                          frame #1 {
                            n945 = Unbundle By Name(w1521) -> ("Table"=w1519:T19[])
                            n946 = for {
                              shift-right: [w1523] -> w1520
                              shift-left: w1519 -> [w1525]
                              tunnel: w1519 -> [_] mode=indexing
                              i -> [w1524]
                              n947 = in-place {
                                n948 = in-place-array #1(w1525, w1524) -> (w1527:T19)
                                n949 = Unbundle By Name(w1527) -> ("Name"=w1528:string)
                                n950 = case shown="\"M1 RF\", \"Q1 RF\", \"Q2 RF\"" w1528 {
                                tunnel: w1527 -> [w1529 w1532]
                                tunnel: [w1529 w1531] -> w1526
                                frame "False", Default {
                                }
                                frame "M1 RF", "Q1 RF", "Q2 RF" {
                                w1530 = 0.0 ("Def+")
                                n951 = Bundle By Name(cluster=w1532, "Def+"=w1530, "Def-"=w1530) -> (w1531:T19)
                                }
                                }
                                n952 = in-place-array #1(w1526) -> (w1523:T19[])  [unwired: 1 out]
                              }
                            }
                            n953 = Bundle By Name(cluster=w1521, "Table"=w1520) -> (w1522:T18)
                            n954 = global write "_Global Configuration.vi" "Configuration 2"(w1522) -> ()
                          }
                          frame #2 {
                            w1539 = 0.0 ("M1RF")
                            n955 = call "_Remote Park Mass.vi"("Q2 Park Mass"=w1539, "Q1 Park Mass"=w1539, "M1RF"=w1539) -> ("error out"=w1542:errorcluster, "Q2 Park Mass Out"=w1538:dbl, "Q1 Park Mass Out"=w1537:dbl, "M1RF Out"=w1536:dbl)  [unwired: 1 in]
                            n956 = local write "Q2 Park Mass"(w1538) -> ()
                            n957 = local write "Q1 Park Mass"(w1537) -> ()
                            n958 = local write "M1RF"(w1536) -> ()
                            n959 = local read "Oscillator Settings"() -> (w1535:string[][])
                            n960 = Bundle By Name(cluster=w1544, "FrequencyTune"=TRUE) -> (w1534:T32)
                            n961 = call "_Remote Communicate.vi"("error in (no error)"=w1542, "DC Param"=u16 0, "Command"=_RT_Command."Toggle Power") -> ("error out"=w1543:errorcluster)  [unwired: 3 in, 3 out]
                            n962 = property on="Oscillator Settings" class="Tbl (strict)"("Val(Sgnl)"=w1535) -> ()  [unwired: 2 in, 2 out]
                            n963 = call "_Handle Error.vi"("error in (no error)"=w1543) -> ()  [unwired: 2 in, 5 out]
                          }
                        }
                      }
                    }
                  }
                  event "Tab Control": Value Change {
                    n964 = event-data() -> ("OldVal"=w1555:T2)  [unwired: 1 out]
                    n965 = Unbundle By Name(w1546) -> ("Running"=w1553:bool, "Update"=w1552:bool)
                    n966 = Not Equal?(x=w1555, y=T27."QDC & Tuning" ("Tab Control")) -> (x != y?=w1550:bool)
                    n967 = Not(x=w1552) -> (.not. x?=w1551:bool)
                    n968 = And(x=w1551, y=w1550) -> (x .and. y?=w1549:bool)
                    n969 = case shown="Default" "Tab Control" {
                      frame Default {
                      }
                      frame "Leybold 3QS" {
                        n970 = property on="LBFreqTemp" class="Bool (strict)"("Val(Sgnl)"=TRUE ("Value (Signaling)")) -> ()  [unwired: 2 in, 2 out]
                      }
                      frame "Tables" {
                        n971 = property on="Table Choice" class="RadioBtnsControl (strict)"("Val(Sgnl)"="Table Choice") -> ()  [unwired: 2 in, 2 out]
                      }
                    }
                    n972 = Or(x=w1553, y=w1549) -> (x .or. y?=w1554:bool)
                    n973 = case shown="False" w1554 {
                      tunnel: w1546 -> [w1560 w1590]
                      tunnel: [w1559 w1590] -> w1545
                      frame False {
                        w1564 = 0 ("index (row)")
                        w1565 = string[][] [["400"], ["0"], ["0"]] ("Value (Signaling)")
                        n974 = flat-sequence {
                          tunnel: [w1577] -> w1558
                          tunnel: w1560 -> [w1577]
                          tunnel: [w1589] -> w1559
                          tunnel: w1558 -> [w1589]
                          frame #0 {
                            n975 = global read "_Global Configuration.vi" "Configuration 2"() -> (w1576:T18)
                            n976 = Unbundle By Name(w1576) -> ("Table"=w1575:T19[])
                            n977 = for {
                              tunnel: w1575 -> [w1579] mode=indexing
                              n978 = Unbundle By Name(w1579) -> ("Name"=w1580:string, "Def+"=w1578:dbl)
                              n979 = case shown="\"Q2 RF\"" w1580 {
                                tunnel: w1578 -> [_ w1581 w1582 w1583]
                                frame "False", Default {
                                }
                                frame "Q2 RF" {
                                (unwired) 0.0 ("Def+")
                                n980 = local write "Q2 Park Mass"(w1581) -> ()
                                }
                                frame "M1 RF" {
                                n981 = local write "M1RF"(w1582) -> ()
                                }
                                frame "Q1 RF" {
                                n982 = local write "Q1 Park Mass"(w1583) -> ()
                                }
                              }
                            }
                          }
                          frame #1 {
                            # "Reset the park mass to default"
                            n983 = local read "M1RF"() -> (w1588:dbl)
                            n984 = call "_Remote Park Mass.vi"("UseDefault (F)"=TRUE, "M1RF"=w1588) -> ("Q2 Park Mass Out"=w1585:dbl, "Q1 Park Mass Out"=w1584:dbl, "M1RF Out"=w1586:dbl)  [unwired: 2 in, 1 out]
                            n985 = local write "Q2 Park Mass"(w1585) -> ()
                            n986 = local write "Q1 Park Mass"(w1584) -> ()
                            n987 = local write "M1RF"(w1586) -> ()
                          }
                        }
                        n988 = call "_Get Lens Configuration.vi"("Channel #"=u8 4) -> ("Lens Configuration"=w1573:T19)  [unwired: 1 in, 5 out]
                        n989 = call "_Get Lens Configuration.vi"("Channel #"=u8 5) -> ("Lens Configuration"=w1572:T19)  [unwired: 1 in, 5 out]
                        n990 = Unbundle By Name(w1573) -> ("Def+"=w1570:dbl)
                        n991 = Unbundle By Name(w1572) -> ("Def+"=w1567:dbl)
                        n992 = Number To Fractional String(number=w1570, precision (6)=i16 0) -> (F-format string=w1566:string)  [unwired: 2 in]
                        n993 = Number To Fractional String(number=w1567, precision (6)=i16 0) -> (F-format string=w1563:string)  [unwired: 2 in]
                        n994 = Replace Array Subset(array=w1565, new element=w1566, index (row)=w1564, index (col)=w1564) -> (w1561:string[][])
                        n995 = Replace Array Subset(array=w1565, new element=w1563, index (row)=w1564, index (col)=w1564) -> (w1562:string[][])
                        n996 = property on="Q1 DC Inputs" class="Tbl (strict)"("Val(Sgnl)"=w1561) -> ()  [unwired: 2 in, 2 out]
                        n997 = property on="Q2 DC Inputs" class="Tbl (strict)"("Val(Sgnl)"=w1562) -> ()  [unwired: 2 in, 2 out]
                      }
                      frame True {
                      }
                    }
                  }
                  event "Options": Value Change {
                    w1592 = cluster{u32, u32}[] [{16711680, 16711680}, {10421504, 10421504}, {8323072, 8323072}, {5177856, 5177856}]  # RedColor
                    w1593 = cluster{u32, u32}[] [{12369084, 12369084}, {9868950, 9868950}, {12369084, 12369084}, {9868950, 9868950}]  # GrayColor
                    n998 = event-data() -> ()  [unwired: 2 out]
                    n999 = call "Start Up Options.vi"("No PW Needed (F)"=TRUE) -> ("All On"=w1594:bool)  [unwired: 6 out]
                    n1000 = Select(t=w1593, s=w1594, f=w1592) -> (s? t:f=w1591:cluster{u32, u32}[])
                    n1001 = property on="Options" class="Bool"("Colors [4]"=w1591) -> ()  [unwired: 2 in, 2 out]
                  }
                  event "Adjust Cal Tables": Value Change {
                    # "#EHSM-380: Remove useless boxes from QDC Tuning Tab"
                    n1002 = event-data() -> ()  [unwired: 2 out]
                    n1003 = disable-structure shown="Disabled" {
                      disable-tunnel: w1598 -> [w1601 w1621]
                      disable-tunnel: [w1600 w1621] -> w1597
                      frame Disabled {
                        n1004 = local read "New Frequence"() -> (w1603:dbl)
                        n1005 = local read "Old Frequency"() -> (w1604:dbl)
                        n1006 = Divide(x=w1603, y=w1604) -> (x/y=w1605:dbl)
                        n1007 = Square(x=w1605) -> (x^2=w1602:dbl)
                        n1008 = stacked-sequence {
                          tunnel: w1602 -> [w1608 w1611 w1614 w1617 _]
                          frame #0 {
                            n1009 = global read "_Global Configuration.vi" "Calibration"() -> (w1607:dbl[][])
                            n1010 = call "_Adjust Calibration Table.vi"("Calibration Table In"=w1607, "Adjustment Factor"=w1608) -> ("Calibration Table Out"=w1606:dbl[][])
                            n1011 = global write "_Global Configuration.vi" "Calibration"(w1606) -> ()
                          }
                          frame #1 {
                            n1012 = global read "_Global Configuration.vi" "Calibration 2"() -> (w1610:dbl[][])
                            n1013 = call "_Adjust Calibration Table.vi"("Calibration Table In"=w1610, "Adjustment Factor"=w1611) -> ("Calibration Table Out"=w1609:dbl[][])
                            n1014 = global write "_Global Configuration.vi" "Calibration 2"(w1609) -> ()
                          }
                          frame #2 {
                            n1015 = global read "_Global Configuration.vi" "Calibration 3"() -> (w1613:dbl[][])
                            n1016 = call "_Adjust Calibration Table.vi"("Calibration Table In"=w1613, "Adjustment Factor"=w1614) -> ("Calibration Table Out"=w1612:dbl[][])
                            n1017 = global write "_Global Configuration.vi" "Calibration 3"(w1612) -> ()
                          }
                          frame #3 {
                            n1018 = global read "_Global Configuration.vi" "Calibration 4"() -> (w1616:dbl[][])
                            n1019 = call "_Adjust Calibration Table.vi"("Calibration Table In"=w1616, "Adjustment Factor"=w1617) -> ("Calibration Table Out"=w1615:dbl[][])
                            n1020 = global write "_Global Configuration.vi" "Calibration 4"(w1615) -> ()
                          }
                          frame #4 {
                            n1021 = for {
                              N: 4 -> [_]
                              i -> [w1619]
                              n1022 = call "_Remote Communicate.vi"("DC Param"=w1619, "Command"=_RT_Command."Update Table") -> ()  [unwired: 4 in, 4 out]
                            }
                          }
                        }
                        n1023 = Bundle By Name(cluster=w1601, "CalAjusted"=TRUE) -> (w1600:T32)
                      }
                      frame Enabled {
                      }
                    }
                  }
                  event "Table Choice": Value Change {
                    n1024 = event-data() -> ("NewVal"=w1622:T8)  [unwired: 1 out]
                    n1025 = case shown="\"Low Resolution\"" w1622 {
                      tunnel: [w1632 w1633 w1634 w1635] -> w1623
                      frame "Calibration", Default {
                        w1632 = u16[] [0, 1, 2, 3] items=["Q1 +ve Mass Calibration Table", "Q2 +ve Mass Calibration Table", "Q1 -ve Mass Calibration Table", "Q2 -ve Mass Calibration Table", "Q1 +ve High Resolution Table", "Q2 +ve High Resolution Table", "Q1 +ve Medium Resolution Table", "Q2 +ve Medium Resolution Table", "Q1 +ve Low Resolution Table", "Q2 +ve Low Resolution Table", "Q1 -ve High Resolution Table", "Q2 -ve High Resolution Table", "Q1 -ve Medium Resolution Table", "Q2 -ve Medium Resolution Table", "Q1 -ve Low Resolution Table", "Q2 -ve Low Resolution Table"]
                      }
                      frame "Low Resolution" {
                        w1633 = u16[] [8, 9, 14, 15] items=["Q1 +ve Mass Calibration Table", "Q2 +ve Mass Calibration Table", "Q1 -ve Mass Calibration Table", "Q2 -ve Mass Calibration Table", "Q1 +ve High Resolution Table", "Q2 +ve High Resolution Table", "Q1 +ve Medium Resolution Table", "Q2 +ve Medium Resolution Table", "Q1 +ve Low Resolution Table", "Q2 +ve Low Resolution Table", "Q1 -ve High Resolution Table", "Q2 -ve High Resolution Table", "Q1 -ve Medium Resolution Table", "Q2 -ve Medium Resolution Table", "Q1 -ve Low Resolution Table", "Q2 -ve Low Resolution Table"]
                      }
                      frame "Unit Resolution" {
                        w1634 = u16[] [6, 7, 12, 13] items=["Q1 +ve Mass Calibration Table", "Q2 +ve Mass Calibration Table", "Q1 -ve Mass Calibration Table", "Q2 -ve Mass Calibration Table", "Q1 +ve High Resolution Table", "Q2 +ve High Resolution Table", "Q1 +ve Medium Resolution Table", "Q2 +ve Medium Resolution Table", "Q1 +ve Low Resolution Table", "Q2 +ve Low Resolution Table", "Q1 -ve High Resolution Table", "Q2 -ve High Resolution Table", "Q1 -ve Medium Resolution Table", "Q2 -ve Medium Resolution Table", "Q1 -ve Low Resolution Table", "Q2 -ve Low Resolution Table"]
                      }
                      frame "High Resolution" {
                        w1635 = u16[] [4, 5, 10, 11] items=["Q1 +ve Mass Calibration Table", "Q2 +ve Mass Calibration Table", "Q1 -ve Mass Calibration Table", "Q2 -ve Mass Calibration Table", "Q1 +ve High Resolution Table", "Q2 +ve High Resolution Table", "Q1 +ve Medium Resolution Table", "Q2 +ve Medium Resolution Table", "Q1 +ve Low Resolution Table", "Q2 +ve Low Resolution Table", "Q1 -ve High Resolution Table", "Q2 -ve High Resolution Table", "Q1 -ve Medium Resolution Table", "Q2 -ve Medium Resolution Table", "Q1 -ve Low Resolution Table", "Q2 -ve Low Resolution Table"]
                      }
                    }
                    n1026 = for {
                      tunnel: w1623 -> [w1627] mode=indexing
                      i -> [w1626]
                      n1027 = case shown="3" w1626 {
                        tunnel: [w1628 w1629 w1630 w1631] -> w1625
                        frame 0, Default {
                          n1028 = control-ref of="Table 1"() -> (w1628:refnum<vi>)
                        }
                        frame 1 {
                          n1029 = control-ref of="Table 2"() -> (w1629:refnum<vi>)
                        }
                        frame 2 {
                          n1030 = control-ref of="Table 3"() -> (w1630:refnum<vi>)
                        }
                        frame 3 {
                          n1031 = control-ref of="Table 4"() -> (w1631:refnum<vi>)
                        }
                      }
                      n1032 = call "_Display Calibration Table.vi"("Table Ref"=w1625, "Table Type"=w1627) -> ()  [unwired: 1 out]
                    }
                  }
                }
              }
              n1033 = while {
                shift-right: [w369] -> _
                shift-left: FALSE -> [w373]
                shift-right: [w367] -> _
                shift-left: w288 -> [w365]
                tunnel: w294 -> [w368]
                shift-left: w288 -> [w364]
                stop <- w370 stop-if-true
                n1034 = local read "Running"() -> (w374:bool)
                n1035 = local read "Quit"() -> (w371:bool)
                n1036 = global read "_Global Configuration.vi" "Quit"() -> (w372:bool)
                n1037 = Wait (ms)(milliseconds to wait=u32 280) -> ()  [unwired: 1 out]
                n1038 = Or(x=w372, y=w371) -> (x .or. y?=w370:bool)
                n1039 = case shown="False" w374 {
                  tunnel: w373 -> [w403 w418]
                  tunnel: w370 -> [w401 _]
                  tunnel: [w390 w418] -> w369
                  tunnel: [w398 w417] -> w367
                  tunnel: w365 -> [w399 w417]
                  tunnel: w368 -> [w392 _]
                  frame False {
                    n1040 = global read "_Global Configuration.vi" "Run"() -> (w402:bool)
                    n1041 = Or(x=w402, y=w401) -> (x .or. y?=w400:bool)
                    n1042 = case shown="False" w400 {
                      tunnel: w403 -> [w414 w416]
                      tunnel: [w413 w415] -> w398
                      tunnel: [w412 w416] -> w390
                      tunnel: w399 -> [_ w415]
                      frame False {
                        n1043 = call "_Remote Get RT Status.vi"("RT Ready"=w414) -> ("InstrState"=w413:T1, "RT Ready Out"=w412:bool)  [unwired: 1 in, 1 out]
                      }
                      frame True {
                      }
                    }
                    n1044 = global read "_Global Configuration.vi" "TCP"() -> (w393:bool)
                    n1045 = Select(t="- Connected", s=w393, f="- Simulation") -> (s? t:f=w407:string)
                    n1046 = Not Equal?(x=w398, y=w399) -> (x != y?=w396:bool)
                    n1047 = Equal?(x=w398, y=_RT_Instrument_State."Ready") -> (x = y?=w395:bool)
                    n1048 = Format Into String(format string=" %s, (state = %s)", initial string=w392, w407, w398) -> (resulting string=w391:string)  [unwired: 1 in, 1 out]
                    n1049 = And(x=w396, y=w395) -> (x .and. y?=w394:bool)
                    n1050 = case shown="True" w394 {
                      frame False {
                      }
                      frame True {
                        n1051 = property on="Load Tune File" class="Bool (strict)"("Val(Sgnl)"=FALSE ("Value (Signaling)")) -> ()  [unwired: 2 in, 2 out]
                        n1052 = call <vilib>:"Application Directory.vi"() -> ("Application Directory"=w408:path)
                        n1053 = Build Path(base path=w408, name or relative path="DEFAULT_SETTINGS.d2m") -> (appended path=w409:path)
                        n1054 = local write "Tune File"(w409) -> ()
                      }
                    }
                    n1055 = property class="VI"("Front Panel Window:Title"=w391) -> ()  [unwired: 2 in, 2 out]
                    n1056 = local write "Version"(w391) -> ()
                    n1057 = global write "_Global Configuration.vi" "RT Ready"(w390) -> ()
                  }
                  frame True {
                    # "Start Health Check Squence"
                    n1058 = stacked-sequence {
                      frame #0 {
                        n1059 = local write "Progress Bar"(u8 1 ("ProgressBar")) -> ()
                        n1060 = call <vilib>:"Application Directory.vi"() -> ("Application Directory"=w419:path)
                        n1061 = Build Path(base path=w419, name or relative path="TEST_ALL.d2m") -> (appended path=w422:path)
                        n1062 = local write "Tune File"(w422) -> ()
                      }
                      frame #1 {
                        n1063 = property on="Load Tune File" class="Bool (strict)"("Val(Sgnl)"=FALSE ("Value (Signaling)")) -> ()  [unwired: 2 in, 2 out]
                      }
                      frame #2 {
                        w425 = TRUE
                        # "Firmware Check"
                        n1064 = local read "Running"() -> (w424:bool)
                        n1065 = case shown="True" w424 {
                          tunnel: w425 -> [_ w428]
                          frame False {
                          }
                          frame True {
                            n1066 = property on="Refresh" class="Bool (strict)"("Val(Sgnl)"=w428) -> ()  [unwired: 2 in, 2 out]
                            n1067 = Wait (ms)(milliseconds to wait=u32 800) -> ()  [unwired: 1 out]
                          }
                        }
                        n1068 = property on="Firmware OK" class="Bool (strict)"("Visible"=w425) -> ()  [unwired: 2 in, 2 out]
                        n1069 = local write "Progress Bar"(u8 2 ("ProgressBar")) -> ()
                      }
                      frame #3 {
                        # "this was 2"
                        n1070 = local write "Progress Bar"(u8 14 ("ProgressBar")) -> ()
                        n1071 = local read "Running"() -> (w429:bool)
                        n1072 = case shown="True" w429 {
                          frame False {
                          }
                          frame True {
                            n1073 = global read "_Global Configuration.vi" "UseLeybold"() -> (w431:bool)
                            n1074 = case shown="False" w431 {
                              tunnel: TRUE -> [w433 w436]
                              frame False {
                                n1075 = call "_Remote Get Turbo Status.vi"("Update Info"=w433) -> ("Pump Info:"=w434:string[][])  [unwired: 4 in, 5 out]
                                n1076 = local write "Pump Info:"(w434) -> ()
                              }
                              frame True {
                                n1077 = call "_Remote Get Leybold Status.vi"("UpdateConfig"=w436) -> ("Configuration:"=w435:string[][])  [unwired: 5 in, 5 out]
                                n1078 = local write "Configuration:"(w435) -> ()
                              }
                            }
                          }
                        }
                      }
                      frame #4 {
                        # "this was 3"
                        n1079 = global read "_Global Configuration.vi" "UseLeybold"() -> (w440:bool)
                        n1080 = local write "Progress Bar"(u8 20 ("ProgressBar")) -> ()
                        n1081 = local read "Running"() -> (w438:bool)
                        n1082 = Not(x=w440) -> (.not. x?=w439:bool)
                        n1083 = And(x=w438, y=w439) -> (x .and. y?=w437:bool)
                        n1084 = case shown="True" w437 {
                          frame False {
                          }
                          frame True {
                            n1085 = call "_Remote Get Turbo Status.vi"("Update Pumping"=TRUE) -> ("Turbo OK"=w445:bool, "Pumping:"=w444:string[][])  [unwired: 4 in, 4 out]
                            n1086 = local write "Turbo OK"(w445) -> ()
                            n1087 = local write "Pumping:"(w444) -> ()
                          }
                        }
                        n1088 = property on="Turbo OK" class="Bool (strict)"("Visible"=TRUE) -> ()  [unwired: 2 in, 2 out]
                      }
                      frame #5 {
                        n1089 = global read "_Global Configuration.vi" "UseLeybold"() -> (w449:bool)
                        n1090 = local read "Running"() -> (w447:bool)
                        n1091 = local write "Progress Bar"(u8 35 ("ProgressBar")) -> ()
                        n1092 = Not(x=w449) -> (.not. x?=w448:bool)
                        n1093 = And(x=w447, y=w448) -> (x .and. y?=w446:bool)
                        n1094 = case shown="True" w446 {
                          frame False {
                          }
                          frame True {
                            n1095 = call "_Remote Get Turbo Status.vi"("Update Temp"=TRUE) -> ("Temperatures:"=w452:string[][])  [unwired: 4 in, 5 out]
                            n1096 = local write "Temperatures:"(w452) -> ()
                          }
                        }
                      }
                      frame #6 {
                        n1097 = global read "_Global Configuration.vi" "UseLeybold"() -> (w456:bool)
                        n1098 = local read "Running"() -> (w454:bool)
                        n1099 = local write "Progress Bar"(u8 40 ("ProgressBar")) -> ()
                        n1100 = Not(x=w456) -> (.not. x?=w455:bool)
                        n1101 = And(x=w454, y=w455) -> (x .and. y?=w453:bool)
                        n1102 = case shown="True" w453 {
                          frame False {
                          }
                          frame True {
                            n1103 = call "_Remote Get Turbo Status.vi"("Update Power"=TRUE) -> ("Power / Current:"=w459:string[][])  [unwired: 4 in, 5 out]
                            n1104 = local write "Power / Current:"(w459) -> ()
                          }
                        }
                      }
                      frame #7 {
                        n1105 = local read "Running"() -> (w461:bool)
                        n1106 = global read "_Global Configuration.vi" "UseLeybold"() -> (w460:bool)
                        n1107 = local write "Progress Bar"(u8 65 ("ProgressBar")) -> ()
                        n1108 = case shown="True" w461 {
                          tunnel: w460 -> [_ w463]
                          frame False {
                          }
                          frame True {
                            n1109 = case shown="True" w463 {
                              frame False {
                                n1110 = call "_Remote Get Turbo Status.vi"("Update Error"=TRUE) -> ("Error History"=w465:string[][])  [unwired: 4 in, 5 out]
                                n1111 = local write "Error History"(w465) -> ()
                              }
                              frame True {
                                w466 = TRUE
                                n1112 = call "_Remote Get Leybold Status.vi"("UpdateError"=w466, "UpdateRunTime"=w466, "UpdatePower"=w466, "UpdateOthers"=w466) -> ("Run Time:"=w481:string[][], "Power:"=w482:string[][], "OtherInfo"=w479:T38, "Turbo OK"=w480:bool, "Errors:"=w483:string[][])  [unwired: 2 in, 1 out]
                                n1113 = local write "Errors:"(w483) -> ()
                                n1114 = local write "Power:"(w482) -> ()
                                n1115 = local write "Run Time:"(w481) -> ()
                                n1116 = local write "Turbo OK"(w480) -> ()
                                n1117 = Unbundle By Name(w479) -> ("Frequency"=w478:u16, "Decel"=w477:bool, "Accel"=w476:bool, "Normal \nOperation"=w475:bool, "Turning"=w474:bool, "BearingTemp"=w473:u32, "MotorTemp"=w472:u32, "ControllerTemp"=w471:u16, "PumpStatus"=w470:u16, "NumErrors"=w469:u32, "NumOverload"=w468:u32, "NumFailure"=w467:u32)
                                n1118 = local write "Frequency (Hz):"(w478) -> ()
                                n1119 = local write "Decel"(w477) -> ()
                                n1120 = local write "Accel"(w476) -> ()
                                n1121 = local write "Normal \nOperation"(w475) -> ()
                                n1122 = local write "Controller Temperature:"(w471) -> ()
                                n1123 = local write "PumpStatus"(w470) -> ()
                                n1124 = local write "Number of Pressure Overload Errors:"(w468) -> ()
                                n1125 = local write "Number of Power Failures:"(w467) -> ()
                                n1126 = local write "Turning"(w474) -> ()
                                n1127 = local write "Bearing Temperature:"(w473) -> ()
                                n1128 = local write "Moter Temperature:"(w472) -> ()
                                n1129 = local write "Total Number of Errors:"(w469) -> ()
                              }
                            }
                          }
                        }
                      }
                      frame #8 {
                        w484 = TRUE
                        # "SVG Check"
                        # "Voltage Check"
                        n1130 = local write "Progress Bar"(u8 70 ("ProgressBar")) -> ()
                        n1131 = property on="SVG OK" class="Bool (strict)"("Visible"=w484) -> ()  [unwired: 2 in, 2 out]
                        n1132 = property on="Voltage OK" class="Bool (strict)"("Visible"=w484) -> ()  [unwired: 2 in, 2 out]
                      }
                      frame #9 {
                        # "Interlock Check"
                        n1133 = local write "Progress Bar"(u8 75 ("ProgressBar")) -> ()
                        n1134 = property on="Intlk/Per OK" class="Bool (strict)"("Visible"=TRUE) -> ()  [unwired: 2 in, 2 out]
                      }
                      frame #10 {
                        # "Done Quad Check"
                        n1135 = local write "Progress Bar"(u8 95 ("ProgressBar")) -> ()
                        n1136 = property on="Quad/Tune OK" class="Bool (strict)"("Visible"=TRUE) -> ()  [unwired: 2 in, 2 out]
                      }
                      frame #11 {
                        # "Finish Run"
                        n1137 = local write "Running"(FALSE ("Unit")) -> ()
                        n1138 = property on="Cancel" class="Bool (strict)"("Val(Sgnl)"=TRUE ("Value (Signaling)")) -> ()  [unwired: 2 in, 2 out]
                        n1139 = local write "Progress Bar"(u8 100 ("ProgressBar")) -> ()
                      }
                    }
                  }
                }
                "MS State" <- w367
                n1140 = Not Equal?(x=w365, y=w364) -> (x != y?=w366:bool)
                n1141 = global write "_Global Configuration.vi" "MS State"(w367) -> ()
                n1142 = case shown="True" w366 {
                  tunnel: w365 -> [_ w383]
                  frame False {
                  }
                  frame True {
                    n1143 = Equal?(x=w383, y=_RT_Instrument_State."Ready") -> (x = y?=w379:bool)
                    n1144 = Equal?(x=w383, y=_RT_Instrument_State."Mass Spectrometer is Off") -> (x = y?=w380:bool)
                    n1145 = Current VI's Menubar() -> (w376:refnum<k9>)
                    n1146 = Or(x=w379, y=w380) -> (x .or. y?=w378:bool)
                    n1147 = case shown="False" w378 {
                      tunnel: "Goto Roughing Pump On Standby" ("item name") -> [w386 w389]
                      tunnel: w376 -> [w385 w388]
                      frame True {
                        n1148 = Set Menu Item Info(7:w386, 9:TRUE ("enabled"), 11:w385) -> ()  [unwired: 4 in, 2 out]
                      }
                      frame False {
                        n1149 = Set Menu Item Info(7:w389, 9:FALSE ("enabled"), 11:w388) -> ()  [unwired: 4 in, 2 out]
                      }
                    }
                  }
                }
              }
              n1150 = while {
                tunnel: w293 -> [w315]
                tunnel: w290 -> [w316]
                tunnel: [w312] -> w292
                tunnel: [w311] -> w291
                stop <- w317 stop-if-true
                # "Command Q"
                n1151 = Dequeue Element(queue=w315, timeout in ms (-1)=280, error in (no error)=w316) -> (queue out=w311:refnum<queue>, element=w314:cluster{"Command":string, "Data":variant}, timed out?=w310:bool, error out=w309:errorcluster)
                n1152 = Or(x=w309, y=w310) -> (x .or. y?=w308:bool)
                n1153 = case shown="False" w308 {
                  tunnel: w309 -> [w321 w363]
                  tunnel: w314 -> [w324 _]
                  tunnel: [w320 w363] -> w312
                  frame False {
                    # "New Command"
                    n1154 = Unbundle(w324) -> ("Command"=w322:string, "Data"=w323:variant)
                    n1155 = case shown="\"Print\"" w322 {
                      tunnel: w323 -> [_ w336]
                      tunnel: w321 -> [w325 w353]
                      tunnel: [w325 w340] -> w320
                      frame Default {
                        # "unknown command"
                      }
                      frame "Print" {
                        w345 = 1 items=["portrait", "landscape"] ("orientation (portrait)")
                        # "the report generation Quick print causes the VI to freeze while the screenshot is taken\nwhich causes a FW dropped connection. Getting a scaled image here, and passing it to the report generation\nneed a scaled image as report generator is not scaling the image properly"
                        # "Print Command"
                        n1156 = Variant To Data(error in=w353, type=T21 {"Picture Name"="", "VI Reference"=refnum} ("Cluster"), Variant=w336) -> (data=w335:T21, error out=w338:errorcluster)
                        n1157 = Unbundle By Name(w335) -> ("Picture Name"=w334:string, "VI Reference"=w333:refnum<vi>)
                        n1158 = invoke class="VI" method="FP.Get Image Scaled"(reference=w333, "visible area only"=TRUE ("Visible Area Only"), "max width"=1100 ("Maximum Width"), "max height"=579 ("Maximum Height")) -> ("image data"=w354:T39)  [unwired: 4 in, 7 out]
                        n1159 = call <vilib>:"Application Directory.vi"() -> ("Application Directory"=w352:path)
                        n1160 = Build Path(base path=w352, name or relative path=w334) -> (appended path=w351:path)
                        n1161 = call <vilib>:"Write JPEG File.vi"("error in (no error)"=w338, "image data"=w354, "path to JPEG file"=w351) -> ("error out"=w342:errorcluster, "path"=w339:path)  [unwired: 7 out]
                        n1162 = call <vilib>:"New Report.vi"("report type"=T22."Standard Report", "error in (no error)"=w342) -> ("report out"=w346:refnum<class "NI_report.lvclass">, "error out"=w349:errorcluster)  [unwired: 12 in]
                        n1163 = call-dynamic "Set Report Orientation.vi"("report in"=w346, "orientation (portrait)"=w345, "error in (no error)"=w349) -> ("report out"=w348:refnum<class "NI_report.lvclass">, "error out"=w350:errorcluster)  [unwired: 11 in]
                        n1164 = call-poly <vilib>:"Append Image to Report.vi"("report in"=w348, "path or URL of image"=w339, "error in (no error)"=w350) -> ("report out"=w328:refnum<class "NI_report.lvclass">, "error out"=w330:errorcluster)  [unwired: 9 in, 2 out]
                        n1165 = call-dynamic "Set Report Margins.vi"("report in"=w328, "margins (1.00)"=T20 {"top"=0.1, "left"=0.1, "right"=0.1, "bottom"=0.1}, "error in (no error)"=w330) -> ("report out"=w327:refnum<class "NI_report.lvclass">, "error out"=w329:errorcluster)  [unwired: 10 in, 1 out]
                        n1166 = call "SelectPrinter.vi"() -> ("ChosenPrinter"=w344:string, "Closed?"=w343:bool)  [unwired: 2 in]
                        n1167 = case shown="False" w343 {
                          tunnel: w327 -> [w361 _]
                          tunnel: w344 -> [w359 _]
                          tunnel: w329 -> [w358 w362]
                          tunnel: [w356 w362] -> w341
                          frame False {
                            n1168 = call-dynamic "Print Report.vi"("report in"=w361, "printer name (default)"=w359, "error in (no error)"=w358) -> ("report out"=w360:refnum<class "NI_report.lvclass">, "error out"=w357:errorcluster)  [unwired: 11 in]
                            n1169 = call-dynamic "Dispose Report.vi"("report in"=w360, "error in (no error)"=w357) -> ("error out"=w356:errorcluster)  [unwired: 13 in]
                          }
                          frame True {
                          }
                        }
                        n1170 = Delete(path (use dialog)=w339, error in=w341) -> (error out=w340:errorcluster)  [unwired: 3 in, 2 out]
                      }
                    }
                  }
                  frame True {
                    # "Timeout/Error"
                  }
                }
                n1171 = local read "Quit"() -> (w319:bool)
                n1172 = global read "_Global Configuration.vi" "Quit"() -> (w318:bool)
                n1173 = Or(x=w318, y=w319) -> (x .or. y?=w317:bool)
              }
              n1174 = Release Queue(queue=w291, error in (no error)=w292) -> ()  [unwired: 1 in, 3 out]
            }
            frame #5 {
              n1175 = global read "_Global Configuration.vi" "Configuration 2"() -> (w1694:T18)
              n1176 = Release Queue(queue=w1700) -> ()  [unwired: 1 in, 4 out]
              n1177 = Unbundle By Name(w1694) -> ("Instrument"=w1693:string[])
              n1178 = Initialize Array("", 16 ("dimension size")) -> (w1691:string[])
              n1179 = Index Array(array=w1643, index #1=10 ("index"), index #5=1 ("index"), index #7=7 ("index")) -> (element #1=w1641:string, element #2=w1640:string, element #3=w1639:string, element #4=w1642:string, element #5=w1636:string, element #6=w1637:string, element #7=w1638:string)  [unwired: 4 in]
              n1180 = local read "LoadedTable"() -> (w1698:bool)
              n1181 = Replace Array Subset(array=w1691, new element=w1693, index=0) -> (w1687:string[])
              n1182 = Select(t="A new configuration table has been loaded.\n", s=w1698, f="") -> (s? t:f=w1673:string)
              n1183 = Index Array(array=w1687, index #1=10 ("index"), index #5=1 ("index"), index #7=7 ("index")) -> (element #1=w1682:string, element #2=w1681:string, element #3=w1680:string, element #4=w1683:string, element #5=w1665:string, element #6=w1664:string, element #7=w1653:string)  [unwired: 4 in]
              n1184 = Not Equal?(x=w1641, y=w1682) -> (x != y?=w1679:bool)
              n1185 = Not Equal?(x=w1642, y=w1683) -> (x != y?=w1684:bool)
              n1186 = Select(t="Pole orientation has been changed.\n", s=w1684, f="") -> (s? t:f=w1672:string)
              n1187 = Not Equal?(x=w1640, y=w1681) -> (x != y?=w1678:bool)
              n1188 = Not Equal?(x=w1639, y=w1680) -> (x != y?=w1677:bool)
              n1189 = Not Equal?(x=w1636, y=w1665) -> (x != y?=w1661:bool)
              n1190 = Not Equal?(x=w1637, y=w1664) -> (x != y?=w1658:bool)
              n1191 = Not Equal?(x=w1638, y=w1653) -> (x != y?=w1650:bool)
              n1192 = Compound Arithmetic op=OR(w1679, w1678, w1677) -> (w1674:bool)
              n1193 = Select(t="Oscillator settings have been changed.\n", s=w1674, f="") -> (s? t:f=w1671:string)
              n1194 = Select(t="Serial number has been changed.\n", s=w1661, f="") -> (s? t:f=w1657:string)
              n1195 = Select(t="Model name has been changed.\n", s=w1658, f="") -> (s? t:f=w1656:string)
              n1196 = Select(t="IP address has been changed.\n", s=w1650, f="") -> (s? t:f=w1649:string)
              n1197 = Unbundle By Name(w1646) -> ("CalAjusted"=w1645:bool)
              n1198 = Select(t="Calibration tables have been adjusted.\n", s=w1645, f="") -> (s? t:f=w1644:string)
              n1199 = Concatenate Strings(w1673, w1672, w1671, w1657, w1656, w1649, w1644) -> (w1669:string)
              n1200 = Empty String/Path?(string/path=w1669) -> (empty?=w1670:bool)
              n1201 = case shown="False" w1670 {
                tunnel: w1669 -> [w1702 _]
                tunnel: [w1701 _] -> w1668
                frame False {
                  n1202 = Format Into String(format string="Do you want to keep the following changes:\n\n%s\n(Press No to revert all changes)", w1702) -> (resulting string=w1707:string)  [unwired: 2 in, 1 out]
                  n1203 = call "_Log Events.vi"("Event"=w1702, "Log Command"=_Log_Command."Write" ("File Command")) -> ("error out"=w1701:errorcluster)  [unwired: 6 in, 1 out]
                  n1204 = Two Button Dialog(message=w1707, 1:"No" ("F button name (\"Cancel\")"), 2:"Yes" ("T button name (\"OK\")")) -> (T button?=w1704:bool)
                  n1205 = case shown="False" w1704 {
                    frame False {
                      n1206 = stacked-sequence {
                        frame #0 {
                          n1207 = call <vilib>:"Set Busy.vi"() -> ()  [unwired: 4 in, 8 out]
                        }
                        frame #1 {
                          n1208 = call "_Load All Tables.vi"("Use temporary file (F)"=TRUE) -> ()  [unwired: 7 out]
                        }
                        frame #2 {
                          n1209 = Wait (ms)(milliseconds to wait=u32 1800) -> ()  [unwired: 1 out]
                        }
                        frame #3 {
                          n1210 = call <vilib>:"Unset Busy.vi"() -> ()  [unwired: 2 in, 10 out]
                        }
                      }
                    }
                    frame True {
                    }
                  }
                }
                frame True {
                }
              }
              n1211 = call "_Log Events.vi"("error in (no error)"=w1668, "Log Command"=_Log_Command."Close" ("File Command")) -> ()  [unwired: 6 in, 2 out]
            }
            frame #6 {
              w1722 = "Lens" ("section")
              n1212 = call "_Open Preference File.vi"() -> ("error"=w1731:errorcluster, "refnum"=w1732:T29)  [unwired: 3 in, 3 out]
              n1213 = local read "Oscillator Settings"() -> (w1717:string[][])
              n1214 = local read "IP Address"() -> (w1726:string)
              n1215 = global read "_Global LC Driver.vi" "LC Type"() -> (w1733:T30)
              n1216 = call-poly <vilib>:"Write Key.vi"("section"=w1722, "error in (no error)"=w1731, "value"=w1733, "key"="LCType" ("section"), "refnum"=w1732) -> ("error out"=w1727:errorcluster, "refnum out"=w1728:T29)  [unwired: 5 out]
              n1217 = call "_Save All Tables.vi"("SaveOption (Temporary File)"=T16."My Tables" ("Use temporary file (F)")) -> ()  [unwired: 2 in, 5 out]
              n1218 = call-poly <vilib>:"Write Key.vi"("section"=w1722, "error in (no error)"=w1727, "value"=w1726, "key"="UpsIP" ("section"), "refnum"=w1728) -> ("error out"=w1725:errorcluster, "refnum out"=w1729:T29)  [unwired: 1 in, 4 out]
              n1219 = Index Array(array=w1717, index (col) #1=2 ("index (row)"), index (col) #2=3 ("index (row)"), index (col) #3=4 ("index (row)"), index (col) #4=5 ("index (row)")) -> (element #1=w1715:string[], element #2=w1714:string[], element #3=w1713:string[], element #4=w1712:string[])  [unwired: 4 in]
              n1220 = Build Array(w1715, w1714, w1713, w1712) -> (w1711:string[][])
              n1221 = for {
                shift-right: [w1746] -> w1724
                shift-left: w1725 -> [w1751]
                shift-right: [w1744] -> w1723
                shift-left: w1729 -> [w1750]
                tunnel: string[] ["RefClk", "ClkMult", "ScaleF", "FreqOut"] -> [w1740] mode=indexing
                tunnel: w1711 -> [w1739] mode=indexing
                n1222 = Index Array(array=w1739) -> (element #1=w1738:string, element #2=w1737:string, element #3=w1736:string)  [unwired: 3 in]
                n1223 = call-poly <vilib>:"Write Key.vi"("section"="Oscillator0" ("key"), "error in (no error)"=w1751, "value"=w1738, "key"=w1740, "refnum"=w1750) -> ("error out"=w1749:errorcluster, "refnum out"=w1747:T29)  [unwired: 4 in, 1 out]
                n1224 = call-poly <vilib>:"Write Key.vi"("section"="Oscillator1" ("key"), "error in (no error)"=w1749, "value"=w1737, "key"=w1740, "refnum"=w1747) -> ("error out"=w1748:errorcluster, "refnum out"=w1745:T29)  [unwired: 4 in, 1 out]
                n1225 = call-poly <vilib>:"Write Key.vi"("section"="Oscillator2" ("key"), "error in (no error)"=w1748, "value"=w1736, "key"=w1740, "refnum"=w1745) -> ("error out"=w1746:errorcluster, "refnum out"=w1744:T29)  [unwired: 4 in, 1 out]
              }
              n1226 = call <vilib>:"Close Config Data.vi"("error in (no error)"=w1724, "refnum"=w1723) -> ()  [unwired: 1 in, 9 out]
            }
            frame #7 {
              n1227 = call "_Remote Communicate.vi"("DC Param"=u16 1, "Command"=_RT_Command."Ignore Error") -> ()  [unwired: 4 in, 4 out]
              n1228 = call "_Copy IPF Files.vi"() -> ()  [unwired: 1 out]
            }
          }
        }
      }
    }
    frame #1 {
      # "Hidden Controls Include:\n1. VoltageInput\n2. LoadedTable\n3. Running\n4. Quit\n5. Tune File\n6. SG Input"
      n1229 = case shown="False" w1754 {
        frame False {
          w1755 = TRUE  # release?
          n1230 = Quit LabVIEW(quit? (T)=w1755) -> ()
        }
        frame True {
        }
      }
    }
  }
  n1231 = property class="VI"(reference=w1, "Front Panel.Title"=w2) -> ()  [unwired: 1 in, 2 out]
  "Version" <- w2
